vi "CRYO_MASTER_FULL_RUN4_dev2.vi"() -> ()   [LabVIEW 2017]
uses:
  LSI218Data.lvclass
  LSI336Data.lvclass
  USBData.lvclass
  6240AData.lvclass
  DMMsData.lvclass
  LMData.lvclass
  <vilib>/DAQmx/miscellaneous.llb/DAQmx Fill In Error Info.vi
  <vilib>/DAQmx/create/channels.llb/DAQmx Create Channel (DO-Digital Output).vi
  <vilib>/DAQmx/create/channels.llb/DAQmx Create Channel (AO-Voltage-Basic).vi
  <vilib>/express/express arith-compare/Formula/XNode/ExpressFormulaBlockNode.xnode
  <vilib>/Analysis/NI_AALBase.lvlib
  istr.lib/Agilent 33XXX Series/Agilent 33XXX Series.lvlib
panel:
  out "Error Out (AZDAX status)":errorcluster
  in  "Automatic \nScreenshots?":bool=TRUE
  in  "Frontpanel screenshots":bool
  in  "Screenshots interval":i64=3605
  in  "Record interval":i64=20
  out "Cycle #":u32=2
  in  "Measurement Interval (s)":dbl=1.0
  in  "Stop Button":bool
  in  "?":T1(tab)=enum."VALVE/HEATER CTRL"
  out "RUN Identifier":string="20210323_164300_RUNIV"
  in  "Base Path (screenshots)":path=path "C:/LabVIEW/DATA/Google/TUCAN Experiments/KEK_cryotests_2019-2020/data/screenshots"
  out "error out (USB6210/6218 AOUT)":errorcluster
  in  "AOUT Labels":string[](array[string])=["PWR400H_I", "PMC183A_I"]
  in  "AOUT assignment":tag[](array[tag])=["Dev1/ao0", "Dev1/ao1"]
  out "AO task out":refnum<k21>="20210323_164300_RUNIV_AO"
  in  "Analog Out ON?":bool=TRUE
  in  "DOUT6218 Labels":string[](array[string])=["D_V1_NO", "D_V2_NC", "D_CV1", "D_H1", "D_HOME", "D_STOP", "D_M0", "D_M1"]
  in  "InstName (USB6218)":string="USB6218"
  in  "USB6218 Config":T2(array[cluster])=[{"Label"="F_1", "FileFormat"="%5.5f", "Active?"=TRUE, "Physical CH"="Dev1/ai0", " terminal\n type"=10083, "ConversionType"={"Type"=enum."SimpleProp", "ConversionParameters"=[0.0, 5.0, 0.0, 500.0]}, "VoltageLimits"=[0.0, 5.0]}, {"Label"="F_2", "FileFormat"="%5.5f", "Active?"=TRUE, "Physical CH"="Dev1/ai1", " terminal\n type"=10083, "ConversionType"={"Type"=enum."SimpleProp", "ConversionParameters"=[0.0, 5.0, 0.0, 200.0]}, "VoltageLimits"=[0.0, 5.0]}, {"Label"="F_3", "FileFormat"="%5.5f", "Active?"=TRUE, "Physical CH"="Dev1/ai2", " terminal\n type"=10083, "ConversionType"={"Type"=enum."SimpleProp", "ConversionParameters"=[0.0, 5.0, 0.0, 200.0]}, "VoltageLimits"=[0.0, 5.0]}, {"Label"="F_4", "FileFormat"="%5.5f", "Active?"=TRUE, "Physical CH"="Dev1/ai3", " terminal\n type"=10083, "ConversionType"={"Type"=enum."SimpleProp", "ConversionParameters"=[0.0, 5.0, 0.0, 500.0]}, "VoltageLimits"=[0.0, 5.0]}, {"Label"="F_5", "FileFormat"="%5.5f", "Active?"=TRUE, "Physical CH"="Dev1/ai4", " terminal\n type"=10083, "ConversionType"={"Type"=enum."SimpleProp", "ConversionParameters"=[0.0, 5.0, 0.0, 500.0]}, "VoltageLimits"=[0.0, 5.0]}, {"Label"="I_CV", "FileFormat"="%3.5f", "Active?"=TRUE, "Physical CH"="Dev1/ai5", " terminal\n type"=10083, "ConversionType"={"Type"=enum."Raw", "ConversionParameters"=[0.0, 0.0, 0.0, 0.0]}, "VoltageLimits"=[0.0, 10.0]}, {"Label"="CV1_answer", "FileFormat"="%3.5f", "Active?"=TRUE, "Physical CH"="Dev1/ai6", " terminal\n type"=10083, "ConversionType"={"Type"=enum."SimpleProp", "ConversionParameters"=[1.0, 5.0, 0.0, 100.0]}, "VoltageLimits"=[0.0, 5.0]}, {"Label"="P_Dewar", "FileFormat"="%5.5e", "Active?"=TRUE, "Physical CH"="Dev1/ai7", " terminal\n type"=10083, "ConversionType"={"Type"=enum."SimpleProp", "ConversionParameters"=[1.0, 5.0, 0.0, 200000.0]}, "VoltageLimits"=[0.0, 5.0]}, {"Label"="L_Dewar", "FileFormat"="%5.5f", "Active?"=TRUE, "Physical CH"="Dev1/ai8", " terminal\n type"=10083, "ConversionType"={"Type"=enum."SimpleProp", "ConversionParameters"=[0.0, 10.0, 0.0, 100.0]}, "VoltageLimits"=[0.0, 10.0]}] {"terminal\n type" items=["Default"=-1, "RSE"=10083, "NRSE"=10078, "Differential"=10106, "Pseudodifferential"=12529]}
  out "error out (USB6218)":errorcluster
  out "error out (USB6210/6218 DOUT)":errorcluster
  out "DOUT task out":refnum<k21>="20210323_164301_DO"
  in  "DOUT Physical CH":tag[](array[tag])=["Dev1/port1/line0", "Dev1/port1/line1", "Dev1/port1/line2", "Dev1/port1/line3", "Dev1/port1/line4", "Dev1/port1/line5", "Dev1/port1/line6", "Dev1/port1/line7"]
  in  "Digital Out ON?":bool=TRUE
  in  "USB6210 Config":T2(array[cluster])=[{"Label"="P_ins", "FileFormat"="%5.5e", "Active?"=TRUE, "Physical CH"="Dev2/ai0", " terminal\n type"=10083, "ConversionType"={"Type"=enum."CC-10_LOG", "ConversionParameters"=[0.5, 9.0, 0.0, 1.0]}, "VoltageLimits"=[0.0, 10.0]}, {"Label"="P_4Kres", "FileFormat"="%5.5e", "Active?"=TRUE, "Physical CH"="Dev2/ai1", " terminal\n type"=10083, "ConversionType"={"Type"=enum."SimpleProp", "ConversionParameters"=[1.0, 5.0, 0.0, 200000.0]}, "VoltageLimits"=[0.0, 5.0]}, {"Label"="P_3HeIN", "FileFormat"="%5.5e", "Active?"=TRUE, "Physical CH"="Dev2/ai2", " terminal\n type"=10083, "ConversionType"={"Type"=enum."SimpleProp", "ConversionParameters"=[1.0, 5.0, 0.0, 200000.0]}, "VoltageLimits"=[0.0, 5.0]}, {"Label"="P_SldRTN", "FileFormat"="%5.5e", "Active?"=TRUE, "Physical CH"="Dev2/ai3", " terminal\n type"=10083, "ConversionType"={"Type"=enum."SimpleProp", "ConversionParameters"=[1.0, 5.0, 0.0, 200000.0]}, "VoltageLimits"=[0.0, 5.0]}, {"Label"="P_3Hepot", "FileFormat"="%5.5e", "Active?"=TRUE, "Physical CH"="Dev2/ai4", " terminal\n type"=10083, "ConversionType"={"Type"=enum."SimpleProp", "ConversionParameters"=[0.0, 10.0, 0.0, 133320.0]}, "VoltageLimits"=[0.0, 10.0]}, {"Label"="P_1Kpot", "FileFormat"="%5.5e", "Active?"=TRUE, "Physical CH"="Dev2/ai5", " terminal\n type"=10083, "ConversionType"={"Type"=enum."SimpleProp", "ConversionParameters"=[0.0, 10.0, 0.0, 133320.0]}, "VoltageLimits"=[0.0, 10.0]}, {"Label"="P_Dewar(old)", "FileFormat"="%5.5e", "Active?"=FALSE, "Physical CH"="Dev2/ai6", " terminal\n type"=10083, "ConversionType"={"Type"=enum."SimpleProp", "ConversionParameters"=[1.0, 5.0, 0.0, 200000.0]}, "VoltageLimits"=[0.0, 5.0]}, {"Label"="DP_HEX4", "FileFormat"="%5.5e", "Active?"=TRUE, "Physical CH"="Dev2/ai7", " terminal\n type"=10083, "ConversionType"={"Type"=enum."SimpleProp", "ConversionParameters"=[1.0, 5.0, 0.0, 1000.0]}, "VoltageLimits"=[0.0, 5.0]}, {"Label"="DP_HEX5", "FileFormat"="%5.5e", "Active?"=TRUE, "Physical CH"="Dev2/ai8", " terminal\n type"=10083, "ConversionType"={"Type"=enum."SimpleProp", "ConversionParameters"=[1.0, 5.0, 0.0, 1000.0]}, "VoltageLimits"=[0.0, 5.0]}, {"Label"="L1(old)", "FileFormat"="%5.5f", "Active?"=TRUE, "Physical CH"="Dev2/ai9", " terminal\n type"=10083, "ConversionType"={"Type"=enum."SimpleProp", "ConversionParameters"=[0.0, 10.0, 0.0, 100.0]}, "VoltageLimits"=[0.0, 10.0]}, {"Label"="L2-1", "FileFormat"="%5.5f", "Active?"=TRUE, "Physical CH"="Dev2/ai10", " terminal\n type"=10083, "ConversionType"={"Type"=enum."SimpleProp", "ConversionParameters"=[0.0, 10.0, 0.0, 100.0]}, "VoltageLimits"=[0.0, 10.0]}, {"Label"="L1", "FileFormat"="%5.5f", "Active?"=TRUE, "Physical CH"="Dev2/ai11", " terminal\n type"=10083, "ConversionType"={"Type"=enum."SimpleProp", "ConversionParameters"=[0.0, 10.0, 0.0, 100.0]}, "VoltageLimits"=[0.0, 10.0]}, {"Label"="L3", "FileFormat"="%5.5f", "Active?"=TRUE, "Physical CH"="Dev2/ai12", " terminal\n type"=10083, "ConversionType"={"Type"=enum."SimpleProp", "ConversionParameters"=[0.0, 10.0, 0.0, 100.0]}, "VoltageLimits"=[0.0, 10.0]}, {"Label"="P_HEX7OUT", "FileFormat"="%5.5e", "Active?"=TRUE, "Physical CH"="Dev2/ai13", " terminal\n type"=10083, "ConversionType"={"Type"=enum."SimpleProp", "ConversionParameters"=[1.0, 5.0, 0.0, 200000.0]}, "VoltageLimits"=[0.0, 5.0]}, {"Label"="P_IP", "FileFormat"="%5.5e", "Active?"=TRUE, "Physical CH"="Dev2/ai14", " terminal\n type"=10083, "ConversionType"={"Type"=enum."CC-10_LOG", "ConversionParameters"=[0.5, 9.0, 0.0, 1.0]}, "VoltageLimits"=[0.0, 10.0]}, {"Label"="V_H1", "FileFormat"="%3.5f", "Active?"=TRUE, "Physical CH"="Dev2/ai15", " terminal\n type"=10083, "ConversionType"={"Type"=enum."Raw", "ConversionParameters"=[0.0, 1.0, 0.0, 1.0]}, "VoltageLimits"=[0.0, 10.0]}] {"terminal\n type" items=["Default"=-1, "RSE"=10083, "NRSE"=10078, "Differential"=10106, "Pseudodifferential"=12529]}
  in  "RUN label":string="RUNIV"
  in  "Base Path":path=path "C:/LabVIEW/DATA/RUN_4"
  in  "InstName (USB6210)":string="USB6210"
  out "error out (USB6210)":errorcluster
  out "File Refn USB AO":refnum<file>
  out "File Refn USB DO":refnum<file>
  out "File ref AZD-AX status":refnum<file>
  in  "LM measurement interval (>0)":i64=10
  in  "Active? (HP34401 LM)":bool=TRUE
  in  "Labels (HP34401 LM)":string[](array[string])=["R_L2-2", "L2-2"]
  in  "FileFormat (HP34401 LM)":string[](array[string])=["%.4f", "%.4f"]
  in  "VISA (HP34401 LM)":refnum<visa-resource-name>="GPIB0::24::INSTR"
  in  "LevelCalibration (R0, R1, L0, L1)":dbl[](array[numeric])=[186.541, 0.0, 0.0, 100.0]
  in  "InstName (HP34401 LM)":string="HP34401LM"
  out "error out (LSI336)":errorcluster
  in  "InstName (LSI336)":string="LSI336"
  in  "FileFormat (336)":string="%4.4f"
  in  "LSI336Settings(X,Y)":T3(array[cluster])=[{"LSIName"="LSi336X", "Labels"=["T1K3-1", "T1K3-2", "T3He5", "T3He8"], "SensorLocations"=[enum."T1K3-1", enum."T1K3-2", enum."T3He5", enum."T3He8"], "Active?"=TRUE, "VISA res. name"="COM15_LSI336Y"}, {"LSIName"="LSi336Y", "Labels"=["T3He6-1", "T3He6-2", "T3He7-1", "T3He7-2"], "SensorLocations"=[enum."T3He6-1", enum."T3He6-2", enum."T3He7-1", enum."T3He7-2"], "Active?"=TRUE, "VISA res. name"="COM20_LSI336X"}]
  in  "FileFormat (218)":string="%4.4f"
  in  "InstName (LSI218)":string="LSI218"
  in  "LSI218Settings(A-F)":T3(array[cluster])=[{"LSIName"="LSI218A", "Labels"=["T3He10", "T3He1-1", "TTH3", "TTH4", "TTH1", "TTH2", "T4He1", "T1K1"], "SensorLocations"=[enum."T3He10", enum."T3He1-1", enum."TTH3", enum."TTH4", enum."TTH1", enum."TTH2", enum."T4He1", enum."T1K1"], "Active?"=TRUE, "VISA res. name"="GPIB0::7::INSTR"}, {"LSIName"="LSI218B", "Labels"=["N.C.", "N.C.", "N.C.", "N.C.", "T3He2-1", "T3He2-2", "T3He3", "T3He1-4"], "SensorLocations"=[enum."N.C.", enum."N.C.", enum."N.C.", enum."N.C.", enum."T3He2-1", enum."T3He2-2", enum."T3He3", enum."T3He1-4"], "Active?"=TRUE, "VISA res. name"="GPIB0::4::INSTR"}, {"LSIName"="LSI218C", "Labels"=["T4He3-1", "T4He3-2", "T4He3-3", "T4He3-4", "T4He2-1", "T4He2-2", "T4He4", "T4He5"], "SensorLocations"=[enum."T4He3-1", enum."T4He3-2", enum."T4He3-3", enum."T4He3-4", enum."T4He2-1", enum."T4He2-2", enum."T4He4", enum."T4He5"], "Active?"=TRUE, "VISA res. name"="GPIB0::3::INSTR"}, {"LSIName"="LSI218D", "Labels"=["T4He6", "T4He9", "T3He1-2", "T3He1-3", "T4He7", "T4He8", "T4He10", "T1K6"], "SensorLocations"=[enum."T4He6", enum."T4He9", enum."T3He1-2", enum."T3He1-3", enum."T4He7", enum."T4He8", enum."T4He10", enum."T1K6"], "Active?"=TRUE, "VISA res. name"="GPIB0::5::INSTR"}, {"LSIName"="LSI218E", "Labels"=["TIP1", "N.C.", "TIP2", "N.C.", "TIP3", "TIP4", "TIP5", "N.C."], "SensorLocations"=[enum."TIP1", enum."N.C.", enum."TIP2", enum."N.C.", enum."TIP3", enum."TIP4", enum."TIP5", enum."N.C."], "Active?"=TRUE, "VISA res. name"="GPIB0::11::INSTR"}, {"LSIName"="LSI218F", "Labels"=["T1K2", "T1K4", "T1K5", "T3He4", "T3He9", "TIP6", "N.C.", "N.C."], "SensorLocations"=[enum."T1K2", enum."T1K4", enum."T1K5", enum."T3He4", enum."T3He9", enum."TIP6", enum."N.C.", enum."N.C."], "Active?"=TRUE, "VISA res. name"="GPIB0::8::INSTR"}]
  out "error out (LSI218)":errorcluster
  out "RUN Identifier 2":string="20210323_164300_RUNIV" caption="RUN Identifier"
  out "error out (HP34401 LM)":errorcluster
  out "Graph 3":T4(graph)=[{"TimeArray"=[timestamp(3699330182.9543066 s since 1904-01-01), timestamp(3699330183.99275 s since 1904-01-01)], "DataArray"=[2.229000287561577, 1.8476051977193715]}, {"TimeArray"=[timestamp(3699330182.9543066 s since 1904-01-01), timestamp(3699330183.99275 s since 1904-01-01)], "DataArray"=[6.5651805759101745, 6.559919954343005]}, {"TimeArray"=[timestamp(3699330182.9543066 s since 1904-01-01), timestamp(3699330183.99275 s since 1904-01-01)], "DataArray"=[0.6141023076914145, 0.5720173311260397]}, {"TimeArray"=[timestamp(3699330182.9543066 s since 1904-01-01), timestamp(3699330183.99275 s since 1904-01-01)], "DataArray"=[-0.3684318274206404, -0.35856816207260195]}, {"TimeArray"=[timestamp(3699330182.9543066 s since 1904-01-01), timestamp(3699330183.99275 s since 1904-01-01)], "DataArray"=[23.39313821847484, 23.485199087329573]}, {"TimeArray"=[timestamp(3699330182.9543066 s since 1904-01-01), timestamp(3699330183.99275 s since 1904-01-01)], "DataArray"=[-0.0038120682713622734, -0.00019463958134809388]}] caption="XY Graph"
  out "Graph 1":T4(graph)=[{"TimeArray"=[timestamp(3699330182.9503174 s since 1904-01-01), timestamp(3699330183.988761 s since 1904-01-01)], "DataArray"=[0.0001467822274904493, 0.00014331210383532943]}, {"TimeArray"=[timestamp(3699330182.9503174 s since 1904-01-01), timestamp(3699330183.988761 s since 1904-01-01)], "DataArray"=[103386.1520739023, 103419.04061540413]}, {"TimeArray"=[timestamp(3699330182.9503174 s since 1904-01-01), timestamp(3699330183.988761 s since 1904-01-01)], "DataArray"=[102917.4903816534, 102917.49038025808]}, {"TimeArray"=[timestamp(3699330182.9503174 s since 1904-01-01), timestamp(3699330183.988761 s since 1904-01-01)], "DataArray"=[102784.29179605731, 102876.37970352173]}, {"TimeArray"=[timestamp(3699330182.9503174 s since 1904-01-01), timestamp(3699330183.988761 s since 1904-01-01)], "DataArray"=[102285.6157171335, 102299.64398756107]}, {"TimeArray"=[timestamp(3699330182.9503174 s since 1904-01-01), timestamp(3699330183.988761 s since 1904-01-01)], "DataArray"=[102778.35876990847, 102783.61937258235]}, {"TimeArray"=[timestamp(3699330182.9503174 s since 1904-01-01), timestamp(3699330183.988761 s since 1904-01-01)], "DataArray"=[0.0, 0.0]}, {"TimeArray"=[timestamp(3699330182.9503174 s since 1904-01-01), timestamp(3699330183.988761 s since 1904-01-01)], "DataArray"=[102831.98017524344, 102960.24547937719]}, {"TimeArray"=[timestamp(3699330182.9503174 s since 1904-01-01), timestamp(3699330183.988761 s since 1904-01-01)], "DataArray"=[6.658695577811817e-05, 6.903046749339257e-05]}, {"TimeArray"=[timestamp(3699330182.9543066 s since 1904-01-01), timestamp(3699330183.99275 s since 1904-01-01)], "DataArray"=[133922.54729625225, 134754.38150670484]}] caption="XY Graph"
  in  "FIle suffix 4":string="Graph4_noise"
  in  "Take Screenshot! 4":bool
  in  "Take Screenshot! 3":bool
  in  "Take Screenshot! 2":bool
  in  "Take Screenshot! 1":bool
  in  "FIle suffix 3":string="Graph3_noise"
  in  "FIle suffix 2":string="Graph2_build"
  in  "FIle suffix 1":string="Graph1_noise"
  in  "log/linear 2":bool
  in  "Tab Control 2":T5(tab)=enum."Temperature (3)"
  in  "Plot selecter (USB6210)\n    1      2     3     4":bool[][](array[boolean])=[[TRUE, FALSE, FALSE, FALSE], [TRUE, FALSE, FALSE, FALSE], [TRUE, FALSE, FALSE, FALSE], [TRUE, FALSE, FALSE, FALSE], [TRUE, FALSE, FALSE, FALSE], [TRUE, FALSE, FALSE, FALSE], [TRUE, FALSE, FALSE, FALSE], [FALSE, FALSE, FALSE, FALSE], [FALSE, FALSE, FALSE, FALSE], [FALSE, TRUE, FALSE, FALSE], [FALSE, TRUE, FALSE, FALSE], [FALSE, TRUE, FALSE, FALSE], [FALSE, TRUE, FALSE, FALSE], [TRUE, FALSE, FALSE, FALSE], [TRUE, FALSE, FALSE, FALSE], [FALSE, FALSE, FALSE, FALSE]]
  out "All Labels (USB6210)":string[](array[string])=["P_ins", "P_4Kres", "P_3HeIN", "P_SldRTN", "P_3Hepot", "P_1Kpot", "P_Dewar(old)", "DP_HEX4", "DP_HEX5", "L1(old)", "L2-1", "L1", "L3", "P_HEX7OUT", "P_IP", "V_H1"]
  out "Last Data \n(USB6210)":dbl[](array[numeric])=[0.00014331210383532943, 103419.04061540413, 102917.49038025808, 102876.37970352173, 102299.64398756107, 102783.61937258235, 0.0, 0.009359860621893645, 6.307429085038785, 9.980910378649359, 0.03893370650245273, 0.17703499365619763, 31.866703704233657, 102960.24547937719, 6.903046749339257e-05, 5.354612085872782] format="%#_6e"
  out "Time of Last Measurement (USB6210)":timestamp=timestamp(3699330183.988761 s since 1904-01-01)
  out "USB6210 Status":T6(ring)=enum."Ready"
  out "Last Vol\n(USB6210)":dbl[](array[numeric])=[5.578141435767079, 3.0683808123080825, 3.0583498076051616, 3.0575275940704345, 7.673240623129393, 7.709542407184395, 0.0, 1.0000374394424876, 1.0252297163401551, 0.9980910378649359, 0.003893370650245273, 0.01770349936561976, 3.1866703704233657, 3.0592049095875438, 5.419520407280226, 5.354612085872782] format="%_5f"
  out "Labels (HP34401 LM) 2":string[](array[string])=["R_L2-2", "L2-2"]
  out "LastData (HP34401 LM)":dbl[](array[numeric])
  in  "Plot selecter (HP34401A)\n    1      2     3     4":bool[][](array[boolean])=[[FALSE, TRUE, FALSE, FALSE], [FALSE, TRUE, FALSE, FALSE], [TRUE, FALSE, FALSE, FALSE], [TRUE, FALSE, FALSE, FALSE], [TRUE, FALSE, FALSE, FALSE], [TRUE, FALSE, FALSE, FALSE], [TRUE, FALSE, FALSE, FALSE], [FALSE, TRUE, FALSE, FALSE], [FALSE, TRUE, FALSE, FALSE], [FALSE, TRUE, FALSE, FALSE], [FALSE, TRUE, FALSE, FALSE], [FALSE, TRUE, FALSE, FALSE], [FALSE, TRUE, FALSE, FALSE], [TRUE, FALSE, FALSE, FALSE], [TRUE, FALSE, FALSE, FALSE], [FALSE, FALSE, FALSE, FALSE]]
  out "Time of Last Measurement (USB6218)":timestamp=timestamp(3699330183.99275 s since 1904-01-01)
  out "USB6218 Status":T6(ring)=enum."Ready"
  out "Last Vol \n(USB6218)":dbl[](array[numeric])=[0.018476051977193715, 0.16399799885857513, 0.014300433278150993, -0.0035856816207260195, 0.23485199087329572, -0.00019463958134809388, 0.003022974846202206, 3.695087630134097, 1.4212571383113937] format="%_5f"
  out "Last Data \n(USB6218)":dbl[](array[numeric])=[1.8476051977193715, 6.559919954343005, 0.5720173311260397, -0.35856816207260195, 23.485199087329573, -0.00019463958134809388, -24.924425628844947, 134754.38150670484, 14.212571383113936] format="%#_6e"
  out "All Labels (USB6218)":string[](array[string])=["F_1", "F_2", "F_3", "F_4", "F_5", "I_CV", "CV1_answer", "P_Dewar", "L_Dewar"]
  in  "Plot selecter (USB6218)\n    1      2     3     4":bool[][](array[boolean])=[[FALSE, FALSE, TRUE, FALSE], [FALSE, FALSE, TRUE, FALSE], [FALSE, FALSE, TRUE, FALSE], [FALSE, FALSE, TRUE, FALSE], [FALSE, FALSE, TRUE, FALSE], [FALSE, FALSE, TRUE, FALSE], [FALSE, FALSE, FALSE, FALSE], [TRUE, FALSE, FALSE, FALSE], [FALSE, TRUE, FALSE, FALSE], [FALSE, FALSE, FALSE, TRUE], [FALSE, FALSE, FALSE, TRUE], [FALSE, FALSE, FALSE, TRUE], [FALSE, FALSE, FALSE, TRUE], [FALSE, FALSE, FALSE, FALSE], [FALSE, FALSE, FALSE, FALSE], [FALSE, FALSE, FALSE, FALSE]]
  out "Time of Last Measurement (LSI218)":timestamp=timestamp(3699330183.988761 s since 1904-01-01)
  out "LSI218 Status":T7(ring)=enum."Measuring"
  out "Last Data \nLSI218 (1)":dbl[](array[numeric])=[238.58, 276.68, 145.02, 218.62, 54.478, 85.05, 4.442, 4.661, 30.0, 0.0, 0.0, 0.0, 56.991, 53.134, 5.055, 271.93, 282.27, 282.4, 279.79, 279.75, 34.466, 36.266, 28.98, 55.8]
  out "Labels LSI218 (1)":string[](array[string])=["T3He10", "T3He1-1", "TTH3", "TTH4", "TTH1", "TTH2", "T4He1", "T1K1", "N.C.", "N.C.", "N.C.", "N.C.", "T3He2-1", "T3He2-2", "T3He3", "T3He1-4", "T4He3-1", "T4He3-2", "T4He3-3", "T4He3-4", "T4He2-1", "T4He2-2", "T4He4", "T4He5"]
  in  "Plot selecter LSI218(1)\n    1      2     3     4":bool[][](array[boolean])=[[FALSE, FALSE, FALSE, TRUE], [FALSE, FALSE, FALSE, TRUE], [FALSE, FALSE, FALSE, TRUE], [FALSE, FALSE, FALSE, TRUE], [FALSE, FALSE, FALSE, TRUE], [FALSE, FALSE, FALSE, TRUE], [FALSE, FALSE, FALSE, TRUE], [FALSE, FALSE, FALSE, TRUE], [FALSE, FALSE, FALSE, FALSE], [FALSE, FALSE, FALSE, FALSE], [FALSE, FALSE, FALSE, FALSE], [FALSE, FALSE, FALSE, FALSE], [FALSE, FALSE, FALSE, TRUE], [FALSE, FALSE, FALSE, TRUE], [FALSE, FALSE, FALSE, TRUE], [FALSE, FALSE, FALSE, TRUE], [FALSE, FALSE, FALSE, TRUE], [FALSE, FALSE, FALSE, TRUE], [FALSE, FALSE, FALSE, TRUE], [FALSE, FALSE, FALSE, TRUE], [FALSE, FALSE, FALSE, TRUE], [FALSE, FALSE, FALSE, TRUE], [FALSE, FALSE, FALSE, TRUE], [FALSE, FALSE, FALSE, TRUE]]
  out "Active?\n (1)":bool[](array[boolean])=[TRUE, TRUE, TRUE, TRUE, TRUE, TRUE, TRUE, TRUE, TRUE, TRUE, TRUE, TRUE, TRUE, TRUE, TRUE, TRUE, TRUE, TRUE, TRUE, TRUE, TRUE, TRUE, TRUE, TRUE]
  out "Labels LSI218 (2)":string[](array[string])=["T4He6", "T4He9", "T3He1-2", "T3He1-3", "T4He7", "T4He8", "T4He10", "T1K6", "TIP1", "N.C.", "TIP2", "N.C.", "TIP3", "TIP4", "TIP5", "N.C.", "T1K2", "T1K4", "T1K5", "T3He4", "T3He9", "TIP6", "N.C.", "N.C."]
  out "Active?\n(2)":bool[](array[boolean])=[TRUE, TRUE, TRUE, TRUE, TRUE, TRUE, TRUE, TRUE, TRUE, TRUE, TRUE, TRUE, TRUE, TRUE, TRUE, TRUE, TRUE, TRUE, TRUE, TRUE, TRUE, TRUE, TRUE, TRUE]
  out "Last Data \nLSI218 (2)":dbl[](array[numeric])=[62.643, 171.21, 276.82, 272.08, 143.05, 161.51, 221.22, 243.0, 252.76, 0.0, 130.11, 688.49, 83.786, 70.623, 114.8, 688.58, 14.054, 11.753, 10.988, 12.938, 10.918, 110.83, 0.433, 0.0]
  in  "Plot selecter LSI218(2)\n    1      2     3     4":bool[][](array[boolean])=[[FALSE, FALSE, FALSE, TRUE], [FALSE, FALSE, FALSE, TRUE], [FALSE, FALSE, FALSE, FALSE], [FALSE, FALSE, FALSE, FALSE], [FALSE, FALSE, FALSE, FALSE], [FALSE, FALSE, FALSE, FALSE], [FALSE, FALSE, FALSE, FALSE], [FALSE, FALSE, FALSE, FALSE], [FALSE, FALSE, FALSE, FALSE], [FALSE, FALSE, FALSE, FALSE], [FALSE, FALSE, FALSE, FALSE], [FALSE, FALSE, FALSE, FALSE], [FALSE, FALSE, FALSE, FALSE], [FALSE, FALSE, FALSE, FALSE], [FALSE, FALSE, FALSE, FALSE], [FALSE, FALSE, FALSE, FALSE], [FALSE, FALSE, FALSE, TRUE], [FALSE, FALSE, FALSE, TRUE], [FALSE, FALSE, FALSE, TRUE], [FALSE, FALSE, FALSE, TRUE], [FALSE, FALSE, FALSE, TRUE], [FALSE, FALSE, FALSE, FALSE], [FALSE, FALSE, FALSE, FALSE], [FALSE, FALSE, FALSE, FALSE]]
  in  "Plot selecter LSI336 \n     1      2     3     4":bool[][](array[boolean])=[[FALSE, FALSE, FALSE, TRUE], [FALSE, FALSE, FALSE, TRUE], [FALSE, FALSE, FALSE, TRUE], [FALSE, FALSE, FALSE, TRUE], [FALSE, FALSE, FALSE, TRUE], [FALSE, FALSE, FALSE, TRUE], [FALSE, FALSE, FALSE, TRUE], [FALSE, FALSE, FALSE, TRUE]]
  out "Time of Last Measurement (LSI336)":timestamp=timestamp(3699330183.988761 s since 1904-01-01)
  out "Last Data \nLSI336":dbl[](array[numeric])=[12.0158, 12.046, 13.2196, 12.3577, 19.0262, 19.857, 21.3351, 16.3982]
  out "Active?\n(LSI336)":bool[](array[boolean])=[TRUE, TRUE, TRUE, TRUE, TRUE, TRUE, TRUE, TRUE]
  out "Labels LSI336":string[](array[string])=["T1K3-1", "T1K3-2", "T3He5", "T3He8", "T3He6-1", "T3He6-2", "T3He7-1", "T3He7-2"]
  out "LSI336 Status":T7(ring)=enum."Measuring"
  in  "log/linear 1":bool
  out "Graph 2":T4(graph)=[{"TimeArray"=[timestamp(3699330182.9503174 s since 1904-01-01), timestamp(3699330183.988761 s since 1904-01-01)], "DataArray"=[10.022340765034453, 9.980910378649359]}, {"TimeArray"=[timestamp(3699330182.9503174 s since 1904-01-01), timestamp(3699330183.988761 s since 1904-01-01)], "DataArray"=[0.028411703634074498, 0.03893370650245273]}, {"TimeArray"=[timestamp(3699330182.9503174 s since 1904-01-01), timestamp(3699330183.988761 s since 1904-01-01)], "DataArray"=[0.17703499366301226, 0.17703499365619763]}, {"TimeArray"=[timestamp(3699330182.9503174 s since 1904-01-01), timestamp(3699330183.988761 s since 1904-01-01)], "DataArray"=[31.87854099600237, 31.866703704233657]}, {"TimeArray"=[timestamp(3699330182.9543066 s since 1904-01-01), timestamp(3699330183.99275 s since 1904-01-01)], "DataArray"=[14.198759390010572, 14.212571383113936]}, {"TimeArray"=[], "DataArray"=[]}, {"TimeArray"=[], "DataArray"=[]}] caption="XY Graph"
  out "Graph 4":T4(graph)=[{"TimeArray"=[timestamp(3699330182.9493194 s since 1904-01-01), timestamp(3699330183.988761 s since 1904-01-01)], "DataArray"=[238.58, 238.58]}, {"TimeArray"=[timestamp(3699330182.9493194 s since 1904-01-01), timestamp(3699330183.988761 s since 1904-01-01)], "DataArray"=[276.68, 276.68]}, {"TimeArray"=[timestamp(3699330182.9493194 s since 1904-01-01), timestamp(3699330183.988761 s since 1904-01-01)], "DataArray"=[145.0, 145.02]}, {"TimeArray"=[timestamp(3699330182.9493194 s since 1904-01-01), timestamp(3699330183.988761 s since 1904-01-01)], "DataArray"=[218.62, 218.62]}, {"TimeArray"=[timestamp(3699330182.9493194 s since 1904-01-01), timestamp(3699330183.988761 s since 1904-01-01)], "DataArray"=[54.48, 54.478]}, {"TimeArray"=[timestamp(3699330182.9493194 s since 1904-01-01), timestamp(3699330183.988761 s since 1904-01-01)], "DataArray"=[85.051, 85.05]}, {"TimeArray"=[timestamp(3699330182.9493194 s since 1904-01-01), timestamp(3699330183.988761 s since 1904-01-01)], "DataArray"=[4.447, 4.442]}, {"TimeArray"=[timestamp(3699330182.9493194 s since 1904-01-01), timestamp(3699330183.988761 s since 1904-01-01)], "DataArray"=[4.668, 4.661]}, {"TimeArray"=[timestamp(3699330182.9493194 s since 1904-01-01), timestamp(3699330183.988761 s since 1904-01-01)], "DataArray"=[56.993, 56.991]}, {"TimeArray"=[timestamp(3699330182.9493194 s since 1904-01-01), timestamp(3699330183.988761 s since 1904-01-01)], "DataArray"=[53.128, 53.134]}, {"TimeArray"=[timestamp(3699330182.9493194 s since 1904-01-01), timestamp(3699330183.988761 s since 1904-01-01)], "DataArray"=[5.052, 5.055]}, {"TimeArray"=[timestamp(3699330182.9493194 s since 1904-01-01), timestamp(3699330183.988761 s since 1904-01-01)], "DataArray"=[271.93, 271.93]}, {"TimeArray"=[timestamp(3699330182.9493194 s since 1904-01-01), timestamp(3699330183.988761 s since 1904-01-01)], "DataArray"=[282.27, 282.27]}, {"TimeArray"=[timestamp(3699330182.9493194 s since 1904-01-01), timestamp(3699330183.988761 s since 1904-01-01)], "DataArray"=[282.4, 282.4]}, {"TimeArray"=[timestamp(3699330182.9493194 s since 1904-01-01), timestamp(3699330183.988761 s since 1904-01-01)], "DataArray"=[279.78, 279.79]}, {"TimeArray"=[timestamp(3699330182.9493194 s since 1904-01-01), timestamp(3699330183.988761 s since 1904-01-01)], "DataArray"=[279.75, 279.75]}, {"TimeArray"=[timestamp(3699330182.9493194 s since 1904-01-01), timestamp(3699330183.988761 s since 1904-01-01)], "DataArray"=[34.464, 34.466]}, {"TimeArray"=[timestamp(3699330182.9493194 s since 1904-01-01), timestamp(3699330183.988761 s since 1904-01-01)], "DataArray"=[36.266, 36.266]}, {"TimeArray"=[timestamp(3699330182.9493194 s since 1904-01-01), timestamp(3699330183.988761 s since 1904-01-01)], "DataArray"=[28.983, 28.98]}, {"TimeArray"=[timestamp(3699330182.9493194 s since 1904-01-01), timestamp(3699330183.988761 s since 1904-01-01)], "DataArray"=[55.799, 55.8]}, {"TimeArray"=[timestamp(3699330182.9493194 s since 1904-01-01), timestamp(3699330183.988761 s since 1904-01-01)], "DataArray"=[62.642, 62.643]}, {"TimeArray"=[timestamp(3699330182.9493194 s since 1904-01-01), timestamp(3699330183.988761 s since 1904-01-01)], "DataArray"=[171.21, 171.21]}, {"TimeArray"=[timestamp(3699330182.9493194 s since 1904-01-01), timestamp(3699330183.988761 s since 1904-01-01)], "DataArray"=[330.07, 14.054]}, {"TimeArray"=[timestamp(3699330182.9493194 s since 1904-01-01), timestamp(3699330183.988761 s since 1904-01-01)], "DataArray"=[11.658, 11.753]}, {"TimeArray"=[timestamp(3699330182.9493194 s since 1904-01-01), timestamp(3699330183.988761 s since 1904-01-01)], "DataArray"=[10.992, 10.988]}, {"TimeArray"=[timestamp(3699330182.9493194 s since 1904-01-01), timestamp(3699330183.988761 s since 1904-01-01)], "DataArray"=[12.951, 12.938]}, {"TimeArray"=[timestamp(3699330182.9493194 s since 1904-01-01), timestamp(3699330183.988761 s since 1904-01-01)], "DataArray"=[10.898, 10.918]}, {"TimeArray"=[timestamp(3699330182.9493194 s since 1904-01-01), timestamp(3699330183.988761 s since 1904-01-01)], "DataArray"=[12.015, 12.0158]}, {"TimeArray"=[timestamp(3699330182.9493194 s since 1904-01-01), timestamp(3699330183.988761 s since 1904-01-01)], "DataArray"=[12.0443, 12.046]}, {"TimeArray"=[timestamp(3699330182.9493194 s since 1904-01-01), timestamp(3699330183.988761 s since 1904-01-01)], "DataArray"=[13.2176, 13.2196]}, {"TimeArray"=[timestamp(3699330182.9493194 s since 1904-01-01), timestamp(3699330183.988761 s since 1904-01-01)], "DataArray"=[12.3577, 12.3577]}, {"TimeArray"=[timestamp(3699330182.9493194 s since 1904-01-01), timestamp(3699330183.988761 s since 1904-01-01)], "DataArray"=[19.0199, 19.0262]}, {"TimeArray"=[timestamp(3699330182.9493194 s since 1904-01-01), timestamp(3699330183.988761 s since 1904-01-01)], "DataArray"=[19.8429, 19.857]}, {"TimeArray"=[timestamp(3699330182.9493194 s since 1904-01-01), timestamp(3699330183.988761 s since 1904-01-01)], "DataArray"=[21.346, 21.3351]}, {"TimeArray"=[timestamp(3699330182.9493194 s since 1904-01-01), timestamp(3699330183.988761 s since 1904-01-01)], "DataArray"=[16.396, 16.3982]}] caption="XY Graph"
  in  "log/linear 4":bool
  in  "log/linear 3":bool
  out "RUN Identifier 3":string="20210323_164300_RUNIV" caption="RUN Identifier"
  in  "AutoFill Source (P)":T8(ring)=enum."USB6218AI"
  in  "AutoFill Source (L)":T8(ring)
  out "RUN Identifier 4":string="20210323_164300_RUNIV" caption="RUN Identifier"
  out "Fill (false)":bool=TRUE
  in  "Fill state":bool
  out "state 1 (false)":bool=TRUE
  out "state 1":bool
  out "state 2":bool
  out "state 2 (false)":bool=TRUE
  out "Status V2 CTRL":enum16{"Pressurize", "Release"}(ring)=enum."Release"
  out "Status V1 CTRL":enum16{"Pressurize", "Release"}(ring)
  out "Lav (%)":dbl=30.34365086955015 format="%0.2f"
  out "Lstd":dbl=0.17773361622742143 format="%0.2f"
  out "Last N M.A. Levels":dbl[](array[numeric])=[30.20997642107327, 30.208825573733307, 30.21112726841796, 30.201098455866088, 30.197317100320245, 30.217045912709, 30.215730658595675, 30.22247133587181, 30.329993364101796, 30.41285437666867, 30.517745896584714, 30.621650976139335, 30.621322162577258, 30.62395267104293] format="%_5e"
  out "Lstd history":dbl(graph)=0.16113734277944766
  out "Lav history":dbl(graph)=30.314139854110472
  out "Target Index (L)":i32=12
  in  "Auto Fll He L. label":string="L3"
  out "Target Index (P)":i32=7
  in  "Auto Fll Dewar P. label":string="P_Dewar"
  out "He Level":T9(graph)=[{"TimeArray"=[timestamp(3699330022.9537086 s since 1904-01-01), timestamp(3699330023.955344 s since 1904-01-01), timestamp(3699330024.9525824 s since 1904-01-01), timestamp(3699330025.9546447 s since 1904-01-01), timestamp(3699330027.2328625 s since 1904-01-01), timestamp(3699330028.229321 s since 1904-01-01), timestamp(3699330029.2276254 s since 1904-01-01), timestamp(3699330030.2324934 s since 1904-01-01), timestamp(3699330031.232282 s since 1904-01-01), timestamp(3699330032.2356615 s since 1904-01-01), timestamp(3699330033.2346354 s since 1904-01-01), timestamp(3699330034.2382703 s since 1904-01-01), timestamp(3699330035.2374697 s since 1904-01-01), timestamp(3699330036.2392607 s since 1904-01-01)], "Filtered X"=[30.210798454864992, 30.199618794984247, 30.206852692583265, 30.18712388103185, 30.195673032681615, 30.278534044539267, 30.201591676129958, 30.214086590136382, 30.625761145601587, 30.60997809480675, 30.62115775579414, 30.629706908354855, 30.624445891353268, 30.620500128669455]}, {"TimeArray"=[timestamp(3699330022.9537086 s since 1904-01-01), timestamp(3699330023.955344 s since 1904-01-01), timestamp(3699330024.9525824 s since 1904-01-01), timestamp(3699330025.9546447 s since 1904-01-01), timestamp(3699330027.2328625 s since 1904-01-01), timestamp(3699330028.229321 s since 1904-01-01), timestamp(3699330029.2276254 s since 1904-01-01), timestamp(3699330030.2324934 s since 1904-01-01), timestamp(3699330031.232282 s since 1904-01-01), timestamp(3699330032.2356615 s since 1904-01-01), timestamp(3699330033.2346354 s since 1904-01-01), timestamp(3699330034.2382703 s since 1904-01-01), timestamp(3699330035.2374697 s since 1904-01-01), timestamp(3699330036.2392607 s since 1904-01-01)], "Filtered X"=[30.20997642107327, 30.208825573733307, 30.21112726841796, 30.201098455866088, 30.197317100320245, 30.217045912709, 30.215730658595675, 30.22247133587181, 30.329993364101796, 30.41285437666867, 30.517745896584714, 30.621650976139335, 30.621322162577258, 30.62395267104293]}] caption="XY Graph"
  in  "P_safelimit_high (Pa)":dbl=300000.0 format="%_4e"
  in  "P_safelimit_low (Pa)":dbl=100.0 format="%_4e"
  in  "Auto Fill ON?":bool=TRUE
  out "Pstd history":dbl(graph)=112.64721280636759
  out "Pav history":dbl(graph)=134960.75483198816
  in  "Mov. Avg Interval":i64=4
  in  "V2 (N.C.)":bool
  in  "V1 (N.O.)":bool=TRUE
  in  "N for sampling":i64=7
  in  "L_low (%)":dbl=100.0 format="%_3f"
  in  "L_high (%)":dbl=100.0 format="%_3g"
  in  "P_2_low (Pa)":dbl=125000.0 format="%_4e"
  in  "P_1_low (Pa)":dbl=130000.0 format="%_4g"
  in  "P_2_high (Pa)":dbl=130000.0 format="%_4e"
  in  "P_1_high (Pa)":dbl=140000.0 format="%_4e"
  out "Dewar Pressure":T9(graph)=[{"TimeArray"=[timestamp(3699330022.9537086 s since 1904-01-01), timestamp(3699330023.955344 s since 1904-01-01), timestamp(3699330024.9525824 s since 1904-01-01), timestamp(3699330025.9546447 s since 1904-01-01), timestamp(3699330027.2328625 s since 1904-01-01), timestamp(3699330028.229321 s since 1904-01-01), timestamp(3699330029.2276254 s since 1904-01-01), timestamp(3699330030.2324934 s since 1904-01-01), timestamp(3699330031.232282 s since 1904-01-01), timestamp(3699330032.2356615 s since 1904-01-01), timestamp(3699330033.2346354 s since 1904-01-01), timestamp(3699330034.2382703 s since 1904-01-01), timestamp(3699330035.2374697 s since 1904-01-01), timestamp(3699330036.2392607 s since 1904-01-01)], "Filtered X"=[135209.75320043054, 134926.99532732347, 134780.68456741524, 135167.01073154903, 135073.3060872024, 135183.4501426732, 134866.16950587436, 135137.4197911484, 135043.7151461262, 134885.8967985415, 135068.37426296223, 135086.4576165694, 134769.176979279, 134866.16950482436]}, {"TimeArray"=[timestamp(3699330022.9537086 s since 1904-01-01), timestamp(3699330023.955344 s since 1904-01-01), timestamp(3699330024.9525824 s since 1904-01-01), timestamp(3699330025.9546447 s since 1904-01-01), timestamp(3699330027.2328625 s since 1904-01-01), timestamp(3699330028.229321 s since 1904-01-01), timestamp(3699330029.2276254 s since 1904-01-01), timestamp(3699330030.2324934 s since 1904-01-01), timestamp(3699330031.232282 s since 1904-01-01), timestamp(3699330032.2356615 s since 1904-01-01), timestamp(3699330033.2346354 s since 1904-01-01), timestamp(3699330034.2382703 s since 1904-01-01), timestamp(3699330035.2374697 s since 1904-01-01), timestamp(3699330036.2392607 s since 1904-01-01)], "Filtered X"=[134731.7773170951, 134792.1921541982, 134855.89487302888, 135021.11095667956, 134986.99917837253, 135051.11288220997, 135072.48411682475, 135065.0863817246, 135057.68864645553, 134983.30031042264, 135033.8514996946, 135021.11095604982, 134952.47641433805, 134947.54459090874]}] caption="XY Graph"
  out "Last N M.A. Pressures":dbl[](array[numeric])=[134731.7773170951, 134792.1921541982, 134855.89487302888, 135021.11095667956, 134986.99917837253, 135051.11288220997, 135072.48411682475, 135065.0863817246, 135057.68864645553, 134983.30031042264, 135033.8514996946, 135021.11095604982, 134952.47641433805, 134947.54459090874] format="%_5e"
  out "Pav (Pa)":dbl=134969.47359128593 format="%0.4e"
  out "Pstd":dbl=105.89314471586617 format="%0.4e"
  out "File Refn DewarCTRL":refnum<file>
  out "Error Out (Dewar CTRL":errorcluster
  out "... more steps":u64
  in  "Current position":dbl format="%_4f"
  out "AZD-AZ status":string
  out "Opening rate (Closed:0, Full open:100)":dbl(knob)=8.822438978731505 scale=0.0..100.0
  in  "DOUT Raw state":bool[](array[boolean])=[FALSE, FALSE, FALSE, FALSE, FALSE, FALSE, FALSE, FALSE]
  out "DOUT Labels 2":string[](array[string])=["D_V1_NO", "D_V2_NC", "D_CV1", "D_H1", "D_HOME", "D_START", "D_M0", "D_M1"]
  in  "DOUT (PMC)":string="D_H1"
  in  "DOUT (PWR)":string="D_CV1"
  in  "lower limit (mA) \n(PMC)":dbl=4.0 format="%_3f"
  in  "upper limit (mA)\n (PMC)":dbl=40.0 format="%_3f"
  in  "OUTPUT\n(PMC)":bool
  in  "Set Current (mA)\n (PMC)":dbl=4.0 min=4.0 max=40.0 format="%_3g"
  in  "update values":bool
  out "USB 6218 AOUT":dbl[](array[numeric])=[0.004, 0.004, 0.06969546425555169, 0.06969546425555169]
  out "Graph 7":T10(graph) caption="XY Graph"
  in  "lower limit (mA)":dbl=4.0 format="%_3f"
  in  "SetCurrent 2 (mA)":dbl=4.0 min=4.0 max=500.0 format="%_3f"
  in  "upper limit (mA)":dbl=500.0 format="%_3f"
  out "error out (KIKUSI CTRL)":errorcluster
  out "ActualVoltage (V)":dbl[](array[numeric]) format="%_6g"
  out "ActualCurrent (A)":dbl[](array[numeric])=[0.004, 0.004] format="%_3e"
  in  "SetCurrent 1 (mA)":dbl=4.0 min=4.0 max=500.0 format="%_3g"
  in  "Output\n (ADCMT)":bool[](array[boolean])=[FALSE, FALSE]
  out "error out (ADCMT6420A)":errorcluster
  out "Monitor Current (mA)":dbl=11.069310829336025 min=0.0 max=1.9 format="%_4e"
  in  "update current":bool
  in  "lower limit (mA) \n(PWR)":dbl=4.0 format="%_3f"
  in  "upper limit (mA)\n (PWR)":dbl=20.0 format="%_3f"
  in  "CONTROL KIKUSUI?":bool=TRUE
  in  "OUTPUT\n(PWR)":bool
  in  "Set Current (mA)\n (PWR)":dbl=4.0 min=4.0 max=20.0 format="%_3g"
  in  "Voltage limits (V)":dbl[](array[numeric])=[12.0, 12.0] format="%_3f"
  in  "CtrlLabels":string[](array[string])=["CV2", "CV3"]
  in  "VISA":refnum<visa-resource-name>[](array[refnum])=["GPIB0::1::INSTR", "GPIB0::12::INSTR"]
  out "Initialized?":bool
  in  "InstName":string="ADCMT6240"
  out "Graph 6":T9(graph)=[{"TimeArray"=[timestamp(3695085214.3168983 s since 1904-01-01), timestamp(3695085244.964852 s since 1904-01-01), timestamp(3695085246.0168433 s since 1904-01-01), timestamp(3695085588.0010176 s since 1904-01-01)], "Filtered X"=[0.001, 0.005, 0.005, 0.01]}, {"TimeArray"=[timestamp(3695085214.3168983 s since 1904-01-01), timestamp(3695085244.964852 s since 1904-01-01), timestamp(3695085246.0168433 s since 1904-01-01), timestamp(3695085588.0010176 s since 1904-01-01)], "Filtered X"=[0.004, 0.004, 0.004, 0.004]}, {"TimeArray"=[timestamp(3695085214.3168983 s since 1904-01-01), timestamp(3695085244.964852 s since 1904-01-01), timestamp(3695085246.0168433 s since 1904-01-01), timestamp(3695085588.0010176 s since 1904-01-01)], "Filtered X"=[0.001, 0.005, 0.005, 0.01]}, {"TimeArray"=[timestamp(3695085214.3168983 s since 1904-01-01), timestamp(3695085244.964852 s since 1904-01-01), timestamp(3695085246.0168433 s since 1904-01-01), timestamp(3695085588.0010176 s since 1904-01-01)], "Filtered X"=[0.004, 0.004, 0.004, 0.004]}] caption="XY Graph"
  in  "Initialize":bool
  out "RUN Identifier 5":string="20210323_164300_RUNIV" caption="RUN Identifier"
  in  "Tab Control 3":enum32{"Basic control", "Advanced control"}(tab)=enum."Advanced control"
  in  "wait for home (s)":dbl=50.0
  in  "wait for open/close/stop (s)":dbl=2.0
  in  "AZD-AZ open":string="D_M0"
  in  "AZD-AZ close":string="D_M1"
  in  "AZD-AZ home":string="D_HOME"
  in  "AZD-AZ stop":string="D_STOP"
  in  "Motor stop":bool
  in  "Open 1/4":bool
  in  "Close 1/4":bool
  in  "Motor home":bool
  in  "N to close":u64=1
  in  "N to open":u64=1
  in  "Open N":bool
  in  "Close N":bool
  out "Close Command accepted":bool
  out "Open Command accepted":bool
  in  "DMMsConfig":T11(array[cluster])=[{"Label"="I_H1", "Active?"=TRUE, "VISA resource name"="USB0::0x1334::0x0204::262800066::INSTR", "Device"=enum."ADCMT7351", "Measurement"=enum."DC Currents", "FileFormat"="%.4e"}, {"Label"="V_H1", "Active?"=TRUE, "VISA resource name"="USB0::0x1334::0x0204::262800451::INSTR", "Device"=enum."ADCMT7351", "Measurement"=enum."DC Volts", "FileFormat"="%.4e"}, {"Label"="I_H2", "Active?"=TRUE, "VISA resource name"="GPIB0::23::INSTR", "Device"=enum."ADCMT7451", "Measurement"=enum."DC Currents", "FileFormat"="%.4e"}, {"Label"="V_H2", "Active?"=TRUE, "VISA resource name"="GPIB0::22::INSTR", "Device"=enum."Agilent34401A", "Measurement"=enum."DC Volts", "FileFormat"="%.4e"}, {"Label"="I_H4", "Active?"=TRUE, "VISA resource name"="GPIB0::21::INSTR", "Device"=enum."Agilent34401A", "Measurement"=enum."DC Currents", "FileFormat"="%.4e"}, {"Label"="V_H4", "Active?"=TRUE, "VISA resource name"="GPIB0::25::INSTR", "Device"=enum."Agilent34401A", "Measurement"=enum."DC Volts", "FileFormat"="%.4e"}]
  out "ƒ¢T=T_2 -T_1":dbl=-101388.71309149737
  out "Graph DMMs 3":T4(graph)=[{"TimeArray"=[timestamp(3695672642.6155486 s since 1904-01-01)], "DataArray"=[-2.68e-05]}, {"TimeArray"=[timestamp(3695672642.6155486 s since 1904-01-01)], "DataArray"=[-0.0014684]}, {"TimeArray"=[timestamp(3695672642.6155486 s since 1904-01-01)], "DataArray"=[-1.232e-05]}, {"TimeArray"=[timestamp(3695672642.6155486 s since 1904-01-01)], "DataArray"=[2.8262e-06]}, {"TimeArray"=[timestamp(3695672642.6155486 s since 1904-01-01)], "DataArray"=[3.71392e-06]}, {"TimeArray"=[timestamp(3695672642.6155486 s since 1904-01-01)], "DataArray"=[0.000182]}, {"TimeArray"=[timestamp(3695672642.6155486 s since 1904-01-01)], "DataArray"=[101407.09548804205]}, {"TimeArray"=[timestamp(3695672642.6155486 s since 1904-01-01)], "DataArray"=[-0.36185606613019977]}, {"TimeArray"=[timestamp(3695672642.6155486 s since 1904-01-01)], "DataArray"=[-3.0973798990583647]}, {"TimeArray"=[timestamp(3695672642.6155486 s since 1904-01-01)], "DataArray"=[18.382396544680894]}, {"TimeArray"=[timestamp(3695672642.6155486 s since 1904-01-01)], "DataArray"=[-48.20456535494683]}, {"TimeArray"=[timestamp(3695672642.6155486 s since 1904-01-01)], "DataArray"=[167.919]}, {"TimeArray"=[timestamp(3695672642.6155486 s since 1904-01-01)], "DataArray"=[163.1]}, {"TimeArray"=[timestamp(3695672642.6155486 s since 1904-01-01)], "DataArray"=[162.659]}, {"TimeArray"=[timestamp(3695672642.6155486 s since 1904-01-01)], "DataArray"=[160.848]}] caption="XY Graph"
  out "Q = I *V":dbl=3.935312e-08
  in  "index I":i64
  in  "index V":i64=1
  out "VariableSources":T12(array[ring])=[enum."USB6210", enum."USB6218AI", enum."USB6218AI", enum."USB6218AI", enum."USB6210", enum."LSI336", enum."LSI336", enum."LSI336", enum."LSI336"]
  in  "DMMsConfig (variables)":T13(array[cluster])=[{"Label"="P_3Hepot", "Active?"=TRUE, "Source"=enum."USB6210", "SourceLabel"="P_3Hepot", "FileFormat"="%6.4e"}, {"Label"="F_1", "Active?"=TRUE, "Source"=enum."USB6218AI", "SourceLabel"="F_1", "FileFormat"="%3.4f"}, {"Label"="F_4", "Active?"=TRUE, "Source"=enum."USB6218AI", "SourceLabel"="F_4", "FileFormat"="%3.4f"}, {"Label"="F_5", "Active?"=TRUE, "Source"=enum."USB6218AI", "SourceLabel"="F_5", "FileFormat"="%3.4f"}, {"Label"="DP_HEX4", "Active?"=TRUE, "Source"=enum."USB6210", "SourceLabel"="DP_HEX4", "FileFormat"="%4.3e"}, {"Label"="T3He6-1", "Active?"=TRUE, "Source"=enum."LSI336", "SourceLabel"="T3He6-1", "FileFormat"="%3.4f"}, {"Label"="T3He6-2", "Active?"=TRUE, "Source"=enum."LSI336", "SourceLabel"="T3He6-2", "FileFormat"="%3.4f"}, {"Label"="T3He7-1", "Active?"=TRUE, "Source"=enum."LSI336", "SourceLabel"="T3He7-1", "FileFormat"="%3.4f"}, {"Label"="T3He7-2", "Active?"=TRUE, "Source"=enum."LSI336", "SourceLabel"="T3He7-2", "FileFormat"="%3.4f"}]
  in  "Measure DMMs?":bool
  out "DMMsLabels":string[](array[string])=["I_H1", "V_H1", "I_H2", "V_H2", "I_H4", "V_H4", "P_3Hepot", "F_1", "F_4", "F_5", "DP_HEX4", "T3He6-1", "T3He6-2", "T3He7-1", "T3He7-2"]
  out "Active?":bool[](array[boolean])=[TRUE, TRUE, TRUE, TRUE, TRUE, TRUE, TRUE, TRUE, TRUE, TRUE, TRUE, TRUE, TRUE, TRUE, TRUE]
  out "DMM LastMeasurements":dbl[](array[numeric])=[-2.68e-05, -0.0014684, -1.232e-05, 2.8262e-06, 3.71392e-06, 0.000182, 101407.09548804205, -0.36185606613019977, -3.0973798990583647, 18.382396544680894, -48.20456535494683, 167.919, 163.1, 162.659, 160.848]
  out "Graph DMMs 2":T4(graph)=[{"TimeArray"=[timestamp(3695672642.6155486 s since 1904-01-01)], "DataArray"=[-2.68e-05]}, {"TimeArray"=[timestamp(3695672642.6155486 s since 1904-01-01)], "DataArray"=[-0.0014684]}, {"TimeArray"=[timestamp(3695672642.6155486 s since 1904-01-01)], "DataArray"=[-1.232e-05]}, {"TimeArray"=[timestamp(3695672642.6155486 s since 1904-01-01)], "DataArray"=[2.8262e-06]}, {"TimeArray"=[timestamp(3695672642.6155486 s since 1904-01-01)], "DataArray"=[3.71392e-06]}, {"TimeArray"=[timestamp(3695672642.6155486 s since 1904-01-01)], "DataArray"=[0.000182]}, {"TimeArray"=[timestamp(3695672642.6155486 s since 1904-01-01)], "DataArray"=[101407.09548804205]}, {"TimeArray"=[timestamp(3695672642.6155486 s since 1904-01-01)], "DataArray"=[-0.36185606613019977]}, {"TimeArray"=[timestamp(3695672642.6155486 s since 1904-01-01)], "DataArray"=[-3.0973798990583647]}, {"TimeArray"=[timestamp(3695672642.6155486 s since 1904-01-01)], "DataArray"=[18.382396544680894]}, {"TimeArray"=[timestamp(3695672642.6155486 s since 1904-01-01)], "DataArray"=[-48.20456535494683]}, {"TimeArray"=[timestamp(3695672642.6155486 s since 1904-01-01)], "DataArray"=[167.919]}, {"TimeArray"=[timestamp(3695672642.6155486 s since 1904-01-01)], "DataArray"=[163.1]}, {"TimeArray"=[timestamp(3695672642.6155486 s since 1904-01-01)], "DataArray"=[162.659]}, {"TimeArray"=[timestamp(3695672642.6155486 s since 1904-01-01)], "DataArray"=[160.848]}] caption="XY Graph"
  out "DMMFileName":string="20210209_084357_RUNIII_DMMs_20210209_084357.csv"
  out "error out (DMMs)":errorcluster
  out "cycle # (DMMs)":i32=7
  in  "Measurement Interval DMMs (ms)":i64=500
  in  "InstName DMMs":string="DMMs"
  in  "Initialize (DMMs)":bool
  out "Graph DMMs 1":T4(graph)=[{"TimeArray"=[timestamp(3695672642.6155486 s since 1904-01-01)], "DataArray"=[-2.68e-05]}, {"TimeArray"=[timestamp(3695672642.6155486 s since 1904-01-01)], "DataArray"=[-0.0014684]}, {"TimeArray"=[timestamp(3695672642.6155486 s since 1904-01-01)], "DataArray"=[-1.232e-05]}, {"TimeArray"=[timestamp(3695672642.6155486 s since 1904-01-01)], "DataArray"=[2.8262e-06]}, {"TimeArray"=[timestamp(3695672642.6155486 s since 1904-01-01)], "DataArray"=[3.71392e-06]}, {"TimeArray"=[timestamp(3695672642.6155486 s since 1904-01-01)], "DataArray"=[0.000182]}, {"TimeArray"=[timestamp(3695672642.6155486 s since 1904-01-01)], "DataArray"=[101407.09548804205]}, {"TimeArray"=[timestamp(3695672642.6155486 s since 1904-01-01)], "DataArray"=[-0.36185606613019977]}, {"TimeArray"=[timestamp(3695672642.6155486 s since 1904-01-01)], "DataArray"=[-3.0973798990583647]}, {"TimeArray"=[timestamp(3695672642.6155486 s since 1904-01-01)], "DataArray"=[18.382396544680894]}, {"TimeArray"=[timestamp(3695672642.6155486 s since 1904-01-01)], "DataArray"=[-48.20456535494683]}, {"TimeArray"=[timestamp(3695672642.6155486 s since 1904-01-01)], "DataArray"=[167.919]}, {"TimeArray"=[timestamp(3695672642.6155486 s since 1904-01-01)], "DataArray"=[163.1]}, {"TimeArray"=[timestamp(3695672642.6155486 s since 1904-01-01)], "DataArray"=[162.659]}, {"TimeArray"=[timestamp(3695672642.6155486 s since 1904-01-01)], "DataArray"=[160.848]}] caption="XY Graph"
  out "error out (DMM graphs)":errorcluster
  in  "Sample #":i32=5
  in  "index T_ 1":i64=6
  in  "index T_2":i64=9
  out "error out (DMMs) 2":errorcluster={"status"=TRUE, "code"=1, "source"="Close File in DMMsData.lvclass:DMMs_terminate.vi->CRYO_MASTER_FULL_RUN4.vi"}
  out "P_HEX7OUT":dbl=102831.98017524344 format="%_4e"
  out "P (HEX7 out)":dbl=102831.98017524344 format="%_4e"
  out "DP HEX5":dbl=5.509892853373055 format="%_4e"
  out "DP_HEX5":dbl=5.509892853373055 format="%_4e"
  in  "Diff pressure HEX5":string="DP_HEX5"
  out "3He pot level":dbl format="%_4f"
  in  "3He pot":string="L1"
  out "He level (3He)":dbl(slide) scale=0.0..100.0
  out "He level (1K) b":dbl(slide) scale=0.0..100.0
  out "He level (1K)":dbl(slide)=0.028411703634074498 scale=0.0..100.0
  out "He level (4K)":dbl(slide)=31.87854099600237 scale=0.0..100.0
  out "1K pot(b1)":dbl format="%_4f"
  in  "1K pot (b)":string="L2-2"
  in  "1K pot level":string="L2-1"
  out "L(1K) (a1)":dbl=0.028411703634074498 format="%_4f"
  in  "SensorLocation 2":T14(ring)=enum."T3He5"
  out "Temperature 2":dbl=13.2176
  out "DP HEX4":dbl=2.073087401132434 format="%_4e"
  in  "Diff pressure HEX4":string="DP_HEX4"
  out "V2":bool
  out "V1":bool
  out "F5 (1K pump ex.)":dbl=23.39313821847484 format="%_4f"
  out "F4 (3He in to HEX7)":dbl=-0.3684318274206404 format="%_3f"
  out "F3 (4He rtn flw via HEX7)":dbl=0.6141023076914145 format="%_4f"
  out "F1 (3He pump exhaust) flow":dbl=2.229000287561577 format="%_4f"
  out "P (Dewar)":dbl=133922.54729625225 format="%_4e"
  out "P (1K pot)":dbl=102778.35876990847 format="%_4e"
  out "P (3He pot)":dbl=102285.6157171335 format="%_4e"
  out "P (shield return)":dbl=102784.29179605731 format="%_4e"
  out "P (3He IN)":dbl=102917.4903816534 format="%_4e"
  out "P (4K reservoir)":dbl=103386.1520739023 format="%_4e"
  out "P (insulation)":dbl=0.0001467822274904493 format="%_4e"
  in  "1Kpot pump exhaust flow":string="F_5"
  out "F_5":dbl=23.39313821847484 format="%_4f"
  in  "3He incoming flow into HEX7":string="F_4"
  out "F_4":dbl=-0.3684318274206404 format="%_4f"
  out "F_3":dbl=0.6141023076914145 format="%_4f"
  in  "4He return flow from HEX7":string="F_3"
  out "F_2":dbl=6.5651805759101745 format="%_4f"
  in  "Shield flow":string="F_2"
  out "P_SldRTN":dbl=102784.29179605731 format="%_4e"
  in  "3He pot pressure":string="P_3Hepot"
  out "P_3Hepot":dbl=102285.6157171335 format="%_4e"
  in  "Shield return press.":string="P_SldRTN"
  out "F_1":dbl=2.229000287561577 format="%_4f"
  in  "3He pump exhaust flow":string="F_1"
  out "P_Dewar":dbl=133922.54729625225 format="%_4e"
  in  "Dewar pressure":string="P_Dewar"
  out "P_1Kpot":dbl=102778.35876990847 format="%_4e"
  in  "1Kpot pressure":string="P_1Kpot"
  out "P_3HeIN":dbl=102917.4903816534 format="%_4e"
  in  "3He inlet pressure":string="P_3HeIN"
  in  "4K reservoir pressure":string="P_4Kres"
  out "P_4Kres":dbl=103386.1520739023 format="%_4e"
  out "P_ins":dbl=0.0001467822274904493 format="%_4e"
  in  "Insulation vacuum":string="P_ins"
  out "T3He7-1/6-2 (3He pot) 2":dbl=16.396 format="%_4f"
  out "T3He7-1/7-2 (HEX1)":dbl=21.346 format="%_4f"
  out "T3He6-1/6-2 (3He pot) 2":dbl=19.8429 format="%_4f"
  out "T3He6-1/6-2 (HEX1)":dbl=19.0199 format="%_4f"
  out "T1K3-1/3-2 (1K pot) 2":dbl=12.0443 format="%_4f"
  out "T1K3-1/3-2 (1K pot)":dbl=12.015 format="%_4f"
  out "T4He1 (4K reservoir )":dbl=4.447 format="%_4f"
  out "Temperature 1":dbl=85.051
  in  "SensorLocation 1":T14(ring)=enum."TTH2"
  out "TIP7":dbl format="%_4g"
  out "T3He6-2":dbl=19.8429 format="%_4g"
  out "T3He7-2":dbl=16.396 format="%_4g"
  out "T3He6-1":dbl=19.0199 format="%_4g"
  out "T3He4":dbl=12.951 format="%_4g"
  out "T3He7-1":dbl=21.346 format="%_4g"
  out "T3He8":dbl=12.3577 format="%_4g"
  out "T3He5":dbl=13.2176 format="%_4g"
  out "T1K3-2":dbl=12.0443 format="%_4g"
  out "T1K3-1":dbl=12.015 format="%_4g"
  out "TIP6":dbl=110.79 format="%_4g"
  out "T3He9":dbl=10.898 format="%_4g"
  out "T1K5":dbl=10.992 format="%_4g"
  out "T1K4":dbl=11.658 format="%_4g"
  out "T1K2":dbl=330.07 format="%_4g"
  out "TIP5":dbl=114.8 format="%_4g"
  out "TIP4":dbl=70.626 format="%_4g"
  out "TIP3":dbl=83.788 format="%_4g"
  out "TIP2":dbl=130.11 format="%_4g"
  out "TIP1":dbl=252.77 format="%_4g"
  out "T1K6":dbl=243.0 format="%_4g"
  out "T4He10":dbl=221.22 format="%_4g"
  out "T4He8":dbl=161.53 format="%_4g"
  out "T4He7":dbl=143.04 format="%_4g"
  out "T3He1-3":dbl=272.06 format="%_4g"
  out "T3He1-2":dbl=276.82 format="%_4g"
  out "T4He9":dbl=171.21 format="%_4g"
  out "T4He6":dbl=62.642 format="%_4g"
  out "T4He5":dbl=55.799 format="%_4g"
  out "T4He4":dbl=28.983 format="%_4g"
  out "T4He2-2":dbl=36.266 format="%_4g"
  out "T4He2-1":dbl=34.464 format="%_4g"
  out "T4He3-4":dbl=279.75 format="%_4g"
  out "T4He3-3":dbl=279.78 format="%_4g"
  out "T4He3-2":dbl=282.4 format="%_4g"
  out "T4He3-1":dbl=282.27 format="%_4g"
  out "T3He1-4":dbl=271.93 format="%_4g"
  out "T3He3":dbl=5.052 format="%_4g"
  out "T3He2-2":dbl=53.128 format="%_4g"
  out "T3He2-1":dbl=56.993 format="%_4g"
  out "T1K1":dbl=4.668 format="%_4g"
  out "T4He1":dbl=4.447 format="%_4g"
  out "TTH1":dbl=54.48 format="%_4g"
  out "TTH2":dbl=85.051 format="%_4g"
  out "TTH4":dbl=218.62 format="%_4g"
  out "TTH3":dbl=145.0 format="%_4g"
  out "T3He1-1":dbl=276.68 format="%_4g"
  out "T3He10":dbl=238.58 format="%_4g"
  out "F2 (shield flow)":dbl=6.5651805759101745 format="%_4f"
  out "DP_HEX4":dbl=2.073087401132434 format="%_4e"
  in  "4K reservoir level":string="L3"
  out "L3":dbl=31.87854099600237 format="%_4f"
  out "RUN Identifier 6":string="20210323_164300_RUNIV" caption="RUN Identifier"
  in  "HEX7 out pressure":string="P_HEX7OUT"
  in  "CHF Graph Comment":string="CHF_TEST2"
  in  "REFRESH GRAPH":bool
  in  "RECORD GRAPH":bool
  out "Graph CHF log 2":T4(graph) caption="XY Graph"
  out "ƒ¢T_array":dbl[](array[numeric])=[52.7753, 52.7753, 52.7113, 52.7149, 52.7149, 52.4737, 52.4737, 52.4737, 52.3482, 52.3482, 52.178799999999995, 52.165000000000006, 52.165000000000006, 52.165000000000006, 52.0492, 52.0492, 51.9912, 51.9912, 51.9912, 51.7804, 51.7804, 51.7804, 51.6556, 51.6556, 51.6556, 51.5194, 51.5194, 51.447500000000005, 51.3779, 51.3779, 51.3779, 51.1899, 51.1899, 51.2118, 51.2118, 51.2118, 51.182199999999995, 51.1555, 51.1555, 51.0157, 51.0157, 51.0157, 50.9915, 50.9915, 50.8838, 50.926899999999996, 50.926899999999996, 50.861599999999996, 50.861599999999996, 50.861599999999996, 50.876400000000004, 50.876400000000004, 50.748400000000004, 50.7998, 50.7998, 50.7998, 50.7818, 50.7818, 50.8097, 50.8097, 50.8097, 50.7905, 50.7905, 50.7905, 50.8299, 50.8299, 50.8299, 50.8304, 50.8304, 50.8908, 50.884699999999995, 50.884699999999995, 51.0378, 51.0378, 51.0378, 51.019000000000005, 51.019000000000005, 51.120799999999996, 51.156600000000005, 51.156600000000005, 51.156600000000005, 51.2329, 51.2329, 51.369299999999996, 51.369299999999996, 51.369299999999996, 51.5356, 51.5356, 51.5356, 51.6671, 51.6671, 51.6671, 51.8208, 51.8208, 51.987899999999996, 52.0073, 52.0073, 52.2344, 52.2344, 52.2344, 52.459, 52.459, 52.672399999999996, 52.708999999999996, 52.708999999999996, 52.708999999999996, 52.9287, 52.9287, 53.1942, 53.1942, 53.1942, 53.5324, 53.5324, 53.5324, 53.849000000000004, 53.849000000000004, 53.849000000000004, 54.1092, 54.1092, 54.4229, 54.5156, 54.5156, 54.8154, 54.8154, 54.8154, 55.2085, 55.2085, 55.5868, 55.656800000000004, 55.656800000000004, 0.0, 0.0, 0.0, 0.0, 0.0, 0.0, 0.0, 0.0, 0.0, 0.0, 0.0, 0.0, 0.0, 0.0, 0.0, 0.0, 0.0, 0.0, 0.0, 0.0, 0.0, 0.0, 0.0, 0.0, 0.0, 0.0, 0.0, 0.0, 0.0, 0.0, 0.0, 0.0, 0.0, 0.0, 0.0, 0.0, 0.0, 0.0, 0.0, 0.0, 0.0, 0.0, 0.0, 0.0, 0.0, 0.0, 0.0, 0.0, 0.0, 0.0, 0.0, 0.0, 0.0, 0.0, 0.0, 0.0, 0.0, 0.0, 0.0, 0.0, 0.0, 0.0, 0.0, 0.0, 0.0, 0.0, 0.0, 0.0, 0.0, 0.0, 0.0, 0.0, 0.0, 0.0, 0.0, 0.0, 0.0, 0.0, 0.0, 0.0, 0.0, 0.0, 0.0, 0.0, 0.0, 0.0, 0.0, 0.0, 0.0, 0.0, 0.0, 0.0, 0.0, 0.0, 0.0, 0.0, 0.0, 0.0, 0.0, 0.0, 0.0, 0.0, 0.0, 0.0, 0.0, 0.0, 0.0, 0.0, 0.0, 0.0, 0.0, 0.0, 0.0, 0.0, 0.0, 0.0, 0.0, 0.0, 0.0, 0.0, 0.0, 0.0, 0.0, 0.0, 0.0, 0.0, 0.0, 0.0, 0.0, 0.0]
  out "Graph CHF":cluster{dbl[], dbl[]}(graph)={[52.7753, 52.7753, 52.7113, 52.7149, 52.7149, 52.4737, 52.4737, 52.4737, 52.3482, 52.3482, 52.178799999999995, 52.165000000000006, 52.165000000000006, 52.165000000000006, 52.0492, 52.0492, 51.9912, 51.9912, 51.9912, 51.7804, 51.7804, 51.7804, 51.6556, 51.6556, 51.6556, 51.5194, 51.5194, 51.447500000000005, 51.3779, 51.3779, 51.3779, 51.1899, 51.1899, 51.2118, 51.2118, 51.2118, 51.182199999999995, 51.1555, 51.1555, 51.0157, 51.0157, 51.0157, 50.9915, 50.9915, 50.8838, 50.926899999999996, 50.926899999999996, 50.861599999999996, 50.861599999999996, 50.861599999999996, 50.876400000000004, 50.876400000000004, 50.748400000000004, 50.7998, 50.7998, 50.7998, 50.7818, 50.7818, 50.8097, 50.8097, 50.8097, 50.7905, 50.7905, 50.7905, 50.8299, 50.8299, 50.8299, 50.8304, 50.8304, 50.8908, 50.884699999999995, 50.884699999999995, 51.0378, 51.0378, 51.0378, 51.019000000000005, 51.019000000000005, 51.120799999999996, 51.156600000000005, 51.156600000000005, 51.156600000000005, 51.2329, 51.2329, 51.369299999999996, 51.369299999999996, 51.369299999999996, 51.5356, 51.5356, 51.5356, 51.6671, 51.6671, 51.6671, 51.8208, 51.8208, 51.987899999999996, 52.0073, 52.0073, 52.2344, 52.2344, 52.2344, 52.459, 52.459, 52.672399999999996, 52.708999999999996, 52.708999999999996, 52.708999999999996, 52.9287, 52.9287, 53.1942, 53.1942, 53.1942, 53.5324, 53.5324, 53.5324, 53.849000000000004, 53.849000000000004, 53.849000000000004, 54.1092, 54.1092, 54.4229, 54.5156, 54.5156, 54.8154, 54.8154, 54.8154, 55.2085, 55.2085, 55.5868, 55.656800000000004, 55.656800000000004, 0.0, 0.0, 0.0, 0.0, 0.0, 0.0, 0.0, 0.0, 0.0, 0.0, 0.0, 0.0, 0.0, 0.0, 0.0, 0.0, 0.0, 0.0, 0.0, 0.0, 0.0, 0.0, 0.0, 0.0, 0.0, 0.0, 0.0, 0.0, 0.0, 0.0, 0.0, 0.0, 0.0, 0.0, 0.0, 0.0, 0.0, 0.0, 0.0, 0.0, 0.0, 0.0, 0.0, 0.0, 0.0, 0.0, 0.0, 0.0, 0.0, 0.0, 0.0, 0.0, 0.0, 0.0, 0.0, 0.0, 0.0, 0.0, 0.0, 0.0, 0.0, 0.0, 0.0, 0.0, 0.0, 0.0, 0.0, 0.0, 0.0, 0.0, 0.0, 0.0, 0.0, 0.0, 0.0, 0.0, 0.0, 0.0, 0.0, 0.0, 0.0, 0.0, 0.0, 0.0, 0.0, 0.0, 0.0, 0.0, 0.0, 0.0, 0.0, 0.0, 0.0, 0.0, 0.0, 0.0, 0.0, 0.0, 0.0, 0.0, 0.0, 0.0, 0.0, 0.0, 0.0, 0.0, 0.0, 0.0, 0.0, 0.0, 0.0, 0.0, 0.0, 0.0, 0.0, 0.0, 0.0, 0.0, 0.0, 0.0, 0.0, 0.0, 0.0, 0.0, 0.0, 0.0, 0.0, 0.0, 0.0, 0.0], [64.988847618, 0.0008371808639999999, 0.0008371808639999999, 0.0008371808639999999, 0.0008371808639999999, 0.0008371808639999999, 0.0008371808639999999, 0.0008371808639999999, 0.0008371808639999999, 0.0008371808639999999, 0.027133083646800005, 0.027133083646800005, 0.027133083646800005, 0.027133083646800005, 0.027133083646800005, 0.027133083646800005, 0.027133083646800005, 0.027133083646800005, 0.497141592024, 0.497141592024, 0.497141592024, 0.497141592024, 0.497141592024, 0.497141592024, 0.497141592024, 0.497141592024, 1.476215545728, 1.476215545728, 1.476215545728, 1.476215545728, 1.476215545728, 1.476215545728, 1.476215545728, 1.476215545728, 1.476215545728, 3.02773055424, 3.02773055424, 3.02773055424, 3.02773055424, 3.02773055424, 3.02773055424, 3.02773055424, 3.02773055424, 4.86484683444, 4.86484683444, 4.86484683444, 4.86484683444, 4.86484683444, 4.86484683444, 4.86484683444, 4.86484683444, 4.86484683444, 7.4475440352, 7.4475440352, 7.4475440352, 7.4475440352, 7.4475440352, 7.4475440352, 7.4475440352, 7.4475440352, 10.986195312400001, 10.986195312400001, 10.986195312400001, 10.986195312400001, 10.986195312400001, 10.986195312400001, 10.986195312400001, 10.986195312400001, 14.5582761144, 14.5582761144, 14.5582761144, 14.5582761144, 14.5582761144, 14.5582761144, 14.5582761144, 14.5582761144, 14.5582761144, 16.831454674799996, 16.831454674799996, 16.831454674799996, 16.831454674799996, 16.831454674799996, 16.831454674799996, 16.831454674799996, 16.831454674799996, 23.431170976799997, 23.431170976799997, 23.431170976799997, 23.431170976799997, 23.431170976799997, 23.431170976799997, 23.431170976799997, 23.431170976799997, 28.729140804, 28.729140804, 28.729140804, 28.729140804, 28.729140804, 28.729140804, 28.729140804, 28.729140804, 28.729140804, 31.9837009252, 31.9837009252, 31.9837009252, 31.9837009252, 31.9837009252, 31.9837009252, 31.9837009252, 31.9837009252, 40.691919848000005, 40.691919848000005, 40.691919848000005, 40.691919848000005, 40.691919848000005, 40.691919848000005, 40.691919848000005, 40.691919848000005, 47.4670420756, 47.4670420756, 47.4670420756, 47.4670420756, 47.4670420756, 47.4670420756, 47.4670420756, 47.4670420756, 47.4670420756, 50.1891742, 50.1891742, 50.1891742, 3.935312e-08, 3.935312e-08, 3.935312e-08, 3.935312e-08, 3.935312e-08, 3.935312e-08, 3.935312e-08, 3.935312e-08, 3.935312e-08, 3.935312e-08, 3.935312e-08, 3.935312e-08, 3.935312e-08, 3.935312e-08, 3.935312e-08, 3.935312e-08, 3.935312e-08, 3.935312e-08, 3.935312e-08, 3.935312e-08, 3.935312e-08, 3.935312e-08, 3.935312e-08, 3.935312e-08, 3.935312e-08, 3.935312e-08, 3.935312e-08, 3.935312e-08, 3.935312e-08, 3.935312e-08, 3.935312e-08, 3.935312e-08, 3.935312e-08, 3.935312e-08, 3.935312e-08, 3.935312e-08, 3.935312e-08, 3.935312e-08, 3.935312e-08, 3.935312e-08, 3.935312e-08, 3.935312e-08, 3.935312e-08, 3.935312e-08, 3.935312e-08, 3.935312e-08, 3.935312e-08, 3.935312e-08, 3.935312e-08, 3.935312e-08, 3.935312e-08, 3.935312e-08, 3.935312e-08, 3.935312e-08, 3.935312e-08, 3.935312e-08, 3.935312e-08, 3.935312e-08, 3.935312e-08, 3.935312e-08, 3.935312e-08, 3.935312e-08, 3.935312e-08, 3.935312e-08, 3.935312e-08, 3.935312e-08, 3.935312e-08, 3.935312e-08, 3.935312e-08, 3.935312e-08, 3.935312e-08, 3.935312e-08, 3.935312e-08, 3.935312e-08, 3.935312e-08, 3.935312e-08, 3.935312e-08, 3.935312e-08, 3.935312e-08, 3.935312e-08, 3.935312e-08, 3.935312e-08, 3.935312e-08, 3.935312e-08, 3.935312e-08, 3.935312e-08, 3.935312e-08, 3.935312e-08, 3.935312e-08, 3.935312e-08, 3.935312e-08, 3.935312e-08, 3.935312e-08, 3.935312e-08, 3.935312e-08, 3.935312e-08, 3.935312e-08, 3.935312e-08, 3.935312e-08, 3.935312e-08, 3.935312e-08, 3.935312e-08, 3.935312e-08, 3.935312e-08, 3.935312e-08, 3.935312e-08, 3.935312e-08, 3.935312e-08, 3.935312e-08, 3.935312e-08, 3.935312e-08, 3.935312e-08, 3.935312e-08, 3.935312e-08, 3.935312e-08, 3.935312e-08, 3.935312e-08, 3.935312e-08, 3.935312e-08, 3.935312e-08, 3.935312e-08, 3.935312e-08, 3.935312e-08, 3.935312e-08, 3.935312e-08, 3.935312e-08, 3.935312e-08, 3.935312e-08, 3.935312e-08, 3.935312e-08]}
  in  "V_lim_low (V)":dbl format="%_5f"
  in  "V_lim_up (V)":dbl=120.0 format="%_5f"
  out "V":dbl=-0.0014684
  out "I":dbl=-2.68e-05
  out "Q":dbl=3.935312e-08
  out "T_low":dbl
  out "error out (Agilent)":errorcluster
  in  "VISA (Agilent 34402)":refnum<visa-resource-name>="USB0::0x0957::0x0407::MY44010230::INSTR"
  out "Agilent\nIntialized?":bool
  in  "Initialize (Agilent)":bool=TRUE
  in  "OUTPUT \nKenwood":bool
  in  "Kenwood set V (V)":dbl min=0.0 max=120.0 format="%_5f"
  out "Graph CHF log 1":T4(graph) caption="XY Graph"
  out "CHF Data Labels":string[](array[string])=["I_H1", "V_H1", "P_3Hepot", "F_1", "F_4", "F_5", "DP_HEX4", "T3He6-1", "T3He6-2", "T3He7-1", "T3He7-2", "T1K3-1", "T1K3-2"]
  out "CHF last data":dbl[](array[numeric])=[-2.68e-05, -0.0014684, -820.4557600165222, -4.458565576380751, 0.2595549305851412, 0.3318884836547996, -250.30990640814414, 0.0, 0.0, 0.0, 0.0, 0.0, 0.0]
  out "Error out (CHF rec)":errorcluster
  out "CHF measurement counter":i32
  out "T_high":dbl
  out "ƒ¢T":dbl
  out "Q_array":dbl[](array[numeric])=[64.988847618, 0.0008371808639999999, 0.0008371808639999999, 0.0008371808639999999, 0.0008371808639999999, 0.0008371808639999999, 0.0008371808639999999, 0.0008371808639999999, 0.0008371808639999999, 0.0008371808639999999, 0.027133083646800005, 0.027133083646800005, 0.027133083646800005, 0.027133083646800005, 0.027133083646800005, 0.027133083646800005, 0.027133083646800005, 0.027133083646800005, 0.497141592024, 0.497141592024, 0.497141592024, 0.497141592024, 0.497141592024, 0.497141592024, 0.497141592024, 0.497141592024, 1.476215545728, 1.476215545728, 1.476215545728, 1.476215545728, 1.476215545728, 1.476215545728, 1.476215545728, 1.476215545728, 1.476215545728, 3.02773055424, 3.02773055424, 3.02773055424, 3.02773055424, 3.02773055424, 3.02773055424, 3.02773055424, 3.02773055424, 4.86484683444, 4.86484683444, 4.86484683444, 4.86484683444, 4.86484683444, 4.86484683444, 4.86484683444, 4.86484683444, 4.86484683444, 7.4475440352, 7.4475440352, 7.4475440352, 7.4475440352, 7.4475440352, 7.4475440352, 7.4475440352, 7.4475440352, 10.986195312400001, 10.986195312400001, 10.986195312400001, 10.986195312400001, 10.986195312400001, 10.986195312400001, 10.986195312400001, 10.986195312400001, 14.5582761144, 14.5582761144, 14.5582761144, 14.5582761144, 14.5582761144, 14.5582761144, 14.5582761144, 14.5582761144, 14.5582761144, 16.831454674799996, 16.831454674799996, 16.831454674799996, 16.831454674799996, 16.831454674799996, 16.831454674799996, 16.831454674799996, 16.831454674799996, 23.431170976799997, 23.431170976799997, 23.431170976799997, 23.431170976799997, 23.431170976799997, 23.431170976799997, 23.431170976799997, 23.431170976799997, 28.729140804, 28.729140804, 28.729140804, 28.729140804, 28.729140804, 28.729140804, 28.729140804, 28.729140804, 28.729140804, 31.9837009252, 31.9837009252, 31.9837009252, 31.9837009252, 31.9837009252, 31.9837009252, 31.9837009252, 31.9837009252, 40.691919848000005, 40.691919848000005, 40.691919848000005, 40.691919848000005, 40.691919848000005, 40.691919848000005, 40.691919848000005, 40.691919848000005, 47.4670420756, 47.4670420756, 47.4670420756, 47.4670420756, 47.4670420756, 47.4670420756, 47.4670420756, 47.4670420756, 47.4670420756, 50.1891742, 50.1891742, 50.1891742, 3.935312e-08, 3.935312e-08, 3.935312e-08, 3.935312e-08, 3.935312e-08, 3.935312e-08, 3.935312e-08, 3.935312e-08, 3.935312e-08, 3.935312e-08, 3.935312e-08, 3.935312e-08, 3.935312e-08, 3.935312e-08, 3.935312e-08, 3.935312e-08, 3.935312e-08, 3.935312e-08, 3.935312e-08, 3.935312e-08, 3.935312e-08, 3.935312e-08, 3.935312e-08, 3.935312e-08, 3.935312e-08, 3.935312e-08, 3.935312e-08, 3.935312e-08, 3.935312e-08, 3.935312e-08, 3.935312e-08, 3.935312e-08, 3.935312e-08, 3.935312e-08, 3.935312e-08, 3.935312e-08, 3.935312e-08, 3.935312e-08, 3.935312e-08, 3.935312e-08, 3.935312e-08, 3.935312e-08, 3.935312e-08, 3.935312e-08, 3.935312e-08, 3.935312e-08, 3.935312e-08, 3.935312e-08, 3.935312e-08, 3.935312e-08, 3.935312e-08, 3.935312e-08, 3.935312e-08, 3.935312e-08, 3.935312e-08, 3.935312e-08, 3.935312e-08, 3.935312e-08, 3.935312e-08, 3.935312e-08, 3.935312e-08, 3.935312e-08, 3.935312e-08, 3.935312e-08, 3.935312e-08, 3.935312e-08, 3.935312e-08, 3.935312e-08, 3.935312e-08, 3.935312e-08, 3.935312e-08, 3.935312e-08, 3.935312e-08, 3.935312e-08, 3.935312e-08, 3.935312e-08, 3.935312e-08, 3.935312e-08, 3.935312e-08, 3.935312e-08, 3.935312e-08, 3.935312e-08, 3.935312e-08, 3.935312e-08, 3.935312e-08, 3.935312e-08, 3.935312e-08, 3.935312e-08, 3.935312e-08, 3.935312e-08, 3.935312e-08, 3.935312e-08, 3.935312e-08, 3.935312e-08, 3.935312e-08, 3.935312e-08, 3.935312e-08, 3.935312e-08, 3.935312e-08, 3.935312e-08, 3.935312e-08, 3.935312e-08, 3.935312e-08, 3.935312e-08, 3.935312e-08, 3.935312e-08, 3.935312e-08, 3.935312e-08, 3.935312e-08, 3.935312e-08, 3.935312e-08, 3.935312e-08, 3.935312e-08, 3.935312e-08, 3.935312e-08, 3.935312e-08, 3.935312e-08, 3.935312e-08, 3.935312e-08, 3.935312e-08, 3.935312e-08, 3.935312e-08, 3.935312e-08, 3.935312e-08, 3.935312e-08, 3.935312e-08, 3.935312e-08, 3.935312e-08, 3.935312e-08, 3.935312e-08]
  out "CHF file name":string="20210205_150936_RUNIII_CHF20210205_154539_CHF_TEST1.csv"
  out "Graph CHF log 3":T4(graph) caption="XY Graph"
  out "File Refnum (CHF)":refnum<file>
  in  "Tab Control":T15(tab)=enum."Beam heat emulation"
  in  "ƒ¢V / cycle (V)":dbl=0.5 format="%_4f"
  in  "V start (V)":dbl format="%_4f"
  in  "V_end (V)":dbl=65.0 format="%_4f"
  in  "CHF cycle interval (s) (>1s)":dbl=1.0 format="%_3f"
  in  "Data I":T16={"Source"=enum."DMMs", "SourceLabel"="I_H1"}
  in  "Data V":T16={"Source"=enum."DMMs", "SourceLabel"="V_H1"}
  in  "RecordSettings":T17(array[cluster])=[{"Source"=enum."DMMs", "SourceLabel"="I_H1", "FileFormat"="%4.4e"}, {"Source"=enum."DMMs", "SourceLabel"="V_H1", "FileFormat"="%4.4f"}, {"Source"=enum."USB6210", "SourceLabel"="P_3Hepot", "FileFormat"="%4.4e"}, {"Source"=enum."USB6218AI", "SourceLabel"="F_1", "FileFormat"="%4.4f"}, {"Source"=enum."USB6218AI", "SourceLabel"="F_4", "FileFormat"="%4.4f"}, {"Source"=enum."USB6218AI", "SourceLabel"="F_5", "FileFormat"="%4.4f"}, {"Source"=enum."USB6210", "SourceLabel"="DP_HEX4", "FileFormat"="%4.4e"}, {"Source"=enum."LSI336", "SourceLabel"="T3He6-1", "FileFormat"="%4.4f"}, {"Source"=enum."LSI336", "SourceLabel"="T3He6-2", "FileFormat"="%4.4f"}, {"Source"=enum."LSI336", "SourceLabel"="T3He7-1", "FileFormat"="%4.4f"}, {"Source"=enum."LSI336", "SourceLabel"="T3He7-2", "FileFormat"="%4.4f"}, {"Source"=enum."LSI336", "SourceLabel"="T1K3-1", "FileFormat"="%4.4f"}, {"Source"=enum."LSI336", "SourceLabel"="T1K3-2", "FileFormat"="%4.4f"}]
  in  "Data T_high":T16={"Source"=enum."LSI336", "SourceLabel"="T3He7-2"}
  in  "Data T_low":T16={"Source"=enum."LSI336", "SourceLabel"="T3He6-1"}
  out "CHF log file name":string="20210318_151011_RUNIV_20210318_151011_CHFlog.csv"
  in  "STOP CHF":bool
  in  "START CHF":bool
  in  "V_peak":dbl=65.0 format="%_4f"
  out "Heat Cycle counter":i32=3
  in  "t_off":dbl=5.0 format="%_4f"
  in  "t_on":dbl=10.0 format="%_4f"
  in  "Q_input":dbl=65.0 format="%_4f"
  out "V_input":dbl=1.0 format="%_4f"
  out "R_sample":dbl=65.0 format="%_4f"
  in  "V_sample":dbl=65.0 format="%_4f"
  out "Q_sample":dbl=65.0 format="%_4f"
  in  "I_sample":dbl=1.0 format="%_4f"
  in  "START heater cycle":bool
  in  "STOP heater cycle":bool
  out "Series 1":string[](array[string])=["P_ins", "P_4Kres", "P_3HeIN", "P_SldRTN", "P_3Hepot", "P_1Kpot", "P_Dewar(old)", "P_HEX7OUT", "P_IP", "P_Dewar"]
  out "Series 2":string[](array[string])=["L1(old)", "L2-1", "L1", "L3", "L_Dewar", "R_L2-2", "L2-2"]
  out "Series 3":string[](array[string])=["F_1", "F_2", "F_3", "F_4", "F_5", "I_CV"]
  out "Series 4":string[](array[string])=["T3He10", "T3He1-1", "TTH3", "TTH4", "TTH1", "TTH2", "T4He1", "T1K1", "T3He2-1", "T3He2-2", "T3He3", "T3He1-4", "T4He3-1", "T4He3-2", "T4He3-3", "T4He3-4", "T4He2-1", "T4He2-2", "T4He4", "T4He5", "T4He6", "T4He9", "T1K2", "T1K4", "T1K5", "T3He4", "T3He9", "T1K3-1", "T1K3-2", "T3He5", "T3He8", "T3He6-1", "T3He6-2", "T3He7-1", "T3He7-2"]
  out "Plot errors":errorcluster={"status"=TRUE, "code"=1077, "source"="Property Node (arg 1) in CRYO_MASTER_FULL_RUN4.vi\n<APPEND>\nProperty Name: <b>Active Plot</b>"}
  out "LastMeasurementConfig (218)":T18(array[cluster])=[{"LSIName"="LSI218A", "Active?"=TRUE, "LastData"=[238.58, 276.68, 145.02, 218.62, 54.478, 85.05, 4.442, 4.661], "Labels"=["T3He10", "T3He1-1", "TTH3", "TTH4", "TTH1", "TTH2", "T4He1", "T1K1"]}, {"LSIName"="LSI218B", "Active?"=TRUE, "LastData"=[30.0, 0.0, 0.0, 0.0, 56.991, 53.134, 5.055, 271.93], "Labels"=["N.C.", "N.C.", "N.C.", "N.C.", "T3He2-1", "T3He2-2", "T3He3", "T3He1-4"]}, {"LSIName"="LSI218C", "Active?"=TRUE, "LastData"=[282.27, 282.4, 279.79, 279.75, 34.466, 36.266, 28.98, 55.8], "Labels"=["T4He3-1", "T4He3-2", "T4He3-3", "T4He3-4", "T4He2-1", "T4He2-2", "T4He4", "T4He5"]}, {"LSIName"="LSI218D", "Active?"=TRUE, "LastData"=[62.643, 171.21, 276.82, 272.08, 143.05, 161.51, 221.22, 243.0], "Labels"=["T4He6", "T4He9", "T3He1-2", "T3He1-3", "T4He7", "T4He8", "T4He10", "T1K6"]}, {"LSIName"="LSI218E", "Active?"=TRUE, "LastData"=[252.76, 0.0, 130.11, 688.49, 83.786, 70.623, 114.8, 688.58], "Labels"=["TIP1", "N.C.", "TIP2", "N.C.", "TIP3", "TIP4", "TIP5", "N.C."]}, {"LSIName"="LSI218F", "Active?"=TRUE, "LastData"=[14.054, 11.753, 10.988, 12.938, 10.918, 110.83, 0.433, 0.0], "Labels"=["T1K2", "T1K4", "T1K5", "T3He4", "T3He9", "TIP6", "N.C.", "N.C."]}]
  out "DataArrayConv (USB6210)":dbl[][](array[numeric])=[[0.0001467822274904493, 103386.1520739023, 102917.4903816534, 102784.29179605731, 102285.6157171335, 102778.35876990847, 0.0, 2.073087401132434, 5.509892853373055, 10.022340765034453, 0.028411703634074498, 0.17703499366301226, 31.87854099600237, 102831.98017524344, 6.658695577811817e-05, 5.600304013757209], [0.00014331210383532943, 103419.04061540413, 102917.49038025808, 102876.37970352173, 102299.64398756107, 102783.61937258235, 0.0, 0.009359860621893645, 6.307429085038785, 9.980910378649359, 0.03893370650245273, 0.17703499365619763, 31.866703704233657, 102960.24547937719, 6.903046749339257e-05, 5.354612085872782]]
  out "LastMeasurementConfig (336)":T18(array[cluster])=[{"LSIName"="LSi336X", "Active?"=TRUE, "LastData"=[12.0158, 12.046, 13.2196, 12.3577], "Labels"=["T1K3-1", "T1K3-2", "T3He5", "T3He8"]}, {"LSIName"="LSi336Y", "Active?"=TRUE, "LastData"=[19.0262, 19.857, 21.3351, 16.3982], "Labels"=["T3He6-1", "T3He6-2", "T3He7-1", "T3He7-2"]}]
  out "DataArrayConv (USB6218)":dbl[][](array[numeric])=[[2.229000287561577, 6.5651805759101745, 0.6141023076914145, -0.3684318274206404, 23.39313821847484, -0.0038120682713622734, -24.983607626866934, 133922.54729625225, 14.198759390010572], [1.8476051977193715, 6.559919954343005, 0.5720173311260397, -0.35856816207260195, 23.485199087329573, -0.00019463958134809388, -24.924425628844947, 134754.38150670484, 14.212571383113936]]
  out "TimeArray (USB6218)":timestamp[](array[timestamp])=[timestamp(3699330182.9543066 s since 1904-01-01), timestamp(3699330183.99275 s since 1904-01-01)]
  out "Data Array sizes (6210)":i32[](array[numeric])=[2, 16]
  out "DataArraySize (6218)":i32[](array[numeric])=[2, 9]
  out "TimeArray size (6218)":i32=2
  out "TimeArray (LSI336)":timestamp[](array[timestamp])=[timestamp(3699330182.9493194 s since 1904-01-01), timestamp(3699330183.988761 s since 1904-01-01)]
  out "TimeArray Size (336)":i32=2
  out "DataArray (336)":dbl[][](array[numeric])=[[12.015, 12.0443, 13.2176, 12.3577, 19.0199, 19.8429, 21.346, 16.396], [12.0158, 12.046, 13.2196, 12.3577, 19.0262, 19.857, 21.3351, 16.3982]]
  out "DataArray size (336)":i32[](array[numeric])=[2, 8]
  out "LastData (LSI218)":dbl[](array[numeric])=[238.58, 276.68, 145.02, 218.62, 54.478, 85.05, 4.442, 4.661, 30.0, 0.0, 0.0, 0.0, 56.991, 53.134, 5.055, 271.93, 282.27, 282.4, 279.79, 279.75, 34.466, 36.266, 28.98, 55.8, 62.643, 171.21, 276.82, 272.08, 143.05, 161.51, 221.22, 243.0, 252.76, 0.0, 130.11, 688.49, 83.786, 70.623, 114.8, 688.58, 14.054, 11.753, 10.988, 12.938, 10.918, 110.83, 0.433, 0.0]
  out "TempSensorsLocations":T19(array[ring])=[enum."T3He10", enum."T3He1-1", enum."TTH3", enum."TTH4", enum."TTH1", enum."TTH2", enum."T4He1", enum."T1K1", enum."N.C.", enum."N.C.", enum."N.C.", enum."N.C.", enum."T3He2-1", enum."T3He2-2", enum."T3He3", enum."T3He1-4", enum."T4He3-1", enum."T4He3-2", enum."T4He3-3", enum."T4He3-4", enum."T4He2-1", enum."T4He2-2", enum."T4He4", enum."T4He5", enum."T4He6", enum."T4He9", enum."T3He1-2", enum."T3He1-3", enum."T4He7", enum."T4He8", enum."T4He10", enum."T1K6", enum."TIP1", enum."N.C.", enum."TIP2", enum."N.C.", enum."TIP3", enum."TIP4", enum."TIP5", enum."N.C.", enum."T1K2", enum."T1K4", enum."T1K5", enum."T3He4", enum."T3He9", enum."TIP6", enum."N.C.", enum."N.C.", enum."T1K3-1", enum."T1K3-2", enum."T3He5", enum."T3He8", enum."T3He6-1", enum."T3He6-2", enum."T3He7-1", enum."T3He7-2"]
  out "AllTemperatures":dbl[](array[numeric])=[238.58, 276.68, 145.0, 218.62, 54.48, 85.051, 4.447, 4.668, 30.0, 0.0, 0.0, 0.0, 56.993, 53.128, 5.052, 271.93, 282.27, 282.4, 279.78, 279.75, 34.464, 36.266, 28.983, 55.799, 62.642, 171.21, 276.82, 272.06, 143.04, 161.53, 221.22, 243.0, 252.77, 0.0, 130.11, 688.49, 83.788, 70.626, 114.8, 688.58, 330.07, 11.658, 10.992, 12.951, 10.898, 110.79, 0.433, 0.0, 12.015, 12.0443, 13.2176, 12.3577, 19.0199, 19.8429, 21.346, 16.396]
  out "error out (frontpanel screenshots)":errorcluster
  out "error out (graph operations)":errorcluster
  out "error out (monthly folder creation)":errorcluster={"status"=TRUE, "code"=10, "source"="Create Folder in CRYO_MASTER_FULL_RUN4.vi<APPEND>\nC:\\LabVIEW\\DATA\\Google\\TUCAN Experiments\\KEK_cryotests_2019-2020\\data\\screenshots\\202103"}
  out "RUN Identifier 7":string="20210323_164300_RUNIV" caption="RUN Identifier"
  out "error out (notifier)":errorcluster
  # "GLOBAL STATUS/CONTROL"
  # "Global Settings"
  # "USB6210 Analog inputs Settings"
  # "USB6218 Analog inputs Settings"
  # "USB6218/6210 Digital Outputs"
  # "USB6218 Analog Output Settings"
  # "LSI218 Settings"
  # "LSI336 Settings"
  # "HP 34401A (He level meter)"
  # "Graph screenshots"
  # "Configuration"
  # "Activated only when *FIll state* = TRUE"
  # "Activated only when *FIll state* = TRUE"
  # "Vavle Status"
  # "OPEN"
  # "CLOSED"
  # "ADCMT6240A Control/Status"
  # "ADCMT6240A Initialization"
  # "Set Currents (mA)"
  # "PWR400H CTRL via USB6218"
  # "PMC18-3A CTRL via USB6218"
  # "USB6218 low-level control"
  # "Stepping motor AZD-AX"
  # "DMM configurations"
  # "DMM measurements"
  # "CAUTION: ADCMT 7351 does not have 4-wire resistance measurement function. \n 4-Wire Resistance --> 2-Wire Resistance wih Low Power for this device"
  # "Representative temperatures"
  # "Pressures / Flows"
  # "Labels"
  # "Values"
  # "Helium Levels"
  # "Manual Control of Kenwood"
  # "Automatic Boiling Cruve Measurement"
  # "Before the measurement\n - Intialize Agilent 34402 (FG)\n - Refresh the CHF graph if necessary\n - Go to DMMs tab and check that DMM measurement is running \n - Fill in the CHF measurement parameters below \nThen press START CHF!"
  # "Measurement Configurations"
  # "Channel selection"
  # "Q = I x V"
  # "ƒ¢T = T_high - T_low"
  # "Record Configurations"
  # "Heat emulation"
  # "Before starting, \n - turn off the boiling curve measuremnt on the other tab\n - make sure that the DMMs are running"
  # "Calculator"
  # "Previous measurement:"
  # "Caclulate V which corresponds to derired Q:"
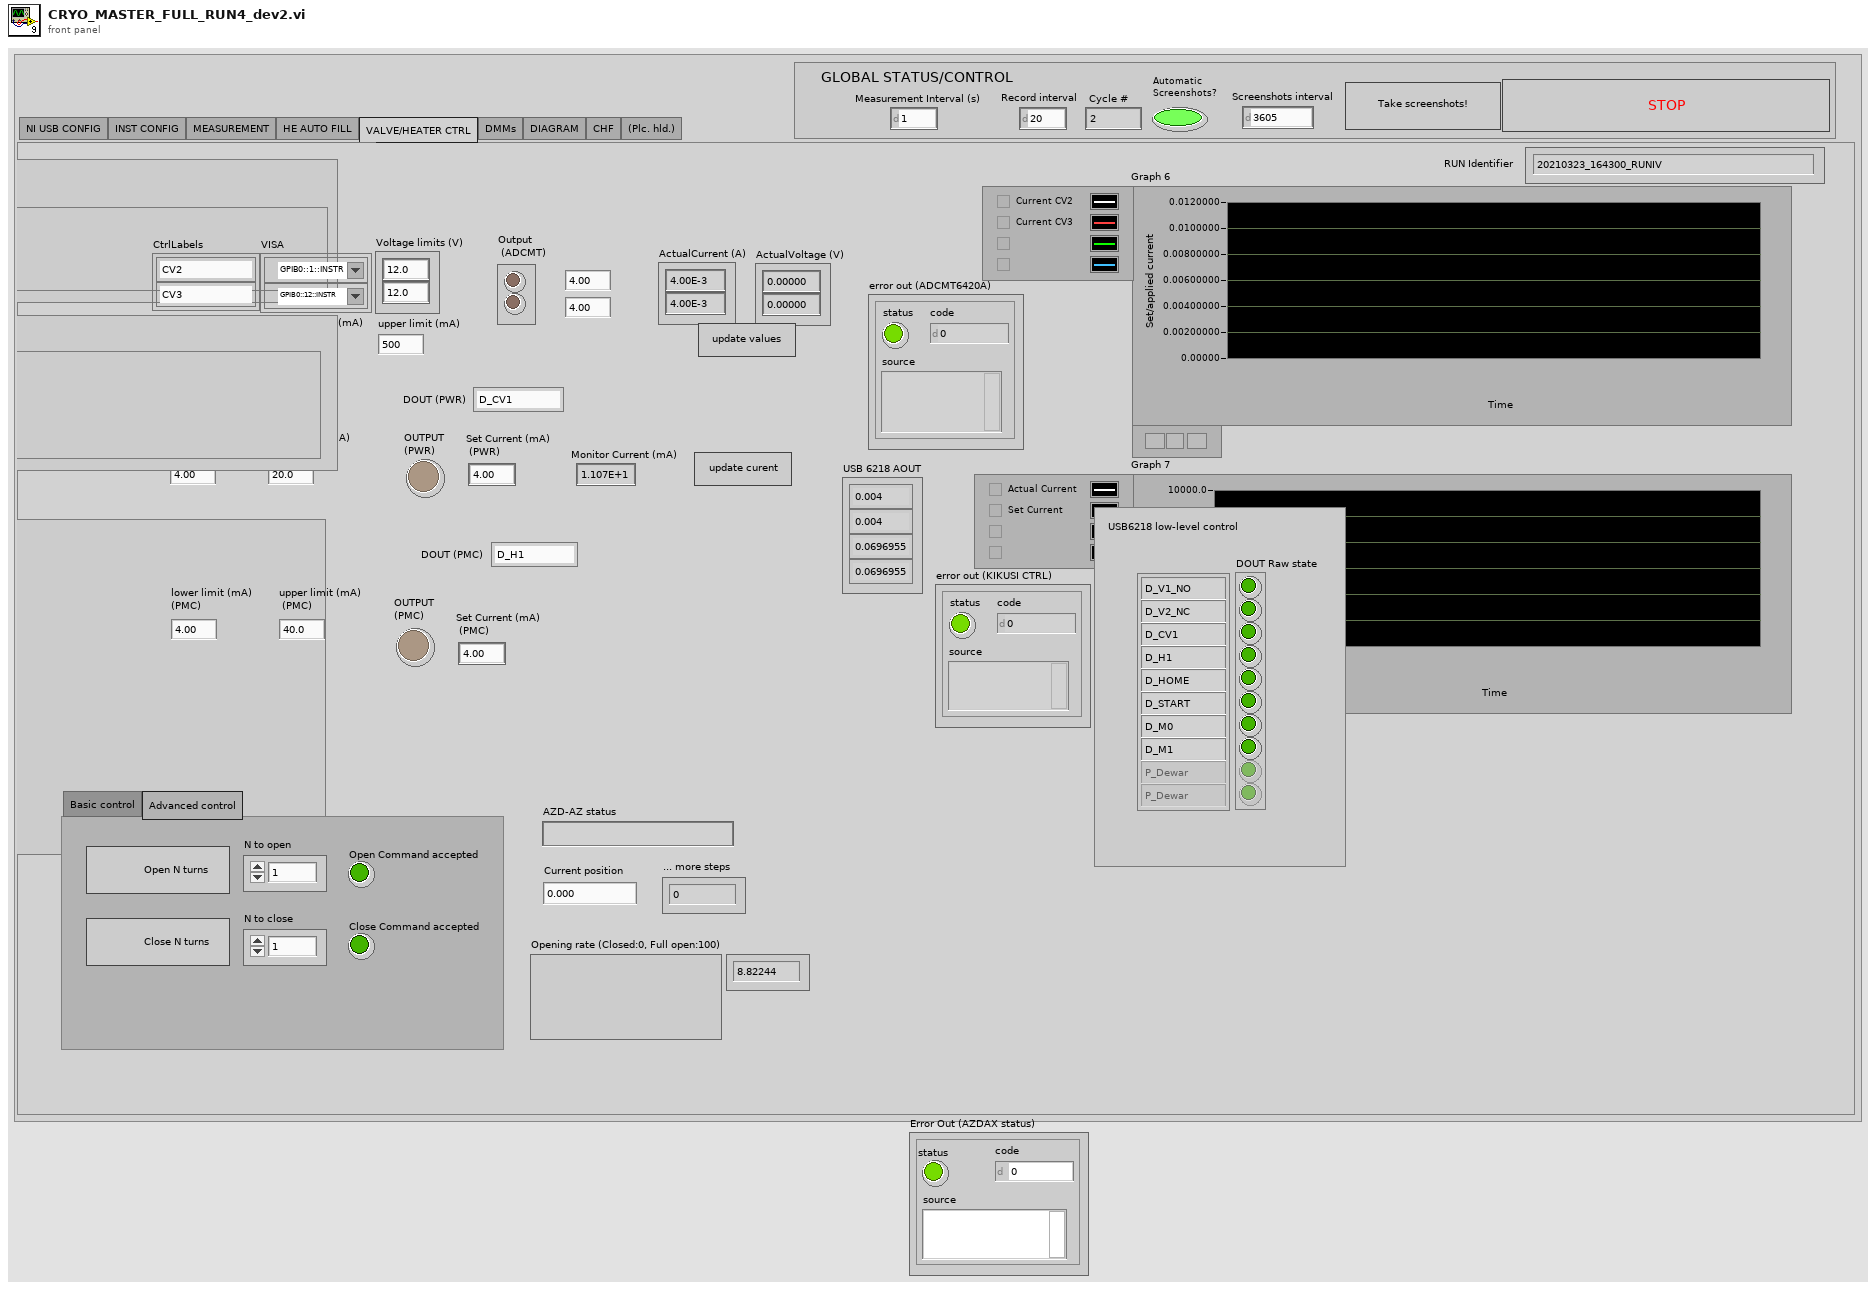
[diagram p1: front panel]
types:
  T1 = enum32{"NI USB CONFIG", "INST CONFIG", "MEASUREMENT", "HE AUTO FILL", "VALVE/HEATER CTRL", "DMMs", "DIAGRAM", "CHF", "(Plc. hld.)"}
  T2 = cluster{"Label":string, "FileFormat":string, "Active?":bool, "Physical CH":tag, " terminal\n type":i32, "ConversionType":cluster{"Type":enum16{"Raw", "SimpleProp", "CC-10_COMBINED", "CC-10_LOG", "LeakDet_EXP", "LeakDet_Mantissa", "Baratron"}, "ConversionParameters":dbl[]}, "VoltageLimits":dbl[]}[]
  T3 = cluster{"LSIName":string, "Labels":string[], "SensorLocations":enum16{"N.C.", "T3He1-1", "T3He1-2", "T3He1-3", "T3He1-4", "T3He2-1", "T3He2-2", "T3He3", "T3He4", "T3He5", "T3He6-1", "T3He6-2", "T3He7-1", "T3He7-2", "T3He8", "T3He9", "T3He10", "T4He1", "T4He2-1", "T4He2-2", "T4He3-1", "T4He3-2", "T4He3-3", "T4He3-4", "T4He4", "T4He5", "T4He6", "T4He7", "T4He8", "T4He9", "T4He10", "T1K1", "T1K2", "T1K3-1", "T1K3-2", "T1K4", "T1K5", "T1K6", "TIP1", "TIP2", "TIP3", "TIP4", "TIP5", "TIP6", "TIP7", "TTH1", "TTH2", "TTH3", "TTH4"}[], "Active?":bool, "VISA res. name":refnum<visa-resource-name>}[]
  T4 = cluster{"TimeArray":timestamp[], "DataArray":dbl[]}[]
  T5 = enum32{"USB6210", "USB6218", "Temeprature (1)", "Temperature (2)", "Temperature (3)"}
  T6 = enum16{"Intialized", "Ready", "Measuring", "Terminated"}
  T7 = enum16{"Initialized", "Ready", "Measuring", "Terminated"}
  T8 = enum16{"USB6210", "USB6218AI", "USB6218AO", "LSI218", "LSI336"}
  T9 = cluster{"TimeArray":timestamp[], "Filtered X":dbl[]}[]
  T10 = cluster{"TimeArray (USB6218)":timestamp[], "DataArrayConv (USB6218)":dbl[]}[]
  T11 = cluster{"Label":string, "Active?":bool, "VISA resource name":refnum<visa-resource-name>, "Device":enum16{"Agilent34401A", "ADCMT7351", "HP3478A", "ADCMT7451"}, "Measurement":enum16{"DC Volts", "DC Currents", "2-Wire Resistance", "4-Wire Resistance"}, "FileFormat":string}[]
  T12 = enum16{"USB6210", "USB6218AI", "USB6218AO", "LSI218", "LSI336"}[]
  T13 = cluster{"Label":string, "Active?":bool, "Source":enum16{"USB6210", "USB6218AI", "USB6218AO", "LSI218", "LSI336"}, "SourceLabel":string, "FileFormat":string}[]
  T14 = enum16{"N.C.", "T3He1-1", "T3He1-2", "T3He1-3", "T3He1-4", "T3He2-1", "T3He2-2", "T3He3", "T3He4", "T3He5", "T3He6-1", "T3He6-2", "T3He7-1", "T3He7-2", "T3He8", "T3He9", "T3He10", "T4He1", "T4He2-1", "T4He2-2", "T4He3-1", "T4He3-2", "T4He3-3", "T4He3-4", "T4He4", "T4He5", "T4He6", "T4He7", "T4He8", "T4He9", "T4He10", "T1K1", "T1K2", "T1K3-1", "T1K3-2", "T1K4", "T1K5", "T1K6", "TIP1", "TIP2", "TIP3", "TIP4", "TIP5", "TIP6", "TIP7", "TTH1", "TTH2", "TTH3", "TTH4"}
  T15 = enum32{"Boiling curve measurement", "Beam heat emulation"}
  T16 = cluster{"Source":enum16{"USB6210", "USB6218AI", "USB6218AO", "LSI218", "LSI336", "DMMs"}, "SourceLabel":string}
  T17 = cluster{"Source":enum16{"USB6210", "USB6218AI", "USB6218AO", "LSI218", "LSI336", "DMMs"}, "SourceLabel":string, "FileFormat":string}[]
  T18 = cluster{"LSIName":string, "Active?":bool, "LastData":dbl[], "Labels":string[]}[]
  T19 = enum16{"N.C.", "T3He1-1", "T3He1-2", "T3He1-3", "T3He1-4", "T3He2-1", "T3He2-2", "T3He3", "T3He4", "T3He5", "T3He6-1", "T3He6-2", "T3He7-1", "T3He7-2", "T3He8", "T3He9", "T3He10", "T4He1", "T4He2-1", "T4He2-2", "T4He3-1", "T4He3-2", "T4He3-3", "T4He3-4", "T4He4", "T4He5", "T4He6", "T4He7", "T4He8", "T4He9", "T4He10", "T1K1", "T1K2", "T1K3-1", "T1K3-2", "T1K4", "T1K5", "T1K6", "TIP1", "TIP2", "TIP3", "TIP4", "TIP5", "TIP6", "TIP7", "TTH1", "TTH2", "TTH3", "TTH4"}[]
  T20 = cluster{"TimeArray (USB6218)":timestamp[], "DataArrayConv (USB6218)":dbl[]}
  T21 = cluster{"appended array":timestamp[], "ActualCurrentArray":dbl[]}
  T22 = cluster{"appended array":timestamp[], "SetCurrentArray":dbl[]}
  T23 = cluster{"appended array":timestamp[], "SetCurrentArray":dbl[]}[]
  T24 = typedef "imagedata.ctl" = cluster{"image type":i32, "image depth":i32, "image":u8[], "mask":u8[], "colors":u32[], "Rectangle":cluster{"left":i16, "top":i16, "right":i16, "bottom":i16}}
  T25 = enum16{"open", "replace", "create", "open or create", "replace or create", "replace or create with confirmation"}
  T26 = cluster{"TimeArray":timestamp[], "DataArrayConv":dbl[]}[]
  T27 = cluster{"IndexArray":i64[], "TimeArray":timestamp[], "DataArrayRaw":dbl[][], "DataArrayConv":dbl[][], "LDArray":dbl[]}
  T28 = cluster{"InstName":string, "Active?":bool, "Status":enum16{"Intialized", "Ready", "Measuring", "Terminated"}, "Labels":string[], "LabelLD":string, "FileFormat":string[], "FileFormatLD":string, "ReadLeakDet?":bool}
  T29 = cluster{"AOUT Labels[0]":string, "AOUT Labels[1]":string, "AOUT Labels[2]":string, "AOUT Labels[3]":string, "AOUT Labels[4]":string, "AOUT Labels[5]":string, "AOUT Labels[6]":string, "AOUT Labels[7]":string, "AOUT Labels[8]":string}
  T30 = cluster{"LastTimeArray":timestamp[], "LastDataArray":dbl[]}
  T31 = cluster{"LastTimeArray":timestamp[], "LastDataArray":dbl[]}[]
  T32 = cluster{"TimeArray":timestamp[], "DataArrayConv":dbl[]}
  T33 = cluster{"TimeArray":timestamp[], "DataArrayConv (USB6218)":dbl[]}
  T34 = cluster{"TimeArray":timestamp[], "M.A. Array":dbl[]}
  T35 = cluster{"TimeArray":timestamp[], "M.A. Array":dbl[]}[]
  T36 = cluster{"TimeArray":timestamp[], "DataArray":dbl[]}
  T37 = enum16{"USB6210", "USB6218AI", "USB6218AO", "LSI218", "LSI336", "DMMs"}
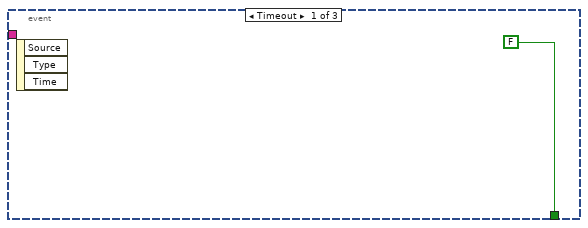
[diagram p3: hidden frame]
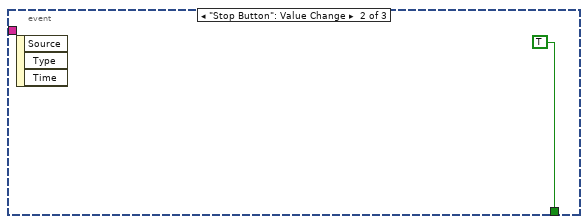
[diagram p4: hidden frame]
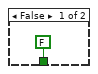
[diagram p5: hidden frame]
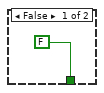
[diagram p7: hidden frame]
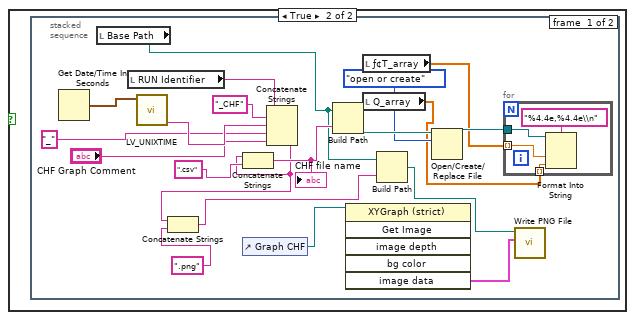
[diagram p8: hidden frame]
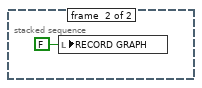
[diagram p9: hidden frame]
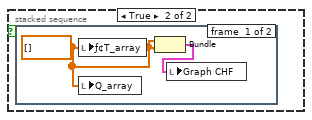
[diagram p10: hidden frame]
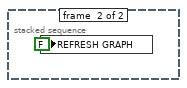
[diagram p11: hidden frame]
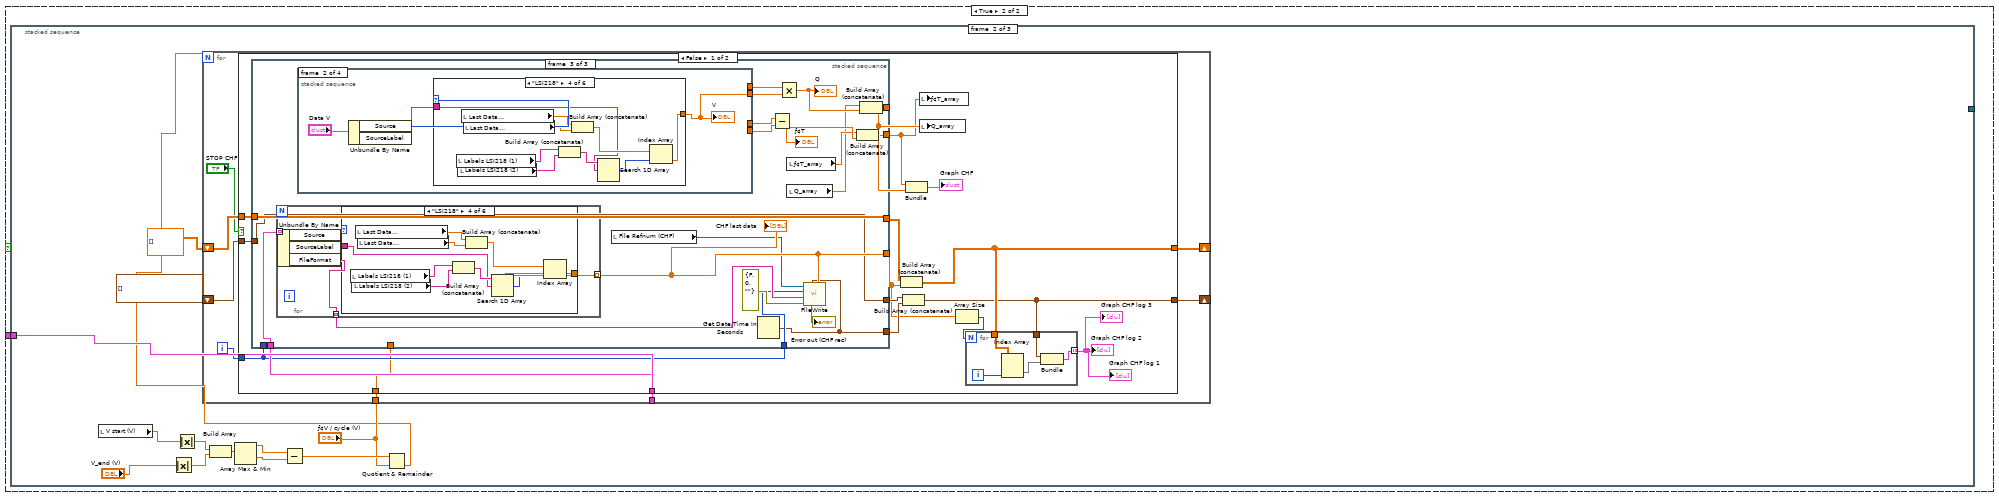
[diagram p12: hidden frame]
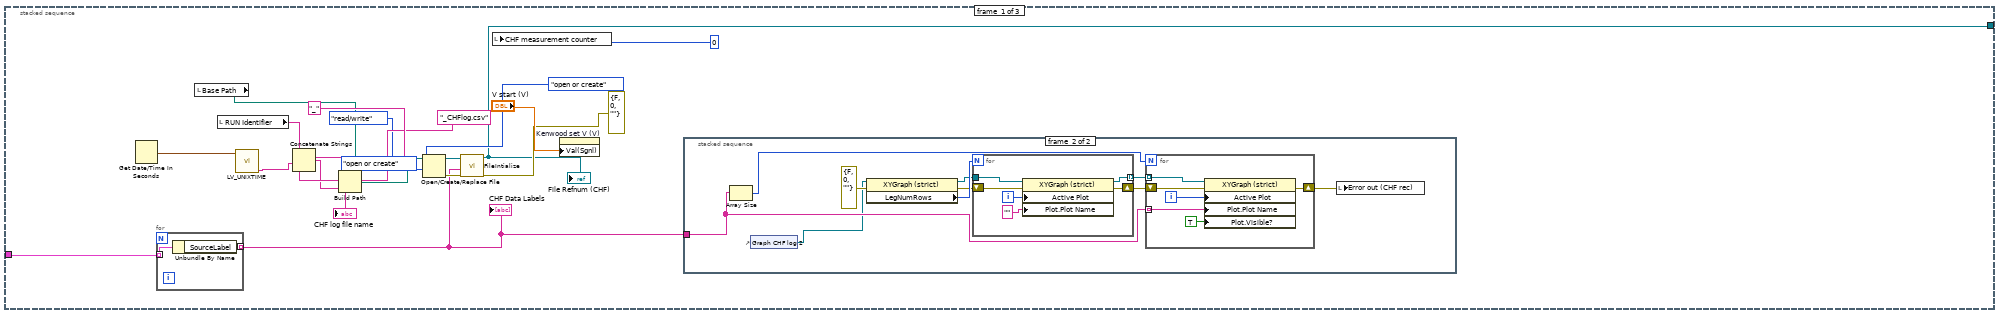
[diagram p13: hidden frame]
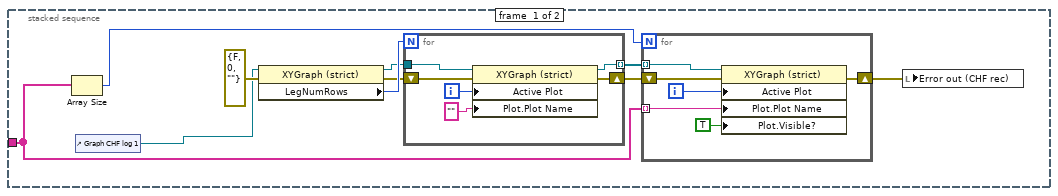
[diagram p14: hidden frame]
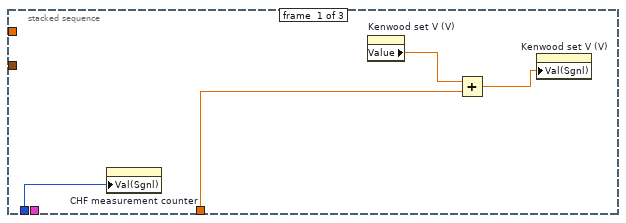
[diagram p15: hidden frame]
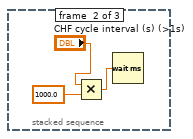
[diagram p16: hidden frame]
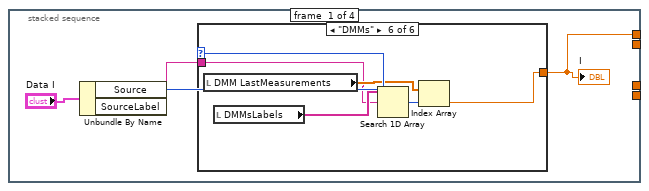
[diagram p17: hidden frame]
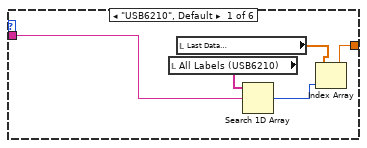
[diagram p18: hidden frame]
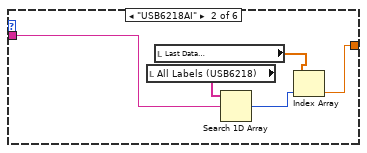
[diagram p19: hidden frame]
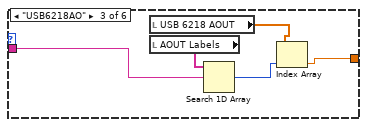
[diagram p20: hidden frame]
diagram:
  w17 = TRUE ("create if not found? (T)")
  w21 = errorcluster {"status"=FALSE, "code"=0, "source"=""} ("error in (no error)")
  w6 = errorcluster {"status"=FALSE, "code"=0, "source"=""} ("error in (no error)")
  n1 = while {
    shift-right: [w45] -> _
    shift-left: dbl[] [] -> [w51]
    shift-right: [w48] -> _
    shift-left: timestamp[] [] -> [w50]
    i -> [w49]
    stop <- w52 stop-if-true
    n2 = Wait (ms)(milliseconds to wait=u32 131) -> ()  [unwired: 1 out]
    n3 = event shown="[7] \"Open N\", \"Close N\": Value Change" {
      selector: _ -> [_ _ _ _ _ _ _ _]
      dyn-events: _ -> [_ _ _ _ _ _ _ _]
      timeout: _ -> [_ _ _ _ _ _ _ _]
      tunnel: [_ TRUE _ _ _ _ _ _] -> w52
      tunnel: w49 -> [_ _ _ w100 _ _ _ _]
      tunnel: [_ _ _ w99 w183 _ _ _] -> w45
      tunnel: w51 -> [_ _ _ w96 w183 _ _ _]
      tunnel: [w53 w63 _ w98 w182 w186 _ _] -> w48
      tunnel: w50 -> [w53 w63 _ w97 w182 w186 _ _]
      tunnel: [_ _ _ w87 _ _ _ _] -> w44
      event Timeout {
        n4 = event-data() -> ()  [unwired: 1 in, 3 out]
      }
      event "Stop Button": Value Change {
        w54 = FALSE
        n5 = event-data() -> ()  [unwired: 1 in, 3 out]
        n6 = local read "error out (USB6210/6218 DOUT)"() -> (w62:errorcluster)
        n7 = local read "error out (USB6210/6218 AOUT)"() -> (w59:errorcluster)
        n8 = local read "DOUT task out"() -> (w58:refnum<k21>)
        n9 = local read "AO task out"() -> (w65:refnum<k21>)
        n10 = property on="OUTPUT\n(PWR)" class="Bool (strict)"("Value"=w54) -> ()  [unwired: 2 in, 2 out]
        n11 = property on="V2 (N.C.)" class="Bool (strict)"("Val(Sgnl)"=w54) -> ()  [unwired: 2 in, 2 out]
        n12 = property on="OUTPUT\n(PMC)" class="Bool (strict)"("Value"=w54) -> ()  [unwired: 2 in, 2 out]
        n13 = Build Array(w54, w54, w54, w54) -> (w61:bool[])
        n14 = Not(x=w54) -> (.not. x?=w55:bool)
        n15 = call <vilib>:"DAQmx Clear Task.vi"("task in"=w65, "error in"=w59) -> ("error out"=w64:errorcluster)  [unwired: 13 in]
        n16 = property on="V1 (N.O.)" class="Bool (strict)"("Val(Sgnl)"=w55) -> ()  [unwired: 2 in, 2 out]
        n17 = call <vilib>:"DAQmx Write (Digital 1D Bool NChan 1Samp 1Line).vi"("task/channels in"=w58, "data"=w61, "timeout"=10.0, "error in"=w62) -> ("task out"=w57:refnum<k21>, "error out"=w56:errorcluster)  [unwired: 9 in, 1 out]
        n18 = call <vilib>:"DAQmx Clear Task.vi"("task in"=w57, "error in"=w56) -> ("error out"=w66:errorcluster)  [unwired: 13 in]
        n19 = local write "error out (USB6210/6218 AOUT)"(w64) -> ()
        n20 = local write "error out (USB6210/6218 DOUT)"(w66) -> ()
      }
      event "V1 (N.O.)", "V2 (N.C.)": Value Change {
        n21 = event-data() -> ()  [unwired: 1 in, 3 out]
        n22 = local read "Cycle #"() -> (w72:u32)
        n23 = Greater?(x=w72, y=u32 0) -> (0:w70:bool)
        n24 = case shown="False" w70 {
          tunnel: "V1 (N.O.)" -> [_ w83]
          tunnel: "V2 (N.C.)" -> [_ w73]
          frame False {
          }
          frame True {
            n25 = local read "DOUT6218 Labels"() -> (w74:string[])
            n26 = property on="DOUT Raw state" class="Arr (strict)"() -> ("Value"=w82:bool[])  [unwired: 2 in, 2 out]
            n27 = Search 1D Array(1D array=w74, element="D_V1_NO") -> (index of element=w81:i32)  [unwired: 1 in]
            n28 = Search 1D Array(1D array=w74, element="D_V2_NC") -> (index of element=w80:i32)  [unwired: 1 in]
            n29 = Not(x=w83) -> (.not. x?=w76:bool)
            n30 = Replace Array Subset(array=w82, new element=w76, index=w81) -> (w79:bool[])
            n31 = Replace Array Subset(array=w79, new element=w73, index=w80) -> (w78:bool[])
            n32 = property on="DOUT Raw state" class="Arr (strict)"("Val(Sgnl)"=w78) -> ()  [unwired: 2 in, 2 out]
          }
        }
        "V1" <- "V1 (N.O.)"
        "V2" <- "V2 (N.C.)"
      }
      event "Set Current (mA)\n (PMC)", "Set Current (mA)\n (PWR)", "update current": Value Change {
        n33 = event-data() -> ()  [unwired: 1 in, 3 out]
        n34 = case shown="True" "CONTROL KIKUSUI?" {
          tunnel: w100 -> [_ w151]
          tunnel: [w110 w144] -> w99
          tunnel: [w113 w143] -> w98
          tunnel: w97 -> [w115 w146]
          tunnel: w96 -> [w111 w145]
          tunnel: "Set Current (mA)\n (PWR)" -> [_ w123]
          tunnel: "Set Current (mA)\n (PMC)" -> [_ w127]
          frame False {
            w112 = 0.0 ("element")
            n35 = Get Date/Time In Seconds() -> (seconds since 1Jan1904=w114:timestamp)
            n36 = local read "AO task out"() -> (w120:refnum<k21>)
            n37 = Build Array (concatenate)(w115, w114) -> (w113:timestamp[])
            n38 = Build Array (concatenate)(w111, w112) -> (w110:dbl[])
            n39 = Build Array(w112, w112) -> (w118:dbl[])
            n40 = call <vilib>:"DAQmx Write (Analog 1D DBL NChan 1Samp).vi"("task/channels in"=w120, "data"=w118, "timeout"=100.0, "error in"=errorcluster {"status"=FALSE, "code"=0, "source"=""}) -> ("task out"=w121:refnum<k21>, "error out"=w116:errorcluster)  [unwired: 9 in, 1 out]
            n41 = local write "AO task out"(w121) -> ()
            n42 = local write "error out (KIKUSI CTRL)"(w116) -> ()
          }
          frame True {
            w138 = 2 ("index")
            n43 = xnode "Formula"("X1"=w123) -> ("Result"=w140:dbl)  [unwired: 1 in, 1 out]
            n44 = xnode "Formula"("X1"=w127) -> ("Result"=w134:dbl)  [unwired: 1 in, 1 out]
            n45 = Build Array (concatenate)(w145, w123) -> (w144:dbl[])
            n46 = In Range and Coerce(upper limit=10.0, x=w140, lower limit=0.0 ("y")) -> (coerced(x)=w132:dbl, In Range?=w133:bool)
            n47 = In Range and Coerce(upper limit=10.0, x=w134, lower limit=0.0 ("y")) -> (coerced(x)=w129:dbl, In Range?=w130:bool)
            n48 = case shown="False" w133 {
              tunnel: w132 -> [_ w163]
              tunnel: [0.0 ("upper limit") w163] -> w131
              frame False {
              }
              frame True {
              }
            }
            n49 = case shown="True" w130 {
              tunnel: w129 -> [_ w161]
              tunnel: [0.0 ("upper limit") w161] -> w128
              frame False {
              }
              frame True {
              }
            }
            n50 = Multiply(x=w123, y=0.001) -> (x*y=w122:dbl)
            n51 = Multiply(x=w127, y=0.001) -> (x*y=w126:dbl)
            n52 = local read "File Refn USB AO"() -> (w152:refnum<file>)
            n53 = Build Array(w122, w126, w131, w128) -> (w139:dbl[])
            "USB 6218 AOUT" <- w139
            n54 = Initialize Array("%.3f", 4 ("dimension size")) -> (w153:string[])
            n55 = Get Date/Time In Seconds() -> (seconds since 1Jan1904=w147:timestamp)
            n56 = local read "AO task out"() -> (w157:refnum<k21>)
            n57 = call "FileWrite.vi"("DataArray"=w139, "Time Stamp"=w147, "Error In"=errorcluster {"status"=FALSE, "code"=0, "source"=""} ("error in"), "FileFormat"=w153, "Index"=w151, "refnum in"=w152) -> ("Error Out"=w149:errorcluster, "Byte Stream File Refnum"=w148:refnum<file>)  [unwired: 4 in]
            n58 = Build Array (concatenate)(w146, w147) -> (w143:timestamp[])
            n59 = Array Subset(array=w139, index=w138, length=w138) -> (w137:dbl[])
            n60 = local write "File Refn USB AO"(w148) -> ()
            n61 = call <vilib>:"DAQmx Write (Analog 1D DBL NChan 1Samp).vi"("task/channels in"=w157, "data"=w137, "timeout"=100.0, "error in"=w149) -> ("task out"=w158:refnum<k21>, "error out"=→"error out (KIKUSI CTRL)":errorcluster)  [unwired: 9 in, 1 out]
            n62 = local write "AO task out"(w158) -> ()
          }
        }
        n63 = local read "All Labels (USB6218)"() -> (w93:string[])
        n64 = local read "DataArrayConv (USB6218)"() -> (w92:dbl[][])
        n65 = local read "Last Data \n(USB6218)"() -> (w89:dbl[])
        n66 = local read "TimeArray (USB6218)"() -> (w90:timestamp[])
        n67 = Search 1D Array(1D array=w93, element="I_CV") -> (index of element=w94:i32)  [unwired: 1 in]
        n68 = Index Array(array=w92, index (row)=w94) -> (element=w91:dbl[])  [unwired: 1 in]
        n69 = Index Array(array=w89, index=w94) -> (element=w86:dbl)
        n70 = Bundle("TimeArray (USB6218)"=w90, "DataArrayConv (USB6218)"=w91) -> (w87:T20)  [unwired: 1 in]
        n71 = xnode "Formula"("X1"=w86) -> ("Result"=→"Monitor Current (mA)":dbl)  [unwired: 1 in, 1 out]
      }
      event "upper limit (mA)\n (PWR)", "lower limit (mA) \n(PWR)": Value Change {
        n72 = event-data() -> ()  [unwired: 1 in, 6 out]
        n73 = property on="Set Current (mA)\n (PWR)" class="DigNum (strict)"("Maximum"="upper limit (mA)\n (PWR)", "Minimum"="lower limit (mA) \n(PWR)") -> ()  [unwired: 2 in, 2 out]
        n74 = property on="Set Current (mA)\n (PMC)" class="DigNum (strict)"("Maximum"="upper limit (mA)\n (PMC)", "Minimum"="lower limit (mA) \n(PMC)") -> ()  [unwired: 2 in, 2 out]
      }
      event "OUTPUT\n(PWR)", "OUTPUT\n(PMC)": Value Change {
        n75 = event-data() -> ()  [unwired: 1 in, 6 out]
        n76 = local read "Cycle #"() -> (w189:u32)
        n77 = Greater?(x=w189, y=u32 0) -> (0:w187:bool)
        n78 = case shown="False" w187 {
          frame False {
          }
          frame True {
            (unwired) FALSE
            n79 = local read "DOUT6218 Labels"() -> (w195:string[])
            n80 = local read "DOUT Raw state"() -> (w190:bool[])
            n81 = Search 1D Array(1D array=w195, element="DOUT (PWR)") -> (index of element=w198:i32)  [unwired: 1 in]
            n82 = Search 1D Array(1D array=w195, element="DOUT (PMC)") -> (index of element=w193:i32)  [unwired: 1 in]
            n83 = Replace Array Subset(array=w190, new element="OUTPUT\n(PWR)", index=w198) -> (w192:bool[])
            n84 = Replace Array Subset(array=w192, new element="OUTPUT\n(PMC)", index=w193) -> (w191:bool[])
            n85 = property on="DOUT Raw state" class="Arr (strict)"("Val(Sgnl)"=w191) -> ()  [unwired: 2 in, 2 out]
          }
        }
      }
      event "Motor stop", "Close 1/4", "Open 1/4", "Motor home": Value Change {
        n86 = event-data() -> ()  [unwired: 1 in, 6 out]
        n87 = Divide(x="Current position", y=10.0) -> (x/y=w210:dbl)
        n88 = Multiply(x=w210, y=100.0) -> (x*y=→"Opening rate (Closed:0, Full open:100)":dbl)
        n89 = Multiply(x="wait for home (s)", y=1000) -> (x*y=w201:dbl)
        n90 = Multiply(x="wait for open/close/stop (s)", y=1000) -> (x*y=w203:dbl)
        n91 = stacked-sequence {
          tunnel: u32 100 ("milliseconds to wait") -> [w213 w254 w293 w322 _]
          tunnel: w203 -> [w212 w253 _ w321 _]
          tunnel: w201 -> [_ _ w290 _ _]
          frame #0 {
            n92 = case shown="True" "Open 1/4" {
              tunnel: "AZD-AZ open" -> [_ w221]
              tunnel: w213 -> [_ w220]
              tunnel: w212 -> [_ w219]
              frame False {
              }
              frame True {
                n93 = local read "Current position"() -> (w218:dbl)
                n94 = Less?(x=w218, y=10.0) -> (x < y?=w216:bool)
                n95 = case shown="False" w216 {
                  tunnel: w221 -> [_ w226]
                  tunnel: w220 -> [_ w225]
                  tunnel: w219 -> [_ w224]
                  frame False {
                    n96 = local write "Open 1/4"(FALSE ("Open 1/4")) -> ()
                    n97 = local write "AZD-AZ status"("Cannot open further!" ("AZD-AZ status")) -> ()
                  }
                  frame True {
                    n98 = flat-sequence {
                      tunnel: w226 -> [w229]
                      tunnel: [w229] -> w228
                      tunnel: w225 -> [w237]
                      tunnel: w228 -> [w236]
                      tunnel: [w236] -> w227
                      tunnel: w227 -> [w239]
                      tunnel: w224 -> [w246]
                      frame #0 {
                        n99 = local read "DOUT6218 Labels"() -> (w234:string[])
                        n100 = local read "DOUT Raw state"() -> (w233:bool[])
                        n101 = Search 1D Array(1D array=w234, element=w229) -> (index of element=w232:i32)  [unwired: 1 in]
                        n102 = Replace Array Subset(array=w233, new element=TRUE ("new element/subarray"), index=w232) -> (w230:bool[])
                        n103 = property on="DOUT Raw state" class="Arr (strict)"("Val(Sgnl)"=w230) -> ()  [unwired: 2 in, 2 out]
                      }
                      frame #1 {
                        n104 = Wait (ms)(milliseconds to wait=w237) -> ()  [unwired: 1 out]
                        n105 = local write "AZD-AZ status"("Command sent \"open 1/4\"" ("AZD-AZ status")) -> ()
                      }
                      frame #2 {
                        n106 = local read "DOUT6218 Labels"() -> (w240:string[])
                        n107 = local read "DOUT Raw state"() -> (w241:bool[])
                        n108 = Search 1D Array(1D array=w240, element=w239) -> (index of element=w242:i32)  [unwired: 1 in]
                        n109 = Replace Array Subset(array=w241, new element=FALSE ("new element/subarray"), index=w242) -> (w244:bool[])
                        n110 = property on="Open 1/4" class="Bool (strict)"("Val(Sgnl)"=FALSE ("Value (Signaling)")) -> ()  [unwired: 2 in, 2 out]
                        n111 = property on="DOUT Raw state" class="Arr (strict)"("Val(Sgnl)"=w244) -> ()  [unwired: 2 in, 2 out]
                      }
                      frame #3 {
                        n112 = local write "AZD-AZ status"("In operation..." ("AZD-AZ status")) -> ()
                        n113 = Wait (ms)(milliseconds to wait=w246) -> ()  [unwired: 1 out]
                      }
                      frame #4 {
                        n114 = property on="Current position" class="DigNum (strict)"() -> ("Value"=w250:dbl)  [unwired: 2 in, 2 out]
                        n115 = Add(x=w250, y=0.25) -> (x+y=w247:dbl)
                        n116 = local write "AZD-AZ status"("Operation complete" ("AZD-AZ status")) -> ()
                        n117 = property on="Current position" class="DigNum (strict)"("Val(Sgnl)"=w247) -> ()  [unwired: 2 in, 2 out]
                      }
                    }
                  }
                }
              }
            }
          }
          frame #1 {
            n118 = case shown="True" "Close 1/4" {
              tunnel: "AZD-AZ close" -> [_ w260]
              tunnel: w254 -> [_ w259]
              tunnel: w253 -> [_ w258]
              frame False {
              }
              frame True {
                n119 = local read "Current position"() -> (w257:dbl)
                n120 = Greater?(x=w257, y=0.0) -> (0:w255:bool)
                n121 = case shown="False" w255 {
                  tunnel: w260 -> [_ w265]
                  tunnel: w259 -> [_ w264]
                  tunnel: w258 -> [_ w263]
                  frame False {
                    n122 = local write "AZD-AZ status"("Cannot close further!" ("AZD-AZ status")) -> ()
                    n123 = local write "Close 1/4"(FALSE ("Value (Signaling)")) -> ()
                  }
                  frame True {
                    n124 = flat-sequence {
                      tunnel: w265 -> [w268]
                      tunnel: [w268] -> w267
                      tunnel: w264 -> [w276]
                      tunnel: w267 -> [w275]
                      tunnel: [w275] -> w266
                      tunnel: w266 -> [w278]
                      tunnel: w263 -> [w285]
                      frame #0 {
                        n125 = local read "DOUT6218 Labels"() -> (w273:string[])
                        n126 = local read "DOUT Raw state"() -> (w272:bool[])
                        n127 = Search 1D Array(1D array=w273, element=w268) -> (index of element=w271:i32)  [unwired: 1 in]
                        n128 = Replace Array Subset(array=w272, new element=TRUE ("new element/subarray"), index=w271) -> (w269:bool[])
                        n129 = property on="DOUT Raw state" class="Arr (strict)"("Val(Sgnl)"=w269) -> ()  [unwired: 2 in, 2 out]
                      }
                      frame #1 {
                        n130 = Wait (ms)(milliseconds to wait=w276) -> ()  [unwired: 1 out]
                        n131 = local write "AZD-AZ status"("Command sent \"close 1/4\"" ("AZD-AZ status")) -> ()
                      }
                      frame #2 {
                        n132 = local read "DOUT6218 Labels"() -> (w279:string[])
                        n133 = local read "DOUT Raw state"() -> (w280:bool[])
                        n134 = Search 1D Array(1D array=w279, element=w278) -> (index of element=w281:i32)  [unwired: 1 in]
                        n135 = Replace Array Subset(array=w280, new element=FALSE ("new element/subarray"), index=w281) -> (w283:bool[])
                        n136 = property on="Close 1/4" class="Bool (strict)"("Val(Sgnl)"=FALSE ("Value (Signaling)")) -> ()  [unwired: 2 in, 2 out]
                        n137 = property on="DOUT Raw state" class="Arr (strict)"("Val(Sgnl)"=w283) -> ()  [unwired: 2 in, 2 out]
                      }
                      frame #3 {
                        n138 = local write "AZD-AZ status"("In operation..." ("AZD-AZ status")) -> ()
                        n139 = Wait (ms)(milliseconds to wait=w285) -> ()  [unwired: 1 out]
                      }
                      frame #4 {
                        n140 = property on="Current position" class="DigNum (strict)"() -> ("Value"=w288:dbl)  [unwired: 2 in, 2 out]
                        n141 = Subtract(x=w288, y=0.25) -> (x-y=w286:dbl)
                        n142 = local write "AZD-AZ status"("Operation complete" ("AZD-AZ status")) -> ()
                        n143 = property on="Current position" class="DigNum (strict)"("Val(Sgnl)"=w286) -> ()  [unwired: 2 in, 2 out]
                      }
                    }
                  }
                }
              }
            }
          }
          frame #2 {
            n144 = case shown="True" "Motor home" {
              tunnel: "AZD-AZ home" -> [_ w298]
              tunnel: w293 -> [_ w297]
              tunnel: w290 -> [_ w294]
              frame False {
              }
              frame True {
                n145 = flat-sequence {
                  tunnel: w298 -> [w299]
                  tunnel: [w299] -> w296
                  tunnel: w297 -> [w307]
                  tunnel: w296 -> [w306]
                  tunnel: [w306] -> w295
                  tunnel: w295 -> [w309]
                  tunnel: w294 -> [w316]
                  frame #0 {
                    n146 = local read "DOUT6218 Labels"() -> (w304:string[])
                    n147 = local read "DOUT Raw state"() -> (w303:bool[])
                    n148 = Search 1D Array(1D array=w304, element=w299) -> (index of element=w302:i32)  [unwired: 1 in]
                    n149 = Replace Array Subset(array=w303, new element=TRUE ("new element/subarray"), index=w302) -> (w300:bool[])
                    n150 = property on="DOUT Raw state" class="Arr (strict)"("Val(Sgnl)"=w300) -> ()  [unwired: 2 in, 2 out]
                  }
                  frame #1 {
                    n151 = Wait (ms)(milliseconds to wait=w307) -> ()  [unwired: 1 out]
                    n152 = local write "AZD-AZ status"("Command sent \"Go home\"" ("AZD-AZ status")) -> ()
                  }
                  frame #2 {
                    n153 = local read "DOUT6218 Labels"() -> (w310:string[])
                    n154 = local read "DOUT Raw state"() -> (w311:bool[])
                    n155 = Search 1D Array(1D array=w310, element=w309) -> (index of element=w312:i32)  [unwired: 1 in]
                    n156 = property on="Motor home" class="Bool (strict)"("Val(Sgnl)"=FALSE ("Value (Signaling)")) -> ()  [unwired: 2 in, 2 out]
                    n157 = Replace Array Subset(array=w311, new element=FALSE ("new element/subarray"), index=w312) -> (w314:bool[])
                    n158 = property on="DOUT Raw state" class="Arr (strict)"("Val(Sgnl)"=w314) -> ()  [unwired: 2 in, 2 out]
                  }
                  frame #3 {
                    n159 = local write "AZD-AZ status"("In operation..." ("AZD-AZ status")) -> ()
                    n160 = Wait (ms)(milliseconds to wait=w316) -> ()  [unwired: 1 out]
                  }
                  frame #4 {
                    n161 = local write "AZD-AZ status"("Operation complete" ("AZD-AZ status")) -> ()
                    n162 = property on="Current position" class="DigNum (strict)"("Val(Sgnl)"=0.0 ("y")) -> ()  [unwired: 2 in, 2 out]
                  }
                }
              }
            }
          }
          frame #3 {
            n163 = case shown="True" "Motor stop" {
              tunnel: "AZD-AZ stop" -> [_ w327]
              tunnel: w322 -> [_ w326]
              tunnel: w321 -> [_ w323]
              frame False {
              }
              frame True {
                n164 = flat-sequence {
                  tunnel: w327 -> [w328]
                  tunnel: [w328] -> w325
                  tunnel: w326 -> [w336]
                  tunnel: w325 -> [w335]
                  tunnel: [w335] -> w324
                  tunnel: w324 -> [w338]
                  tunnel: w323 -> [w345]
                  frame #0 {
                    n165 = local read "DOUT6218 Labels"() -> (w333:string[])
                    n166 = local read "DOUT Raw state"() -> (w332:bool[])
                    n167 = Search 1D Array(1D array=w333, element=w328) -> (index of element=w331:i32)  [unwired: 1 in]
                    n168 = Replace Array Subset(array=w332, new element=TRUE ("new element/subarray"), index=w331) -> (w329:bool[])
                    n169 = property on="DOUT Raw state" class="Arr (strict)"("Val(Sgnl)"=w329) -> ()  [unwired: 2 in, 2 out]
                  }
                  frame #1 {
                    n170 = Wait (ms)(milliseconds to wait=w336) -> ()  [unwired: 1 out]
                    n171 = local write "AZD-AZ status"("Command sent \"Stop\"" ("AZD-AZ status")) -> ()
                  }
                  frame #2 {
                    n172 = local read "DOUT6218 Labels"() -> (w339:string[])
                    n173 = local read "DOUT Raw state"() -> (w340:bool[])
                    n174 = Search 1D Array(1D array=w339, element=w338) -> (index of element=w341:i32)  [unwired: 1 in]
                    n175 = Replace Array Subset(array=w340, new element=FALSE ("new element/subarray"), index=w341) -> (w343:bool[])
                    n176 = property on="Motor stop" class="Bool (strict)"("Val(Sgnl)"=FALSE ("Value (Signaling)")) -> ()  [unwired: 2 in, 2 out]
                    n177 = property on="DOUT Raw state" class="Arr (strict)"("Val(Sgnl)"=w343) -> ()  [unwired: 2 in, 2 out]
                  }
                  frame #3 {
                    n178 = local write "AZD-AZ status"("In operation..." ("AZD-AZ status")) -> ()
                    n179 = Wait (ms)(milliseconds to wait=w345) -> ()  [unwired: 1 out]
                  }
                  frame #4 {
                    n180 = local write "AZD-AZ status"("Operation complete" ("AZD-AZ status")) -> ()
                  }
                }
              }
            }
          }
          frame #4 {
            n181 = local read "Cycle #"() -> (w353:u32)
            n182 = local read "File ref AZD-AX status"() -> (w352:refnum<file>)
            n183 = property on="Current position" class="DigNum (strict)"() -> ("Value"=w350:dbl)  [unwired: 2 in, 2 out]
            n184 = Get Date/Time In Seconds() -> (seconds since 1Jan1904=w351:timestamp)
            n185 = Build Array(w350) -> (w349:dbl[])
            n186 = call "FileWrite.vi"("DataArray"=w349, "Time Stamp"=w351, "Error In"=errorcluster {"status"=FALSE, "code"=0, "source"=""}, "FileFormat"=string[] ["%.2f"], "Index"=w353, "refnum in"=w352) -> ("Error Out"=→"Error Out (AZDAX status)":errorcluster)  [unwired: 4 in, 1 out]
          }
        }
      }
      event "Open N", "Close N": Value Change {
        n187 = event-data() -> ()  [unwired: 1 in, 6 out]
        n188 = property on="Current position" class="DigNum (strict)"() -> ("Value"=w355:dbl)  [unwired: 2 in, 2 out]
        n189 = Divide(x=w355, y=10.0) -> (x/y=w362:dbl)
        n190 = Multiply(x=w362, y=100.0) -> (x*y=w356:dbl)
        n191 = property on="Opening rate (Closed:0, Full open:100)" class="Knob (strict)"("Val(Sgnl)"=w356) -> ()  [unwired: 2 in, 2 out]
        n192 = local read "wait for open/close/stop (s)"() -> (w357:dbl)
        n193 = Multiply(x=w357, y=1000) -> (x*y=w358:dbl)
        n194 = stacked-sequence {
          tunnel: u32 100 ("milliseconds to wait") -> [w370 w435]
          tunnel: w358 -> [w369 w434]
          frame #0 {
            n195 = local read "AZD-AZ open"() -> (w364:string)
            n196 = Multiply(x="N to open", y=u64 4) -> (x*y=w365:u64)
            n197 = case shown="True" "Open N" {
              tunnel: w364 -> [_ w380]
              tunnel: w370 -> [_ w379]
              tunnel: w369 -> [_ w378]
              tunnel: w365 -> [_ w374]
              frame False {
              }
              frame True {
                n198 = property on="Current position" class="DigNum (strict)"() -> ("Value"=w377:dbl)  [unwired: 2 in, 2 out]
                n199 = Multiply(x=0.25, y=w374) -> (x*y=w376:dbl)
                n200 = Add(x=w377, y=w376) -> (x+y=w373:dbl)
                n201 = Less Or Equal?(x=w373, y=9.9) -> (x <= y?=w371:bool)
                "Open Command accepted" <- w371
                n202 = case shown="False" w371 {
                  tunnel: w380 -> [_ w386]
                  tunnel: w379 -> [_ w385]
                  tunnel: w378 -> [_ w384]
                  tunnel: w374 -> [_ w383]
                  frame False {
                    n203 = local write "AZD-AZ status"("Cannot open further!" ("AZD-AZ status")) -> ()
                    n204 = local write "Open N"(FALSE ("Close N")) -> ()
                  }
                  frame True {
                    n205 = for {
                      N: w383 -> [w394]
                      tunnel: w386 -> [w399]
                      tunnel: w385 -> [w398]
                      tunnel: w384 -> [w397]
                      i -> [w396]
                      (unwired) errorcluster {"status"=FALSE, "code"=0, "source"=""} ("Error In")
                      n206 = stacked-sequence {
                        tunnel: w399 -> [w400 _ w408 _ _]
                        tunnel: w398 -> [_ w407 _ _ _]
                        tunnel: w396 -> [_ _ w413 _ _]
                        tunnel: w394 -> [_ _ w412 _ _]
                        tunnel: w397 -> [_ _ _ w421 _]
                        tunnel: [_ _ _ _ w425] -> w389
                        frame #0 {
                          n207 = local read "DOUT6218 Labels"() -> (w405:string[])
                          n208 = local read "DOUT Raw state"() -> (w404:bool[])
                          n209 = Search 1D Array(1D array=w405, element=w400) -> (index of element=w403:i32)  [unwired: 1 in]
                          n210 = Replace Array Subset(array=w404, new element=TRUE ("new element/subarray"), index=w403) -> (w401:bool[])
                          n211 = property on="DOUT Raw state" class="Arr (strict)"("Val(Sgnl)"=w401) -> ()  [unwired: 2 in, 2 out]
                        }
                        frame #1 {
                          n212 = Wait (ms)(milliseconds to wait=w407) -> ()  [unwired: 1 out]
                          n213 = local write "AZD-AZ status"("Command sent \"open 1/4\"" ("AZD-AZ status")) -> ()
                        }
                        frame #2 {
                          n214 = Subtract(x=w412, y=1) -> (x-y=w410:i32)
                          n215 = local read "DOUT6218 Labels"() -> (w414:string[])
                          n216 = Equal?(x=w413, y=w410) -> (x = y?=w409:bool)
                          n217 = case shown="True" w409 {
                            frame False {
                            }
                            frame True {
                              n218 = property on="Open N" class="Bool (strict)"("Val(Sgnl)"=FALSE ("Value (Signaling)")) -> ()  [unwired: 2 in, 2 out]
                            }
                          }
                          n219 = local read "DOUT Raw state"() -> (w415:bool[])
                          n220 = Search 1D Array(1D array=w414, element=w408) -> (index of element=w416:i32)  [unwired: 1 in]
                          n221 = Replace Array Subset(array=w415, new element=FALSE ("new element/subarray"), index=w416) -> (w418:bool[])
                          n222 = property on="DOUT Raw state" class="Arr (strict)"("Val(Sgnl)"=w418) -> ()  [unwired: 2 in, 2 out]
                        }
                        frame #3 {
                          n223 = local write "AZD-AZ status"("In operation..." ("AZD-AZ status")) -> ()
                          n224 = Wait (ms)(milliseconds to wait=w421) -> ()  [unwired: 1 out]
                        }
                        frame #4 {
                          n225 = property on="Current position" class="DigNum (strict)"() -> ("Value"=w426:dbl)  [unwired: 2 in, 2 out]
                          n226 = property on="Opening rate (Closed:0, Full open:100)" class="Knob (strict)"() -> ("Value"=w423:dbl)  [unwired: 2 in, 2 out]
                          n227 = Add(x=w423, y=2.5) -> (x+y=w422:dbl)
                          n228 = Add(x=w426, y=0.25) -> (x+y=w425:dbl)
                          n229 = local write "AZD-AZ status"("Operation complete" ("AZD-AZ status")) -> ()
                          n230 = property on="Current position" class="DigNum (strict)"("Val(Sgnl)"=w425) -> ()  [unwired: 2 in, 2 out]
                          n231 = property on="Opening rate (Closed:0, Full open:100)" class="Knob (strict)"("Val(Sgnl)"=w422) -> ()  [unwired: 2 in, 2 out]
                        }
                      }
                      n232 = Subtract(x=w394, y=w396) -> (x-y=w395:i32)
                      n233 = local write "... more steps"(w395) -> ()
                      n234 = local read "Cycle #"() -> (w393:u32)
                      n235 = local read "File ref AZD-AX status"() -> (w392:refnum<file>)
                      n236 = Get Date/Time In Seconds() -> (seconds since 1Jan1904=w391:timestamp)
                      n237 = Build Array(w389) -> (w388:dbl[])
                      n238 = call "FileWrite.vi"("DataArray"=w388, "Time Stamp"=w391, "FileFormat"=string[] ["%.2f"], "Index"=w393, "refnum in"=w392) -> ("Error Out"=w390:errorcluster)  [unwired: 5 in, 1 out]
                      n239 = local write "Error Out (AZDAX status)"(w390) -> ()
                    }
                  }
                }
              }
            }
          }
          frame #1 {
            n240 = local read "AZD-AZ close"() -> (w433:string)
            n241 = Multiply(x="N to close", y=u64 4) -> (x*y=w429:u64)
            n242 = case shown="True" "Close N" {
              tunnel: w433 -> [_ w446]
              tunnel: w435 -> [_ w445]
              tunnel: w434 -> [_ w444]
              tunnel: w429 -> [_ w443]
              tunnel: w429 -> [_ w441]
              frame False {
              }
              frame True {
                n243 = property on="Current position" class="DigNum (strict)"() -> ("Value"=w439:dbl)  [unwired: 2 in, 2 out]
                n244 = Multiply(x=0.25, y=w441) -> (x*y=w440:dbl)
                n245 = Subtract(x=w439, y=w440) -> (x-y=w438:dbl)
                n246 = Greater Or Equal?(x=w438, y=0.0) -> (x >= y?=w436:bool)
                "Close Command accepted" <- w436
                n247 = case shown="False" w436 {
                  tunnel: w446 -> [_ w452]
                  tunnel: w445 -> [_ w451]
                  tunnel: w444 -> [_ w450]
                  tunnel: w443 -> [_ w449]
                  frame False {
                    n248 = local write "Close N"(FALSE ("Close N")) -> ()
                    n249 = local write "AZD-AZ status"("Cannot close further!" ("AZD-AZ status")) -> ()
                  }
                  frame True {
                    n250 = flat-sequence {
                      tunnel: w452 -> [w456]
                      tunnel: w451 -> [w455]
                      tunnel: w450 -> [w454]
                      tunnel: w449 -> [w453]
                      frame #0 {
                        n251 = for {
                          N: w453 -> [w468]
                          tunnel: w456 -> [w457]
                          tunnel: w455 -> [w471]
                          tunnel: w454 -> [w470]
                          i -> [w466]
                          n252 = Subtract(x=w468, y=w466) -> (x-y=w467:i32)
                          n253 = stacked-sequence {
                            tunnel: w471 -> [_ w479 _ _ _]
                            tunnel: w468 -> [_ _ w484 _ _]
                            tunnel: w467 -> [_ _ _ _ _]
                            tunnel: w466 -> [_ _ w482 _ _]
                            tunnel: w470 -> [_ _ _ w493 _]
                            tunnel: [_ _ _ _ w497] -> w460
                            tunnel: w457 -> [w472 _ w480 _ _]
                            frame #0 {
                              n254 = local read "DOUT6218 Labels"() -> (w477:string[])
                              n255 = local read "DOUT Raw state"() -> (w476:bool[])
                              n256 = Search 1D Array(1D array=w477, element=w472) -> (index of element=w475:i32)  [unwired: 1 in]
                              n257 = Replace Array Subset(array=w476, new element=TRUE ("new element/subarray"), index=w475) -> (w473:bool[])
                              n258 = property on="DOUT Raw state" class="Arr (strict)"("Val(Sgnl)"=w473) -> ()  [unwired: 2 in, 2 out]
                            }
                            frame #1 {
                              n259 = local write "AZD-AZ status"("Command sent \"close 1/4\"" ("AZD-AZ status")) -> ()
                              n260 = Wait (ms)(milliseconds to wait=w479) -> ()  [unwired: 1 out]
                            }
                            frame #2 {
                              n261 = local read "DOUT6218 Labels"() -> (w487:string[])
                              n262 = local read "DOUT Raw state"() -> (w488:bool[])
                              n263 = Search 1D Array(1D array=w487, element=w480) -> (index of element=w489:i32)  [unwired: 1 in]
                              n264 = Replace Array Subset(array=w488, new element=FALSE ("new element/subarray"), index=w489) -> (w490:bool[])
                              n265 = property on="DOUT Raw state" class="Arr (strict)"("Val(Sgnl)"=w490) -> ()  [unwired: 2 in, 2 out]
                              n266 = Subtract(x=w484, y=1) -> (x-y=w483:i32)
                              n267 = Equal?(x=w482, y=w483) -> (x = y?=w481:bool)
                              n268 = case shown="True" w481 {
                                frame False {
                                }
                                frame True {
                                n269 = property on="Close N" class="Bool (strict)"("Val(Sgnl)"=FALSE ("new element/subarray")) -> ()  [unwired: 2 in, 2 out]
                                }
                              }
                            }
                            frame #3 {
                              n270 = local write "AZD-AZ status"("In operation..." ("AZD-AZ status")) -> ()
                              n271 = Wait (ms)(milliseconds to wait=w493) -> ()  [unwired: 1 out]
                            }
                            frame #4 {
                              n272 = property on="Current position" class="DigNum (strict)"() -> ("Value"=w498:dbl)  [unwired: 2 in, 2 out]
                              n273 = property on="Opening rate (Closed:0, Full open:100)" class="Knob (strict)"() -> ("Value"=w495:dbl)  [unwired: 2 in, 2 out]
                              n274 = Subtract(x=w495, y=2.5) -> (x-y=w496:dbl)
                              n275 = Subtract(x=w498, y=0.25) -> (x-y=w497:dbl)
                              n276 = local write "AZD-AZ status"("Operation complete" ("AZD-AZ status")) -> ()
                              n277 = property on="Current position" class="DigNum (strict)"("Val(Sgnl)"=w497) -> ()  [unwired: 2 in, 2 out]
                              n278 = property on="Opening rate (Closed:0, Full open:100)" class="Knob (strict)"("Val(Sgnl)"=w496) -> ()  [unwired: 2 in, 2 out]
                            }
                          }
                          n279 = local write "... more steps"(w467) -> ()
                          n280 = Wait (ms)(milliseconds to wait=u32 5) -> ()  [unwired: 1 out]
                          n281 = local read "File ref AZD-AX status"() -> (w464:refnum<file>)
                          n282 = local read "Cycle #"() -> (w465:u32)
                          n283 = Get Date/Time In Seconds() -> (seconds since 1Jan1904=w463:timestamp)
                          n284 = Build Array(w460) -> (w459:dbl[])
                          n285 = call "FileWrite.vi"("DataArray"=w459, "Time Stamp"=w463, "Error In"=errorcluster {"status"=FALSE, "code"=0, "source"=""}, "FileFormat"=string[] ["%.2f"], "Index"=w465, "refnum in"=w464) -> ("Error Out"=w458:errorcluster)  [unwired: 4 in, 1 out]
                          n286 = local write "Error Out (AZDAX status)"(w458) -> ()
                        }
                      }
                      frame #1 {
                        n287 = local write "... more steps"(u64 1 ("... more steps")) -> ()
                      }
                    }
                  }
                }
              }
            }
          }
        }
      }
    }
    n288 = Bundle(w48, w45) -> (w47:cluster{timestamp[], dbl[]})  [unwired: 1 in]
    n289 = Build Array(w47, w44) -> (→"Graph 7":T10)
  }
  n290 = while {
    i -> [w505]
    stop <- w507 stop-if-true
    n291 = local read "DOUT6218 Labels"() -> (w502:string[])
    "DOUT Labels 2" <- w502
    n292 = Wait (ms)(milliseconds to wait=u32 99) -> ()  [unwired: 1 out]
    n293 = Equal?(x=w505, y=0) -> (x = y?=w503:bool)
    n294 = case shown="True" w503 {
      tunnel: w502 -> [_ w510]
      frame False {
      }
      frame True {
        n295 = Array Size(array=w510) -> (size(s)=w509:i32)
        n296 = for {
          N: w509 -> [_]
          tunnel: [FALSE] -> w508 mode=indexing
        }
        n297 = property on="DOUT Raw state" class="Arr (strict)"("Val(Sgnl)"=w508) -> ()  [unwired: 2 in, 2 out]
      }
    }
    n298 = event shown="[2] \"DOUT Raw state\": Value Change" {
      selector: _ -> [_ _ _]
      dyn-events: _ -> [_ _ _]
      timeout: _ -> [_ _ _]
      tunnel: [FALSE TRUE w519] -> w507
      tunnel: w502 -> [_ _ w514]
      event Timeout {
        n299 = event-data() -> ()  [unwired: 1 in, 3 out]
      }
      event "Stop Button": Value Change {
        n300 = event-data() -> ()  [unwired: 1 in, 3 out]
      }
      event "DOUT Raw state": Value Change {
        n301 = event-data() -> ()  [unwired: 1 in, 3 out]
        n302 = local read "Cycle #"() -> (w516:u32)
        n303 = Greater?(x=w516, y=u32 0) -> (0:w517:bool)
        n304 = case shown="True" w517 {
          tunnel: [FALSE FALSE] -> w519
          tunnel: w516 -> [_ w525]
          tunnel: "DOUT Raw state" -> [_ w524]
          tunnel: "DOUT Raw state" -> [_ w523]
          tunnel: w514 -> [_ w522]
          frame False {
          }
          frame True {
            n305 = local read "error out (USB6210/6218 DOUT)"() -> (w528:errorcluster)
            n306 = local read "DOUT task out"() -> (w527:refnum<k21>)
            n307 = Array Size(array=w522) -> (size(s)=w521:i32)
            n308 = local read "File Refn USB DO"() -> (w536:refnum<file>)
            n309 = Boolean To (0,1)(Boolean=w524) -> (0, 1=w538:i16[])
            n310 = call <vilib>:"DAQmx Write (Digital 1D Bool NChan 1Samp 1Line).vi"("task/channels in"=w527, "data"=w523, "timeout"=10.0, "error in"=w528) -> ("task out"=w530:refnum<k21>, "error out"=w532:errorcluster)  [unwired: 9 in, 1 out]
            n311 = Initialize Array("%d" ("element"), w521) -> (w534:string[])
            n312 = local write "DOUT task out"(w530) -> ()
            n313 = Get Date/Time In Seconds() -> (seconds since 1Jan1904=w535:timestamp)
            n314 = call "FileWrite.vi"("DataArray"=w538, "Time Stamp"=w535, "Error In"=w532, "FileFormat"=w534, "Index"=w525, "refnum in"=w536) -> ("Error Out"=w533:errorcluster, "Byte Stream File Refnum"=w537:refnum<file>)  [unwired: 4 in]
            n315 = local write "File Refn USB DO"(w537) -> ()
            n316 = local write "error out (USB6210/6218 DOUT)"(w533) -> ()
          }
        }
      }
    }
  }
  n317 = while {
    shift-right: [w547] -> _
    shift-left: refnum<class "6240AData.lvclass"> refnum ("6240AData.lvclass") -> [w545]
    shift-right: [w543] -> _
    shift-left: errorcluster {"status"=FALSE, "code"=0, "source"=""} ("error in (no error)") -> [w544]
    i -> [w539]
    stop <- w546 stop-if-true
    n318 = Wait (ms)(milliseconds to wait=u32 231) -> ()  [unwired: 1 out]
    n319 = Equal?(x=w539, y=0) -> (x = y?=w541:bool)
    n320 = case shown="True" w541 {
      frame False {
      }
      frame True {
        n321 = property on="Initialized?" class="Bool (strict)"("Val(Sgnl)"=FALSE ("Value (Signaling)")) -> ()  [unwired: 2 in, 2 out]
      }
    }
    n322 = event shown="[1] \"update values\", \"SetCurrent 1 (mA)\", \"SetCurrent 2 (mA)\": Value Change" {
      selector: _ -> [_ _ _ _ _]
      dyn-events: _ -> [_ _ _ _ _]
      timeout: _ -> [_ _ _ _ _]
      tunnel: [w550 w565 _ w614 w635] -> w547
      tunnel: [_ _ _ _ TRUE ("Value (Signaling)")] -> w546
      tunnel: w545 -> [w550 w564 _ w598 w633]
      tunnel: w544 -> [w549 w563 _ w597 w631]
      tunnel: [w549 w562 _ w612 w634] -> w543
      tunnel: w539 -> [_ w561 _ _ _]
      tunnel: w539 -> [_ _ _ w606 _]
      event Timeout {
        n323 = event-data() -> ()  [unwired: 1 in, 3 out]
      }
      event "update values", "SetCurrent 1 (mA)", "SetCurrent 2 (mA)": Value Change {
        w554 = 1000.0 ("y")
        n324 = event-data() -> ()  [unwired: 1 in, 6 out]
        n325 = local read "Initialized?"() -> (w560:bool)
        n326 = Divide(x="SetCurrent 1 (mA)", y=w554) -> (x/y=w555:dbl)
        n327 = Divide(x="SetCurrent 2 (mA)", y=w554) -> (x/y=w556:dbl)
        n328 = Build Array(w555, w556) -> (w553:dbl[])
        n329 = Not Equal?(x=w560, y=FALSE) -> (x != y?=w558:bool)
        n330 = case shown="True" w558 {
          tunnel: [w567 w591] -> w565
          tunnel: "Output\n (ADCMT)" -> [_ w590]
          tunnel: w564 -> [w567 w589]
          tunnel: w563 -> [w566 w588]
          tunnel: [w566 w587] -> w562
          tunnel: w561 -> [_ w583]
          tunnel: w553 -> [_ w569]
          frame False {
          }
          frame True {
            w576 = 1 ("index (col)")
            w577 = 0 ("disabled index (col)")
            n331 = call-dynamic "6240AData_execute.vi"("6240AData in"=w589, "SetCurrent (A)"=w569, "FileFormat"="%3.5f", "Output status"=w590, "ExecutionIndex"=w583, "error in (no error)"=w588) -> ("ActualVoltage (V)"=w568:dbl[], "ActualCurrent (A)"=w582:dbl[], "6240AData out"=w591:refnum<class "6240AData.lvclass">, "appended array"=w572:timestamp[], "SetCurrentArray"=w578:dbl[][], "ActualCurrentArray"=w585:dbl[][], "error out"=w587:errorcluster)  [unwired: 3 in]
            n332 = property on="ActualVoltage (V)" class="Arr (strict)"("Val(Sgnl)"=w568) -> ()  [unwired: 2 in, 2 out]
            n333 = property on="ActualCurrent (A)" class="Arr (strict)"("Val(Sgnl)"=w582) -> ()  [unwired: 2 in, 2 out]
            n334 = Index Array(array=w585, index (col) #1=w577, index (col) #2=w576) -> (element #1=w586:dbl[], element #2=w580:dbl[])  [unwired: 2 in]
            n335 = Index Array(array=w578, index (col) #1=w577, index (col) #2=w576) -> (element #1=w574:dbl[], element #2=w571:dbl[])  [unwired: 2 in]
            n336 = Bundle("appended array"=w572, "ActualCurrentArray"=w586) -> (w581:T21)  [unwired: 1 in]
            n337 = Bundle("appended array"=w572, "ActualCurrentArray"=w580) -> (w575:T21)  [unwired: 1 in]
            n338 = Bundle("appended array"=w572, "SetCurrentArray"=w574) -> (w573:T22)  [unwired: 1 in]
            n339 = Bundle("appended array"=w572, "SetCurrentArray"=w571) -> (w570:T22)  [unwired: 1 in]
            n340 = Build Array(w581, w575, w573, w570) -> (→"Graph 6":T23)
          }
        }
      }
      event "upper limit (mA)", "lower limit (mA)": Value Change {
        n341 = event-data() -> ()  [unwired: 1 in, 6 out]
        n342 = property on="SetCurrent 1 (mA)" class="DigNum (strict)"("Maximum"="upper limit (mA)", "Minimum"="lower limit (mA)") -> ()  [unwired: 2 in, 2 out]
        n343 = property on="SetCurrent 2 (mA)" class="DigNum (strict)"("Maximum"="upper limit (mA)", "Minimum"="lower limit (mA)") -> ()  [unwired: 2 in, 2 out]
      }
      event "Initialize": Value Change {
        w608 = FALSE
        n344 = event-data() -> ()  [unwired: 1 in, 6 out]
        n345 = local read "Initialized?"() -> (w596:bool)
        n346 = case shown="True" w596 {
          tunnel: w598 -> [w624 w628]
          tunnel: w597 -> [w623 w627]
          tunnel: [w624 w626] -> w595
          tunnel: [w623 w625] -> w594
          frame False {
          }
          frame True {
            n347 = call-dynamic "6240AData_terrminate.vi"("error in (no error)"=w627, "6240AData in"=w628) -> ("error out"=w625:errorcluster, "6240AData out"=w626:refnum<class "6240AData.lvclass">)  [unwired: 8 in]
          }
        }
        n348 = property on="Initialized?" class="Bool (strict)"("Val(Sgnl)"=TRUE ("Value (Signaling)")) -> ()  [unwired: 2 in, 2 out]
        n349 = local read "SetCurrent 2 (mA)"() -> (w601:dbl)
        n350 = local read "SetCurrent 1 (mA)"() -> (w604:dbl)
        n351 = local read "RUN Identifier"() -> (w616:string)
        n352 = local read "Base Path"() -> (w617:path)
        n353 = Divide(x=w604, y=1000.0) -> (x/y=w603:dbl)
        n354 = Divide(x=w601, y=1000.0) -> (x/y=w600:dbl)
        n355 = Get Date/Time In Seconds() -> ()  [unwired: 1 out]
        n356 = call-dynamic "6240AData_initialize.vi"("6240AData in"=w595, "RunIdentifier"=w616, "InstName"="InstName", "base path"=w617, "VISA"="VISA", "error in (no error)"=w594, "CtrlLabels"="CtrlLabels", "Voltage limits (V)"="Voltage limits (V)") -> ("6240AData out"=w615:refnum<class "6240AData.lvclass">, "error out"=w613:errorcluster)  [unwired: 6 in]
        n357 = Build Array(w603, w600) -> (w599:dbl[])
        n358 = Build Array(w608, w608) -> (w607:bool[])
        n359 = call-dynamic "6240AData_execute.vi"("6240AData in"=w615, "SetCurrent (A)"=w599, "FileFormat"="%3.5f", "Output status"=w607, "ExecutionIndex"=w606, "error in (no error)"=w613) -> ("ActualVoltage (V)"=w610:dbl[], "ActualCurrent (A)"=w609:dbl[], "6240AData out"=w614:refnum<class "6240AData.lvclass">, "error out"=w612:errorcluster)  [unwired: 3 in, 3 out]
        n360 = property on="ActualVoltage (V)" class="Arr (strict)"("Val(Sgnl)"=w610) -> ()  [unwired: 2 in, 2 out]
        n361 = property on="ActualCurrent (A)" class="Arr (strict)"("Val(Sgnl)"=w609) -> ()  [unwired: 2 in, 2 out]
      }
      event "Stop Button": Value Change {
        n362 = event-data() -> ()  [unwired: 1 in, 6 out]
        n363 = local read "Initialized?"() -> (w629:bool)
        n364 = case shown="False" w629 {
          tunnel: w633 -> [w638 w650]
          tunnel: [w638 w649] -> w632
          tunnel: w631 -> [w637 w648]
          tunnel: [w637 w647] -> w630
          frame False {
          }
          frame True {
            w654 = FALSE
            n365 = local read "SetCurrent 2 (mA)"() -> (w640:dbl)
            n366 = local read "SetCurrent 1 (mA)"() -> (w644:dbl)
            n367 = Divide(x=w644, y=1000.0) -> (x/y=w642:dbl)
            n368 = Divide(x=w640, y=1000.0) -> (x/y=w639:dbl)
            n369 = Build Array(w642, w639) -> (w646:dbl[])
            n370 = Build Array(w654, w654) -> (w645:bool[])
            n371 = property on="Output\n (ADCMT)" class="Arr (strict)"("Val(Sgnl)"=w645) -> ()  [unwired: 2 in, 2 out]
            n372 = call-dynamic "6240AData_execute.vi"("6240AData in"=w650, "SetCurrent (A)"=w646, "FileFormat"="%3.5f", "Output status"=w645, "error in (no error)"=w648) -> ("ActualVoltage (V)"=w651:dbl[], "ActualCurrent (A)"=w652:dbl[], "6240AData out"=w649:refnum<class "6240AData.lvclass">, "error out"=w647:errorcluster)  [unwired: 4 in, 3 out]
            n373 = property on="ActualVoltage (V)" class="Arr (strict)"("Val(Sgnl)"=w651) -> ()  [unwired: 2 in, 2 out]
            n374 = property on="ActualCurrent (A)" class="Arr (strict)"("Val(Sgnl)"=w652) -> ()  [unwired: 2 in, 2 out]
          }
        }
        n375 = call-dynamic "6240AData_terrminate.vi"("error in (no error)"=w630, "6240AData in"=w632) -> ("error out"=w634:errorcluster, "6240AData out"=w635:refnum<class "6240AData.lvclass">)  [unwired: 8 in]
      }
    }
    "error out (ADCMT6420A)" <- w543
  }
  n376 = while {
    stop <- w663 stop-if-true
    n377 = Get Date/Time In Seconds() -> (seconds since 1Jan1904=w662:timestamp)
    n378 = Format Date/Time String(time format string (%c)="%Y%m", seconds (now)=w662) -> (date/time string=w659:string)  [unwired: 1 in]
    n379 = Build Path(base path="Base Path (screenshots)", name or relative path=w659) -> (appended path=w658:path)
    n380 = Create Folder(path (use dialog)=w658, error in=errorcluster {"status"=FALSE, "code"=0, "source"=""}) -> (created path=w655:path, error out=→"error out (monthly folder creation)":errorcluster)  [unwired: 1 in, 1 out]
    n381 = event shown="[1] \"Frontpanel screenshots\": Value Change" {
      selector: _ -> [_ _ _]
      dyn-events: _ -> [_ _ _]
      timeout: _ -> [_ _ _]
      tunnel: [FALSE _ TRUE] -> w663
      tunnel: w655 -> [_ w671 _]
      tunnel: w662 -> [_ w670 _]
      event Timeout {
        n382 = event-data() -> ()  [unwired: 1 in, 3 out]
      }
      event "Frontpanel screenshots": Value Change {
        n383 = event-data() -> ()  [unwired: 1 in, 3 out]
        n384 = property class="TabCtl (strict)"() -> ("Value"=w668:T1)  [unwired: 2 in, 2 out]
        n385 = stacked-sequence {
          tunnel: w671 -> [w677 w699 w721 w743 w765 w787 w809 w831 w853 _]
          tunnel: w670 -> [w676 w698 w720 w742 w764 w786 w808 w830 w852 _]
          tunnel: [w674 _ _ _ _ _ _ _ _ _] -> w669
          tunnel: w668 -> [w673 _ _ _ _ _ _ _ _ _]
          tunnel: [w673 _ _ _ _ _ _ _ _ _] -> w667
          tunnel: "cryostatus_" ("string") -> [w672 w695 w717 w739 w761 w783 w805 w827 w849 _]
          frame #0 {
            n386 = flat-sequence {
              tunnel: w676 -> [w679]
              tunnel: [w679] -> w675
              tunnel: w677 -> [w694]
              tunnel: w675 -> [w682]
              tunnel: [w681] -> w674
              tunnel: w672 -> [w680]
              frame #0 {
                n387 = property class="TabCtl (strict)"("Val(Sgnl)"=T1."NI USB CONFIG" ("Value (Signaling)")) -> ()  [unwired: 2 in, 2 out]
              }
              frame #1 {
                w692 = "_" ("string")
                n388 = local read "Cycle #"() -> (w690:u32)
                n389 = call "LV_UNIXTIME.vi"("current time"=w682) -> ("date/time string"=w693:string)  [unwired: 9 in, 1 out]
                n390 = Format Value(format string="%06d", value (0)=w690) -> (output string=w689:string)  [unwired: 1 in]
                n391 = Concatenate Strings(w680, w693, w692, w689, w692, "page1.png" ("string")) -> (w687:string)
                n392 = invoke class="TabCtl (strict)" method="Get Image"(error in=errorcluster {"status"=FALSE, "code"=0, "source"=""} ("error in (no error)")) -> (error out=w683:errorcluster, "image data"=w685:T24)  [unwired: 5 in, 4 out]
                n393 = Build Path(base path=w694, name or relative path=w687) -> (appended path=w686:path)
                n394 = call <vilib>:"Write PNG File.vi"("error in (no error)"=w683, "image data"=w685, "path to PNG file"=w686) -> ("error out"=w681:errorcluster)  [unwired: 7 in, 1 out]
              }
            }
          }
          frame #1 {
            n395 = flat-sequence {
              tunnel: w698 -> [w701]
              tunnel: [w701] -> w697
              tunnel: w699 -> [w716]
              tunnel: w697 -> [w704]
              tunnel: [w703] -> w696
              tunnel: w695 -> [w702]
              frame #0 {
                n396 = property class="TabCtl (strict)"("Val(Sgnl)"=T1."NI USB CONFIG" ("Value (Signaling)")) -> ()  [unwired: 2 in, 2 out]
              }
              frame #1 {
                w714 = "_" ("string")
                n397 = local read "Cycle #"() -> (w712:u32)
                n398 = call "LV_UNIXTIME.vi"("current time"=w704) -> ("date/time string"=w715:string)  [unwired: 9 in, 1 out]
                n399 = Format Value(format string="%06d", value (0)=w712) -> (output string=w711:string)  [unwired: 1 in]
                n400 = Concatenate Strings(w702, w715, w714, w711, w714, "page2.png" ("string")) -> (w709:string)
                n401 = invoke class="TabCtl (strict)" method="Get Image"(error in=errorcluster {"status"=FALSE, "code"=0, "source"=""} ("error in (no error)")) -> (error out=w705:errorcluster, "image data"=w707:T24)  [unwired: 5 in, 4 out]
                n402 = Build Path(base path=w716, name or relative path=w709) -> (appended path=w708:path)
                n403 = call <vilib>:"Write PNG File.vi"("error in (no error)"=w705, "image data"=w707, "path to PNG file"=w708) -> ("error out"=w703:errorcluster)  [unwired: 7 in, 1 out]
              }
            }
            n404 = local write "error out (frontpanel screenshots)"(w696) -> ()
          }
          frame #2 {
            n405 = flat-sequence {
              tunnel: w720 -> [w723]
              tunnel: [w723] -> w719
              tunnel: w721 -> [w738]
              tunnel: w719 -> [w726]
              tunnel: [w725] -> w718
              tunnel: w717 -> [w724]
              frame #0 {
                n406 = property class="TabCtl (strict)"("Val(Sgnl)"=T1."MEASUREMENT" ("Value (Signaling)")) -> ()  [unwired: 2 in, 2 out]
              }
              frame #1 {
                w736 = "_" ("string")
                n407 = local read "Cycle #"() -> (w734:u32)
                n408 = Format Value(format string="%06d", value (0)=w734) -> (output string=w733:string)  [unwired: 1 in]
                n409 = call "LV_UNIXTIME.vi"("current time"=w726) -> ("date/time string"=w737:string)  [unwired: 9 in, 1 out]
                n410 = Concatenate Strings(w724, w737, w736, w733, w736, "page3.png" ("string")) -> (w731:string)
                n411 = invoke class="TabCtl (strict)" method="Get Image"(error in=errorcluster {"status"=FALSE, "code"=0, "source"=""} ("error in (no error)")) -> (error out=w727:errorcluster, "image data"=w729:T24)  [unwired: 5 in, 4 out]
                n412 = Build Path(base path=w738, name or relative path=w731) -> (appended path=w730:path)
                n413 = call <vilib>:"Write PNG File.vi"("error in (no error)"=w727, "image data"=w729, "path to PNG file"=w730) -> ("error out"=w725:errorcluster)  [unwired: 7 in, 1 out]
              }
            }
            n414 = local write "error out (frontpanel screenshots)"(w718) -> ()
          }
          frame #3 {
            n415 = flat-sequence {
              tunnel: w742 -> [w745]
              tunnel: [w745] -> w741
              tunnel: w743 -> [w760]
              tunnel: w741 -> [w748]
              tunnel: [w747] -> w740
              tunnel: w739 -> [w746]
              frame #0 {
                n416 = property class="TabCtl (strict)"("Val(Sgnl)"=T1."HE AUTO FILL" ("Value (Signaling)")) -> ()  [unwired: 2 in, 2 out]
              }
              frame #1 {
                w758 = "_" ("string")
                n417 = local read "Cycle #"() -> (w756:u32)
                n418 = Format Value(format string="%06d", value (0)=w756) -> (output string=w755:string)  [unwired: 1 in]
                n419 = call "LV_UNIXTIME.vi"("current time"=w748) -> ("date/time string"=w759:string)  [unwired: 9 in, 1 out]
                n420 = Concatenate Strings(w746, w759, w758, w755, w758, "page4.png" ("string")) -> (w753:string)
                n421 = invoke class="TabCtl (strict)" method="Get Image"(error in=errorcluster {"status"=FALSE, "code"=0, "source"=""} ("error in (no error)")) -> (error out=w749:errorcluster, "image data"=w751:T24)  [unwired: 5 in, 4 out]
                n422 = Build Path(base path=w760, name or relative path=w753) -> (appended path=w752:path)
                n423 = call <vilib>:"Write PNG File.vi"("error in (no error)"=w749, "image data"=w751, "path to PNG file"=w752) -> ("error out"=w747:errorcluster)  [unwired: 7 in, 1 out]
              }
            }
            n424 = local write "error out (frontpanel screenshots)"(w740) -> ()
          }
          frame #4 {
            n425 = flat-sequence {
              tunnel: w764 -> [w767]
              tunnel: [w767] -> w763
              tunnel: w765 -> [w782]
              tunnel: w763 -> [w770]
              tunnel: [w769] -> w762
              tunnel: w761 -> [w768]
              frame #0 {
                n426 = property class="TabCtl (strict)"("Val(Sgnl)"=T1."VALVE/HEATER CTRL" ("Value (Signaling)")) -> ()  [unwired: 2 in, 2 out]
              }
              frame #1 {
                w780 = "_" ("string")
                n427 = local read "Cycle #"() -> (w778:u32)
                n428 = call "LV_UNIXTIME.vi"("current time"=w770) -> ("date/time string"=w781:string)  [unwired: 9 in, 1 out]
                n429 = Format Value(format string="%06d", value (0)=w778) -> (output string=w777:string)  [unwired: 1 in]
                n430 = Concatenate Strings(w768, w781, w780, w777, w780, "page5.png" ("string")) -> (w775:string)
                n431 = invoke class="TabCtl (strict)" method="Get Image"(error in=errorcluster {"status"=FALSE, "code"=0, "source"=""} ("error in (no error)")) -> (error out=w771:errorcluster, "image data"=w773:T24)  [unwired: 5 in, 4 out]
                n432 = Build Path(base path=w782, name or relative path=w775) -> (appended path=w774:path)
                n433 = call <vilib>:"Write PNG File.vi"("error in (no error)"=w771, "image data"=w773, "path to PNG file"=w774) -> ("error out"=w769:errorcluster)  [unwired: 7 in, 1 out]
              }
            }
            n434 = local write "error out (frontpanel screenshots)"(w762) -> ()
          }
          frame #5 {
            n435 = flat-sequence {
              tunnel: w786 -> [w789]
              tunnel: [w789] -> w785
              tunnel: w787 -> [w804]
              tunnel: w785 -> [w792]
              tunnel: [w791] -> w784
              tunnel: w783 -> [w790]
              frame #0 {
                n436 = property class="TabCtl (strict)"("Val(Sgnl)"=T1."DMMs" ("Value (Signaling)")) -> ()  [unwired: 2 in, 2 out]
              }
              frame #1 {
                w802 = "_" ("string")
                n437 = local read "Cycle #"() -> (w800:u32)
                n438 = call "LV_UNIXTIME.vi"("current time"=w792) -> ("date/time string"=w803:string)  [unwired: 9 in, 1 out]
                n439 = Format Value(format string="%06d", value (0)=w800) -> (output string=w799:string)  [unwired: 1 in]
                n440 = Concatenate Strings(w790, w803, w802, w799, w802, "page6.png" ("string")) -> (w797:string)
                n441 = invoke class="TabCtl (strict)" method="Get Image"(error in=errorcluster {"status"=FALSE, "code"=0, "source"=""} ("error in (no error)")) -> (error out=w793:errorcluster, "image data"=w795:T24)  [unwired: 5 in, 4 out]
                n442 = Build Path(base path=w804, name or relative path=w797) -> (appended path=w796:path)
                n443 = call <vilib>:"Write PNG File.vi"("error in (no error)"=w793, "image data"=w795, "path to PNG file"=w796) -> ("error out"=w791:errorcluster)  [unwired: 7 in, 1 out]
              }
            }
            n444 = local write "error out (frontpanel screenshots)"(w784) -> ()
          }
          frame #6 {
            n445 = flat-sequence {
              tunnel: w808 -> [w811]
              tunnel: [w811] -> w807
              tunnel: w809 -> [w826]
              tunnel: w807 -> [w814]
              tunnel: [w813] -> w806
              tunnel: w805 -> [w812]
              frame #0 {
                n446 = property class="TabCtl (strict)"("Val(Sgnl)"=T1."DIAGRAM" ("Value (Signaling)")) -> ()  [unwired: 2 in, 2 out]
              }
              frame #1 {
                w824 = "_" ("string")
                n447 = local read "Cycle #"() -> (w822:u32)
                n448 = Format Value(format string="%06d", value (0)=w822) -> (output string=w821:string)  [unwired: 1 in]
                n449 = call "LV_UNIXTIME.vi"("current time"=w814) -> ("date/time string"=w825:string)  [unwired: 9 in, 1 out]
                n450 = Concatenate Strings(w812, w825, w824, w821, w824, "page7.png" ("string")) -> (w819:string)
                n451 = invoke class="TabCtl (strict)" method="Get Image"(error in=errorcluster {"status"=FALSE, "code"=0, "source"=""} ("error in (no error)")) -> (error out=w815:errorcluster, "image data"=w817:T24)  [unwired: 5 in, 4 out]
                n452 = Build Path(base path=w826, name or relative path=w819) -> (appended path=w818:path)
                n453 = call <vilib>:"Write PNG File.vi"("error in (no error)"=w815, "image data"=w817, "path to PNG file"=w818) -> ("error out"=w813:errorcluster)  [unwired: 7 in, 1 out]
              }
            }
            n454 = local write "error out (frontpanel screenshots)"(w806) -> ()
          }
          frame #7 {
            n455 = flat-sequence {
              tunnel: w830 -> [w833]
              tunnel: [w833] -> w829
              tunnel: w831 -> [w848]
              tunnel: w829 -> [w836]
              tunnel: [w835] -> w828
              tunnel: w827 -> [w834]
              frame #0 {
                n456 = property class="TabCtl (strict)"("Val(Sgnl)"=T1."CHF" ("Value (Signaling)")) -> ()  [unwired: 2 in, 2 out]
              }
              frame #1 {
                w846 = "_" ("string")
                n457 = local read "Cycle #"() -> (w844:u32)
                n458 = Format Value(format string="%06d", value (0)=w844) -> (output string=w843:string)  [unwired: 1 in]
                n459 = call "LV_UNIXTIME.vi"("current time"=w836) -> ("date/time string"=w847:string)  [unwired: 9 in, 1 out]
                n460 = Concatenate Strings(w834, w847, w846, w843, w846, "page8.png" ("string")) -> (w841:string)
                n461 = invoke class="TabCtl (strict)" method="Get Image"(error in=errorcluster {"status"=FALSE, "code"=0, "source"=""} ("error in (no error)")) -> (error out=w837:errorcluster, "image data"=w839:T24)  [unwired: 5 in, 4 out]
                n462 = Build Path(base path=w848, name or relative path=w841) -> (appended path=w840:path)
                n463 = call <vilib>:"Write PNG File.vi"("error in (no error)"=w837, "image data"=w839, "path to PNG file"=w840) -> ("error out"=w835:errorcluster)  [unwired: 7 in, 1 out]
              }
            }
            n464 = local write "error out (frontpanel screenshots)"(w828) -> ()
          }
          frame #8 {
            n465 = flat-sequence {
              tunnel: w852 -> [w855]
              tunnel: [w855] -> w851
              tunnel: w853 -> [w870]
              tunnel: w851 -> [w858]
              tunnel: [w857] -> w850
              tunnel: w849 -> [w856]
              frame #0 {
                n466 = property class="TabCtl (strict)"("Val(Sgnl)"=T1."(Plc. hld.)" ("Value (Signaling)")) -> ()  [unwired: 2 in, 2 out]
              }
              frame #1 {
                w868 = "_" ("string")
                n467 = local read "Cycle #"() -> (w866:u32)
                n468 = Format Value(format string="%06d", value (0)=w866) -> (output string=w865:string)  [unwired: 1 in]
                n469 = call "LV_UNIXTIME.vi"("current time"=w858) -> ("date/time string"=w869:string)  [unwired: 9 in, 1 out]
                n470 = Concatenate Strings(w856, w869, w868, w865, w868, "page8.png" ("string")) -> (w863:string)
                n471 = invoke class="TabCtl (strict)" method="Get Image"(error in=errorcluster {"status"=FALSE, "code"=0, "source"=""} ("error in (no error)")) -> (error out=w859:errorcluster, "image data"=w861:T24)  [unwired: 5 in, 4 out]
                n472 = Build Path(base path=w870, name or relative path=w863) -> (appended path=w862:path)
                n473 = call <vilib>:"Write PNG File.vi"("error in (no error)"=w859, "image data"=w861, "path to PNG file"=w862) -> ("error out"=w857:errorcluster)  [unwired: 7 in, 1 out]
              }
            }
            n474 = local write "error out (frontpanel screenshots)"(w850) -> ()
          }
          frame #9 {
            n475 = local write "Frontpanel screenshots"(FALSE ("Frontpanel screenshots")) -> ()
          }
        }
        "error out (frontpanel screenshots)" <- w669
        n476 = property class="TabCtl (strict)"("Val(Sgnl)"=w667) -> ()  [unwired: 2 in, 2 out]
      }
      event "Stop Button": Value Change {
        n477 = event-data() -> ()  [unwired: 1 in, 3 out]
      }
    }
    n478 = Wait (ms)(milliseconds to wait=u32 123) -> ()  [unwired: 1 out]
  }
  n479 = while {
    stop <- w877 stop-if-true
    n480 = event shown="[5] \"Plot selecter LSI218(1)     1      2     3     4\", \"Plot selecter LSI218(2)     1      2     3     4\", \"Plot selecter (USB6210)     1      2     3     4\", \"Plot selecter LSI336       1      2     3     4\", \"Plot selecter (USB6218)     1      2     3     4\", \"Plot selecter (HP34401A)     1      2     3     4\": Value Change" {
      selector: _ -> [_ _ _ _ _ _ _ _ _ _ _]
      dyn-events: _ -> [_ _ _ _ _ _ _ _ _ _ _]
      timeout: _ -> [_ _ _ _ _ _ _ _ _ _ _]
      tunnel: [_ _ _ _ _ _ _ _ _ _ TRUE] -> w877
      tunnel: [errorcluster {"status"=FALSE, "code"=0, "source"=""} ("error out") w881 _ _ _ _ w1017 w1034 w1051 w1068 errorcluster {"status"=FALSE, "code"=0, "source"=""} ("error out")] -> w873
      event Timeout {
        n481 = event-data() -> ()  [unwired: 1 in, 3 out]
      }
      event "log/linear 1": Value Change {
        n482 = event-data() -> ()  [unwired: 1 in, 6 out]
        n483 = flat-sequence {
          tunnel: [w882] -> w881
          frame #0 {
            n484 = Boolean To (0,1)(Boolean="log/linear 1") -> (0, 1=w887:i16)
            n485 = control-ref of="Graph 1"() -> (w883:refnum<vi>)
            n486 = property class="XYGraph (strict)"(reference=w883, error in=errorcluster {"status"=FALSE, "code"=0, "source"=""} ("error in (no error)"), "YScale.Mapping Mode"=w887) -> (error out=w885:errorcluster)  [unwired: 1 out]
            n487 = control-ref of="error out (USB6210)"() -> (w886:refnum<vi>)
            n488 = property class="Clust (strict)"(reference=w886, "Val(Sgnl)"=w885) -> (error out=w882:errorcluster)  [unwired: 1 in, 1 out]
          }
        }
      }
      event "log/linear 2": Value Change {
        n489 = event-data() -> ()  [unwired: 1 in, 6 out]
        n490 = flat-sequence {
          frame #0 {
            n491 = Boolean To (0,1)(Boolean="log/linear 2") -> (0, 1=w893:i16)
            n492 = control-ref of="Graph 2"() -> (w891:refnum<vi>)
            n493 = property class="XYGraph (strict)"(reference=w891, error in=errorcluster {"status"=FALSE, "code"=0, "source"=""} ("error in (no error)"), "YScale.Mapping Mode"=w893) -> (error out=w892:errorcluster)  [unwired: 1 out]
            n494 = control-ref of="error out (USB6210)"() -> (w890:refnum<vi>)
            n495 = property class="Clust (strict)"(reference=w890, "Value"=w892) -> ()  [unwired: 1 in, 2 out]
          }
        }
      }
      event "log/linear 3": Value Change {
        n496 = event-data() -> ()  [unwired: 1 in, 6 out]
        n497 = flat-sequence {
          frame #0 {
            n498 = Boolean To (0,1)(Boolean="log/linear 3") -> (0, 1=w899:i16)
            n499 = control-ref of="Graph 3"() -> (w895:refnum<vi>)
            n500 = property class="XYGraph (strict)"(reference=w895, error in=errorcluster {"status"=FALSE, "code"=0, "source"=""} ("error in (no error)"), "YScale.Mapping Mode"=w899) -> (error out=w898:errorcluster)  [unwired: 1 out]
            n501 = control-ref of="error out (USB6210)"() -> (w897:refnum<vi>)
            n502 = property class="Clust (strict)"(reference=w897, "Value"=w898) -> ()  [unwired: 1 in, 2 out]
          }
        }
      }
      event "log/linear 4": Value Change {
        n503 = event-data() -> ()  [unwired: 1 in, 6 out]
        n504 = flat-sequence {
          frame #0 {
            n505 = Boolean To (0,1)(Boolean="log/linear 4") -> (0, 1=w905:i16)
            n506 = control-ref of="Graph 4"() -> (w901:refnum<vi>)
            n507 = property class="XYGraph (strict)"(reference=w901, error in=errorcluster {"status"=FALSE, "code"=0, "source"=""} ("error in (no error)"), "YScale.Mapping Mode"=w905) -> (error out=w904:errorcluster)  [unwired: 1 out]
            n508 = control-ref of="error out (USB6210)"() -> (w903:refnum<vi>)
            n509 = property class="Clust (strict)"(reference=w903, "Value"=w904) -> ()  [unwired: 1 in, 2 out]
          }
        }
      }
      event "Plot selecter LSI218(1)\n    1      2     3     4", "Plot selecter LSI218(2)\n    1      2     3     4", "Plot selecter (USB6210)\n    1      2     3     4", "Plot selecter LSI336 \n     1      2     3     4", "Plot selecter (USB6218)\n    1      2     3     4", "Plot selecter (HP34401A)\n    1      2     3     4": Value Change {
        n510 = event-data() -> ()  [unwired: 1 in, 6 out]
        n511 = local read "Labels (HP34401 LM)"() -> (w912:string[])
        n512 = call "BuildPlotLegends.vi"("Plot selecter \n    1      2     3     4"="Plot selecter (HP34401A)\n    1      2     3     4", "AllLabels"=w912) -> ("Series 4"=w907:string[], "Series 3"=w908:string[], "Series 2"=w909:string[], "Series 1"=w910:string[])  [unwired: 6 in]
        n513 = local read "All Labels (USB6210)"() -> (w929:string[])
        n514 = local read "All Labels (USB6218)"() -> (w918:string[])
        n515 = local read "Labels LSI218 (1)"() -> (w931:string[])
        n516 = local read "Labels LSI218 (2)"() -> (w932:string[])
        n517 = local read "Labels LSI336"() -> (w924:string[])
        n518 = call "BuildPlotLegends_LSI218.vi"("Plot selecter (2)\n    1      2     3     5"="Plot selecter LSI218(2)\n    1      2     3     4", "Plot selecter (1)\n    1      2     3     4"="Plot selecter LSI218(1)\n    1      2     3     4", "Labels (2)"=w932, "Labels (1)"=w931) -> ("Series 4"=w942:string[], "Series 3"=w940:string[], "Series 2"=w938:string[], "Series 1"=w936:string[])  [unwired: 4 in]
        n519 = call "BuildPlotLegends.vi"("Plot selecter \n    1      2     3     4"="Plot selecter (USB6210)\n    1      2     3     4", "AllLabels"=w929) -> ("Series 4"=w941:string[], "Series 3"=w939:string[], "Series 2"=w937:string[], "Series 1"=w935:string[])  [unwired: 6 in]
        n520 = call "BuildPlotLegends.vi"("Plot selecter \n    1      2     3     4"="Plot selecter LSI336 \n     1      2     3     4", "AllLabels"=w924) -> ("Series 4"=w919:string[], "Series 3"=w920:string[], "Series 2"=w921:string[], "Series 1"=w922:string[])  [unwired: 6 in]
        n521 = call "BuildPlotLegends.vi"("Plot selecter \n    1      2     3     4"="Plot selecter (USB6218)\n    1      2     3     4", "AllLabels"=w918) -> ("Series 4"=w914:string[], "Series 3"=w913:string[], "Series 2"=w915:string[], "Series 1"=w916:string[])  [unwired: 6 in]
        n522 = Build Array (concatenate)(w937, w938, w921, w915, w909) -> (w926:string[])
        "Series 2" <- w926
        n523 = Build Array (concatenate)(w939, w940, w920, w913, w908) -> (w927:string[])
        "Series 3" <- w927
        n524 = Build Array (concatenate)(w941, w942, w919, w914, w907) -> (w928:string[])
        "Series 4" <- w928
        n525 = Build Array (concatenate)(w935, w936, w922, w916, w910) -> (w925:string[])
        "Series 1" <- w925
        n526 = stacked-sequence {
          tunnel: [w952 _ _ _] -> w946
          tunnel: [_ w970 _ _] -> w947
          tunnel: [_ _ w987 _] -> w945
          tunnel: [_ _ _ w1004] -> w944
          tunnel: w925 -> [w950 _ _ _]
          tunnel: w926 -> [_ w968 _ _]
          tunnel: w927 -> [_ _ w985 _]
          tunnel: w928 -> [_ _ _ w1002]
          frame #0 {
            n527 = Array Size(array=w950) -> (size(s)=w954:i32)
            n528 = control-ref of="Graph 1"() -> (w948:refnum<vi>)
            n529 = property class="XYGraph (strict)"(reference=w948) -> ("LegNumRows"=w949:u32)  [unwired: 1 in, 2 out]
            n530 = for {
              N: w949 -> [_]
              tunnel: w948 -> [w963]
              shift-right: [w961] -> w953
              shift-left: errorcluster {"status"=FALSE, "code"=0, "source"=""} ("error in (no error)") -> [w962]
              i -> [w965]
              n531 = property class="XYGraph (strict)"(reference=w963, error in=w962, "Active Plot"=w965, "Plot.Plot Name"="") -> (error out=w961:errorcluster)  [unwired: 1 out]
            }
            n532 = for {
              N: w954 -> [_]
              tunnel: w948 -> [w959]
              shift-right: [w957] -> w952
              shift-left: w953 -> [w958]
              tunnel: w950 -> [w956] mode=indexing
              i -> [w960]
              n533 = property class="XYGraph (strict)"(reference=w959, error in=w958, "Active Plot"=w960, "Plot.Plot Name"=w956, "Plot.Visible?"=TRUE ("Plot.Visible")) -> (error out=w957:errorcluster)  [unwired: 1 out]
            }
          }
          frame #1 {
            n534 = Array Size(array=w968) -> (size(s)=w972:i32)
            n535 = control-ref of="Graph 2"() -> (w967:refnum<vi>)
            n536 = property class="XYGraph (strict)"(reference=w967) -> ("LegNumRows"=w966:u32)  [unwired: 1 in, 2 out]
            n537 = for {
              N: w966 -> [_]
              shift-right: [w979] -> w971
              shift-left: errorcluster {"status"=FALSE, "code"=0, "source"=""} ("error in (no error)") -> [w980]
              tunnel: w967 -> [w978]
              i -> [w982]
              n538 = property class="XYGraph (strict)"(reference=w978, error in=w980, "Active Plot"=w982, "Plot.Plot Name"="") -> (error out=w979:errorcluster)  [unwired: 1 out]
            }
            n539 = for {
              N: w972 -> [_]
              shift-right: [w975] -> w970
              shift-left: w971 -> [w976]
              tunnel: w968 -> [w974] mode=indexing
              tunnel: w967 -> [w973]
              i -> [w977]
              n540 = property class="XYGraph (strict)"(reference=w973, error in=w976, "Active Plot"=w977, "Plot.Plot Name"=w974) -> (error out=w975:errorcluster)  [unwired: 1 out]
            }
          }
          frame #2 {
            n541 = Array Size(array=w985) -> (size(s)=w989:i32)
            n542 = control-ref of="Graph 3"() -> (w983:refnum<vi>)
            n543 = property class="XYGraph (strict)"(reference=w983) -> ("LegNumRows"=w984:u32)  [unwired: 1 in, 2 out]
            n544 = for {
              N: w984 -> [_]
              tunnel: w983 -> [w997]
              shift-right: [w995] -> w988
              shift-left: errorcluster {"status"=FALSE, "code"=0, "source"=""} ("error in (no error)") -> [w996]
              i -> [w999]
              n545 = property class="XYGraph (strict)"(reference=w997, error in=w996, "Active Plot"=w999, "Plot.Plot Name"="") -> (error out=w995:errorcluster)  [unwired: 1 out]
            }
            n546 = for {
              N: w989 -> [_]
              tunnel: w983 -> [w993]
              shift-right: [w991] -> w987
              shift-left: w988 -> [w992]
              tunnel: w985 -> [w990] mode=indexing
              i -> [w994]
              n547 = property class="XYGraph (strict)"(reference=w993, error in=w992, "Active Plot"=w994, "Plot.Plot Name"=w990) -> (error out=w991:errorcluster)  [unwired: 1 out]
            }
          }
          frame #3 {
            n548 = Array Size(array=w1002) -> (size(s)=w1006:i32)
            n549 = control-ref of="Graph 4"() -> (w1000:refnum<vi>)
            n550 = property class="XYGraph (strict)"(reference=w1000) -> ("LegNumRows"=w1001:u32)  [unwired: 1 in, 2 out]
            n551 = for {
              N: w1001 -> [_]
              tunnel: w1000 -> [w1014]
              shift-right: [w1012] -> w1005
              shift-left: errorcluster {"status"=FALSE, "code"=0, "source"=""} ("error in (no error)") -> [w1013]
              i -> [w1016]
              n552 = property class="XYGraph (strict)"(reference=w1014, error in=w1013, "Active Plot"=w1016, "Plot.Plot Name"="") -> (error out=w1012:errorcluster)  [unwired: 1 out]
            }
            n553 = for {
              N: w1006 -> [_]
              tunnel: w1000 -> [w1010]
              shift-right: [w1008] -> w1004
              shift-left: w1005 -> [w1009]
              tunnel: w1002 -> [w1007] mode=indexing
              i -> [w1011]
              n554 = property class="XYGraph (strict)"(reference=w1010, error in=w1009, "Active Plot"=w1011, "Plot.Plot Name"=w1007) -> (error out=w1008:errorcluster)  [unwired: 1 out]
            }
          }
        }
        n555 = Merge Errors(w946, w947, w945, w944) -> (→"Plot errors":errorcluster)
      }
      event "Take Screenshot! 1": Value Change {
        n556 = event-data() -> ()  [unwired: 1 in, 6 out]
        n557 = flat-sequence {
          tunnel: [w1018] -> w1017
          frame #0 {
            n558 = flat-sequence {
              tunnel: [w1019] -> w1018
              frame #0 {
                w1028 = "_" ("string")
                n559 = Get Date/Time In Seconds() -> (seconds since 1Jan1904=w1025:timestamp)
                n560 = local read "RUN Identifier"() -> (w1030:string)
                n561 = call "LV_UNIXTIME.vi"("current time"=w1025) -> ("date/time string"=w1029:string)  [unwired: 9 in, 1 out]
                n562 = control-ref of="Graph 1"() -> (w1024:refnum<vi>)
                n563 = Concatenate Strings(w1030, w1028, w1029, w1028, "FIle suffix 1", ".png" ("string")) -> (w1032:string)
                n564 = local read "Base Path"() -> (w1031:path)
                n565 = invoke class="XYGraph (strict)" method="Get Image"(reference=w1024, error in=errorcluster {"status"=FALSE, "code"=0, "source"=""} ("error in (no error)")) -> (error out=w1020:errorcluster, "image data"=w1023:T24)  [unwired: 4 in, 4 out]
                n566 = Build Path(base path=w1031, name or relative path=w1032) -> (appended path=w1022:path)
                n567 = call <vilib>:"Write PNG File.vi"("error in (no error)"=w1020, "image data"=w1023, "path to PNG file"=w1022) -> ("error out"=w1019:errorcluster)  [unwired: 7 in, 1 out]
              }
              frame #1 {
                n568 = local write "Take Screenshot! 1"(FALSE ("Take Screenshot! 1")) -> ()
              }
            }
          }
        }
      }
      event "Take Screenshot! 2": Value Change {
        n569 = event-data() -> ()  [unwired: 1 in, 6 out]
        n570 = flat-sequence {
          tunnel: [w1035] -> w1034
          frame #0 {
            n571 = flat-sequence {
              tunnel: [w1041] -> w1035
              frame #0 {
                w1045 = "_" ("string")
                n572 = Get Date/Time In Seconds() -> (seconds since 1Jan1904=w1042:timestamp)
                n573 = local read "RUN Identifier"() -> (w1047:string)
                n574 = call "LV_UNIXTIME.vi"("current time"=w1042) -> ("date/time string"=w1046:string)  [unwired: 9 in, 1 out]
                n575 = control-ref of="Graph 2"() -> (w1036:refnum<vi>)
                n576 = Concatenate Strings(w1047, w1045, w1046, w1045, "FIle suffix 2", ".png" ("string")) -> (w1049:string)
                n577 = local read "Base Path"() -> (w1048:path)
                n578 = invoke class="XYGraph (strict)" method="Get Image"(reference=w1036, error in=errorcluster {"status"=FALSE, "code"=0, "source"=""} ("error in (no error)")) -> (error out=w1040:errorcluster, "image data"=w1038:T24)  [unwired: 4 in, 4 out]
                n579 = Build Path(base path=w1048, name or relative path=w1049) -> (appended path=w1037:path)
                n580 = call <vilib>:"Write PNG File.vi"("error in (no error)"=w1040, "image data"=w1038, "path to PNG file"=w1037) -> ("error out"=w1041:errorcluster)  [unwired: 7 in, 1 out]
              }
              frame #1 {
                n581 = local write "Take Screenshot! 2"(FALSE ("Take Screenshot! 1")) -> ()
              }
            }
          }
        }
      }
      event "Take Screenshot! 3": Value Change {
        n582 = event-data() -> ()  [unwired: 1 in, 6 out]
        n583 = flat-sequence {
          tunnel: [w1052] -> w1051
          frame #0 {
            n584 = flat-sequence {
              tunnel: [w1054] -> w1052
              frame #0 {
                w1062 = "_" ("string")
                n585 = Get Date/Time In Seconds() -> (seconds since 1Jan1904=w1060:timestamp)
                n586 = local read "RUN Identifier"() -> (w1064:string)
                n587 = call "LV_UNIXTIME.vi"("current time"=w1060) -> ("date/time string"=w1063:string)  [unwired: 9 in, 1 out]
                n588 = control-ref of="Graph 3"() -> (w1057:refnum<vi>)
                n589 = Concatenate Strings(w1064, w1062, w1063, w1062, "FIle suffix 3", ".png" ("string")) -> (w1066:string)
                n590 = local read "Base Path"() -> (w1065:path)
                n591 = invoke class="XYGraph (strict)" method="Get Image"(reference=w1057, error in=errorcluster {"status"=FALSE, "code"=0, "source"=""} ("error in (no error)")) -> (error out=w1055:errorcluster, "image data"=w1053:T24)  [unwired: 4 in, 4 out]
                n592 = Build Path(base path=w1065, name or relative path=w1066) -> (appended path=w1058:path)
                n593 = call <vilib>:"Write PNG File.vi"("error in (no error)"=w1055, "image data"=w1053, "path to PNG file"=w1058) -> ("error out"=w1054:errorcluster)  [unwired: 7 in, 1 out]
              }
              frame #1 {
                n594 = local write "Take Screenshot! 3"(FALSE ("Take Screenshot! 1")) -> ()
              }
            }
          }
        }
      }
      event "Take Screenshot! 4": Value Change {
        n595 = event-data() -> ()  [unwired: 1 in, 6 out]
        n596 = flat-sequence {
          tunnel: [w1069] -> w1068
          frame #0 {
            n597 = flat-sequence {
              tunnel: [w1072] -> w1069
              frame #0 {
                w1079 = "_" ("string")
                n598 = Get Date/Time In Seconds() -> (seconds since 1Jan1904=w1077:timestamp)
                n599 = local read "RUN Identifier"() -> (w1081:string)
                n600 = call "LV_UNIXTIME.vi"("current time"=w1077) -> ("date/time string"=w1080:string)  [unwired: 9 in, 1 out]
                n601 = control-ref of="Graph 4"() -> (w1073:refnum<vi>)
                n602 = Concatenate Strings(w1081, w1079, w1080, w1079, "FIle suffix 4", ".png" ("string")) -> (w1083:string)
                n603 = local read "Base Path"() -> (w1082:path)
                n604 = invoke class="XYGraph (strict)" method="Get Image"(reference=w1073, error in=errorcluster {"status"=FALSE, "code"=0, "source"=""} ("error in (no error)")) -> (error out=w1070:errorcluster, "image data"=w1074:T24)  [unwired: 4 in, 4 out]
                n605 = Build Path(base path=w1082, name or relative path=w1083) -> (appended path=w1075:path)
                n606 = call <vilib>:"Write PNG File.vi"("error in (no error)"=w1070, "image data"=w1074, "path to PNG file"=w1075) -> ("error out"=w1072:errorcluster)  [unwired: 7 in, 1 out]
              }
              frame #1 {
                n607 = local write "Take Screenshot! 4"(FALSE ("Take Screenshot! 1")) -> ()
              }
            }
          }
        }
      }
      event "Stop Button": Value Change {
        n608 = event-data() -> ()  [unwired: 1 in, 6 out]
      }
    }
    "error out (graph operations)" <- w873
    n609 = local write "Take Screenshot! 1"(FALSE ("Take Screenshot! 1")) -> ()
    n610 = local write "Take Screenshot! 2"(FALSE ("Take Screenshot! 1")) -> ()
    n611 = Wait (ms)(milliseconds to wait=u32 1000) -> ()  [unwired: 1 out]
    n612 = local write "Take Screenshot! 3"(FALSE ("Take Screenshot! 1")) -> ()
    n613 = local write "Take Screenshot! 4"(FALSE ("Take Screenshot! 1")) -> ()
  }
  n614 = while {
    i -> [w1091]
    stop <- w1088 stop-if-true
    n615 = Equal?(x=w1091, y=0) -> (x = y?=w1089:bool)
    n616 = case shown="True" w1089 {
      frame False {
      }
      frame True {
        n617 = property on="Agilent\nIntialized?" class="Bool (strict)"("Val(Sgnl)"=FALSE ("Value (Signaling)")) -> ()  [unwired: 2 in, 2 out]
      }
    }
    n618 = Wait (ms)(milliseconds to wait=u32 123) -> ()  [unwired: 1 out]
    n619 = event shown="[3] \"OUTPUT  Kenwood\", \"Kenwood set V (V)\": Value Change" {
      selector: _ -> [_ _ _ _ _]
      dyn-events: _ -> [_ _ _ _ _]
      timeout: _ -> [_ _ _ _ _]
      tunnel: [FALSE ("Value (Signaling)") TRUE ("Value (Signaling)") _ _ _] -> w1088
      tunnel: "VISA (Agilent 34402)" -> [_ _ w1097 w1100 _]
      event Timeout {
        n620 = event-data() -> ()  [unwired: 1 in, 3 out]
      }
      event "Stop Button": Value Change {
        n621 = event-data() -> ()  [unwired: 1 in, 3 out]
      }
      event "Initialize (Agilent)": Value Change {
        n622 = event-data() -> ()  [unwired: 1 in, 3 out]
        n623 = property on="Agilent\nIntialized?" class="Bool (strict)"("Val(Sgnl)"=TRUE ("Value (Signaling)")) -> ()  [unwired: 2 in, 2 out]
        n624 = call "Initialize.vi"("error in (no error)"=errorcluster {"status"=FALSE, "code"=0, "source"=""}, "VISA resource name"=w1097) -> ("error out"=→"error out (Agilent)":errorcluster)  [unwired: 8 in, 1 out]
      }
      event "OUTPUT \nKenwood", "Kenwood set V (V)": Value Change {
        n625 = local read "Agilent\nIntialized?"() -> (w1099:bool)
        n626 = event-data() -> ()  [unwired: 1 in, 3 out]
        n627 = case shown="True" w1099 {
          tunnel: w1100 -> [_ w1106]
          frame False {
          }
          frame True {
            w1108 = u16 0 items=["DC", "Sine", "Square", "Triangle", "Ramp", "Pulse", "Noise", "Sinc", "Negative Ramp", "Exponential Rise", "Exponential Fall", "Cardiac"] ("Waveform Function (1: Sine)")
            n628 = xnode "Formula"("X1"="Kenwood set V (V)") -> ("Result"=w1101:dbl)  [unwired: 1 in, 1 out]
            n629 = call "Configure Standard Waveform.vi"("DC Offset (0.00 V)"=w1101, "Frequency (1000 Hz)"=1.0, "error in (no error)"=errorcluster {"status"=FALSE, "code"=0, "source"=""}, "Amplitude (1)"=1.0, "Waveform Function (1: Sine)"=w1108, "VISA resource name"=w1106) -> ("error out"=w1110:errorcluster, "VISA resource name out"=w1111:refnum<visa-resource-name>)  [unwired: 4 in]
            n630 = call "Enable Output.vi"("error in (no error)"=w1110, "Enable Output  (T: Enable)"="OUTPUT \nKenwood", "VISA resource name"=w1111) -> ("error out"=w1104:errorcluster)  [unwired: 7 in, 1 out]
            n631 = local write "error out (Agilent)"(w1104) -> ()
          }
        }
      }
      event "V_lim_up (V)", "V_lim_low (V)": Value Change {
        n632 = event-data() -> ()  [unwired: 1 in, 3 out]
        n633 = property on="Kenwood set V (V)" class="DigNum (strict)"("Minimum"="V_lim_low (V)", "Maximum"="V_lim_up (V)") -> ()  [unwired: 2 in, 2 out]
      }
    }
  }
  n634 = while {
    stop <- w1123 stop-if-true
    n635 = Wait (ms)(milliseconds to wait=u32 101) -> ()  [unwired: 1 out]
    n636 = event shown="[2] Timeout" {
      selector: _ -> [_ _ _]
      dyn-events: _ -> [_ _ _]
      timeout: _ -> [_ _ _]
      tunnel: [FALSE TRUE FALSE] -> w1123
      event "Initialize (DMMs)": Value Change {
        w1126 = T4 [] ("Value (Signaling)")
        n637 = event-data() -> ()  [unwired: 1 in, 3 out]
        n638 = property on="Graph DMMs 1" class="XYGraph (strict)"("Val(Sgnl)"=w1126) -> ()  [unwired: 2 in, 2 out]
        n639 = property on="Graph DMMs 2" class="XYGraph (strict)"("Val(Sgnl)"=w1126) -> ()  [unwired: 2 in, 2 out]
      }
      event "Stop Button": Value Change {
        n640 = event-data() -> ()  [unwired: 1 in, 3 out]
      }
      event Timeout {
        n641 = event-data() -> ()  [unwired: 1 in, 3 out]
      }
    }
  }
  n642 = Obtain Notifier(name (unnamed)="stop notifier", notification data type=w17, create if not found? (T)=w17, error in (no error)=errorcluster {"status"=FALSE, "code"=0, "source"=""}) -> (notifier out=w5:refnum<notifier>, error out=w4:errorcluster)  [unwired: 1 out]
  n643 = while {
    shift-right: [w1239] -> w40
    shift-left: refnum<class "USBData.lvclass"> refnum ("USBData.lvclass") -> [w1242]
    shift-right: [w1235] -> w39
    shift-left: w6 -> [w1241]
    tunnel: "Base Path" -> [w1141]
    shift-right: [w1217] -> w34
    shift-left: errorcluster {"status"=FALSE, "code"=0, "source"=""} ("error in (no error)") -> [w1233]
    shift-right: [w1218] -> w35
    shift-left: refnum<class "LSI218Data.lvclass"> refnum ("LSI218Data.lvclass") -> [w1232]
    shift-right: [w1205] -> w31
    shift-left: refnum<class "LSI336Data.lvclass"> refnum ("LSI336Data.lvclass") -> [w1214]
    shift-right: [w1204] -> w30
    shift-left: w21 -> [w1213]
    shift-right: [w1193] -> _
    shift-left: w6 -> [w1194]
    shift-right: [w1183] -> w25
    shift-left: refnum<class "USBData.lvclass"> refnum ("USBData.lvclass") -> [w1191]
    shift-right: [w1182] -> w24
    shift-left: errorcluster {"status"=FALSE, "code"=0, "source"=""} ("error in (no error)") -> [w1190]
    shift-right: [w1179] -> _
    shift-left: w21 -> [w1178]
    tunnel: w5 -> [w1149]
    tunnel: w4 -> [w1148]
    tunnel: [w1146] -> w13
    tunnel: [w1145] -> w12
    shift-right: [w1142] -> _
    shift-left: refnum<class "LMData.lvclass"> refnum ("LMData in") -> [w1143]
    shift-right: [w1139] -> _
    shift-left: errorcluster {"status"=FALSE, "code"=0, "source"=""} ("error in (no error)") -> [w1140]
    i -> [w1138]
    stop <- "Stop Button" stop-if-true
    w1134 = T26 [] ("appended array")
    w1200 = u32 24 ("Number of Rows")
    w1210 = T26 [] ("appended array")
    w1227 = T26 [] ("appended array")
    n644 = local read "LSI218Settings(A-F)"() -> (w1170:T3)
    n645 = control-ref of="Plot selecter LSI218(2)\n    1      2     3     4"() -> (w1198:refnum<vi>)
    n646 = control-ref of="Plot selecter LSI218(1)\n    1      2     3     4"() -> (w1199:refnum<vi>)
    n647 = control-ref of="Plot selecter LSI336 \n     1      2     3     4"() -> (w1197:refnum<vi>)
    n648 = property on="Property Node" class="Arr (strict)"(reference=w1198, "Number of Rows"=w1200) -> ()  [unwired: 1 in, 2 out]
    n649 = property on="Property Node" class="Arr (strict)"(reference=w1199, "Number of Rows"=w1200) -> ()  [unwired: 1 in, 2 out]
    n650 = local read "LSI336Settings(X,Y)"() -> (w1168:T3)
    n651 = Array Size(array=w1170) -> (size(s)=w1169:i32)
    n652 = property on="Property Node" class="Arr (strict)"(reference=w1197, "Number of Rows"=u32 8) -> ()  [unwired: 1 in, 2 out]
    n653 = Multiply(x="Measurement Interval (s)", y=u32 1000) -> (x*y=w1236:dbl)
    n654 = Wait (ms)(milliseconds to wait=w1236) -> ()  [unwired: 1 out]
    n655 = for {
      N: w1169 -> [_]
      tunnel: w1170 -> [w1330] mode=indexing
      tunnel: [w1329] -> w1166 mode=concatenating
      n656 = Unbundle By Name(w1330) -> ("SensorLocations"=w1329:T19)
    }
    n657 = for {
      tunnel: w1168 -> [w1328] mode=indexing
      tunnel: [w1327] -> w1167 mode=concatenating
      n658 = Unbundle By Name(w1328) -> ("SensorLocations"=w1327:T19)
    }
    n659 = Quotient & Remainder(x=w1138, y="Screenshots interval") -> (x-y*floor(x/y)=w1154:i64)  [unwired: 1 out]
    n660 = Equal?(x=w1138, y=0) -> (x = y?=w1144:bool)
    n661 = case shown="True" w1144 {
      tunnel: w1242 -> [w2393 w2416]
      tunnel: w1241 -> [w2387 w2414]
      tunnel: w1138 -> [w2378 _]
      tunnel: [w2385 w2411] -> w1235
      tunnel: [w2382 w2410] -> w1192
      tunnel: [w2383 w2409] -> w1239
      tunnel: [w2373 w2404] -> w1240
      tunnel: w1141 -> [_ w2403]
      tunnel: [w2372 w2400] -> w1175
      frame False {
        n662 = call-dynamic "USBData_measure.vi"("USBData in"=w2393, "DAQ sample #"=i64 5, "DAQ timeout"=100.0 ("DAQ timeout (def: 100)"), "MeasurementIndex"=w2378, "error in (no error)"=w2387, "save every ... measurements"="Record interval") -> ("USBData out"=w2392:refnum<class "USBData.lvclass">, "TimeMeasuremeent"=w2389:timestamp, "Status"=→"USB6210 Status":T6, "LastDataAcquired"=w2374:dbl[], "error out"=w2388:errorcluster)  [unwired: 3 in, 2 out]
        "Time of Last Measurement (USB6210)" <- w2389
        "Last Vol\n(USB6210)" <- w2374
        n663 = call-dynamic "USBData_convert.vi"("Save every ... measurements"="Record interval", "MeasurementIndex"=w2378, "error in (no error)"=w2388, "LastDataAcquired"=w2374, "TimeMeasuremeent"=w2389, "USBData in"=w2392) -> ("error out"=w2386:errorcluster, "LeakDet_FULL"=w2381:dbl, "LastDataConverted"=w2375:dbl[], "USBData out"=w2384:refnum<class "USBData.lvclass">)  [unwired: 2 in]
        n664 = call "USBData_read.vi"("USBData in"=w2384, "error in (no error)"=w2386) -> ("Status"=w2376:T6, "USBData out"=w2383:refnum<class "USBData.lvclass">, "Data"=w2382:T27, "Basic"=w2373:T28, "error out"=w2385:errorcluster)  [unwired: 2 in, 2 out]
        n665 = local write "USB6210 Status"(w2376) -> ()
        n666 = Unbundle By Name(w2373) -> ("ReadLeakDet?"=w2380:bool)
        n667 = Unbundle By Name(w2373) -> ("Labels"=w2372:string[])
        n668 = case shown="False" w2380 {
          tunnel: w2375 -> [w2394 w2397]
          tunnel: w2381 -> [_ w2396]
          tunnel: [w2394 w2395] -> w2379
          frame False {
          }
          frame True {
            n669 = Build Array (concatenate)(w2397, w2396) -> (w2395:dbl[])
          }
        }
        "Last Data \n(USB6210)" <- w2379
      }
      frame True {
        n670 = local read "RUN Identifier"() -> (w2398:string)
        n671 = call-dynamic "USBData_initialize.vi"("USBData in"=w2416, "SeriesSetting"="USB6210 Config", "BasePath"=w2403, "RunIdentifier"=w2398, "FileName"="InstName (USB6210)", "error in (no error)"=w2414) -> ("Status"=w2399:T6, "USBData out"=w2412:refnum<class "USBData.lvclass">, "error out"=w2413:errorcluster)  [unwired: 5 in, 2 out]
        n672 = local write "USB6210 Status"(w2399) -> ()
        n673 = call "USBData_read.vi"("USBData in"=w2412, "error in (no error)"=w2413) -> ("Status"=w2402:T6, "USBData out"=w2409:refnum<class "USBData.lvclass">, "Data"=w2410:T27, "Basic"=w2404:T28, "error out"=w2411:errorcluster)  [unwired: 2 in, 2 out]
        n674 = local write "USB6210 Status"(w2402) -> ()
        n675 = Unbundle By Name(w2404) -> ("ReadLeakDet?"=w2408:bool, "Labels"=w2400:string[])
        n676 = Array Size(array=w2400) -> (size(s)=w2407:i32)
        n677 = case shown="True" w2408 {
          tunnel: w2407 -> [w2417 w2419]
          tunnel: [w2417 w2418] -> w2405
          frame False {
          }
          frame True {
            n678 = Add(x=w2419, y=1) -> (x+y=w2418:i32)
          }
        }
        n679 = Initialize Array(TRUE ("Activate 2"), w2405) -> ()  [unwired: 1 out]
      }
    }
    "error out (USB6210)" <- w1235
    n680 = case shown="False" w1144 {
      tunnel: [w1911 w1938] -> w1182
      tunnel: [w1908 w1937] -> w1189
      tunnel: [w1909 w1936] -> w1183
      tunnel: [w1900 w1931] -> w1188
      tunnel: [w1899 w1929] -> _
      tunnel: w1191 -> [w1898 w1927]
      tunnel: w1141 -> [_ w1926]
      tunnel: w1190 -> [w1897 w1925]
      tunnel: w1138 -> [w1896 _]
      frame False {
        n681 = local read "Record interval"() -> (w1895:i64)
        n682 = call-dynamic "USBData_measure.vi"("USBData in"=w1898, "DAQ sample #"=i64 5, "DAQ timeout"=100.0 ("DAQ timeout (def: 100)"), "MeasurementIndex"=w1896, "error in (no error)"=w1897, "save every ... measurements"=w1895) -> ("USBData out"=w1917:refnum<class "USBData.lvclass">, "TimeMeasuremeent"=w1914:timestamp, "Status"=→"USB6218 Status":T6, "LastDataAcquired"=w1901:dbl[], "error out"=w1913:errorcluster)  [unwired: 3 in, 2 out]
        "Time of Last Measurement (USB6218)" <- w1914
        "Last Vol \n(USB6218)" <- w1901
        n683 = call-dynamic "USBData_convert.vi"("Save every ... measurements"=w1895, "MeasurementIndex"=w1896, "error in (no error)"=w1913, "LastDataAcquired"=w1901, "TimeMeasuremeent"=w1914, "USBData in"=w1917) -> ("error out"=w1912:errorcluster, "LeakDet_FULL"=w1907:dbl, "LastDataConverted"=w1902:dbl[], "USBData out"=w1910:refnum<class "USBData.lvclass">)  [unwired: 2 in]
        n684 = call "USBData_read.vi"("USBData in"=w1910, "error in (no error)"=w1912) -> ("Status"=w1903:T6, "USBData out"=w1909:refnum<class "USBData.lvclass">, "Data"=w1908:T27, "Basic"=w1900:T28, "error out"=w1911:errorcluster)  [unwired: 2 in, 2 out]
        n685 = local write "USB6218 Status"(w1903) -> ()
        n686 = Unbundle By Name(w1900) -> ("ReadLeakDet?"=w1906:bool)
        n687 = Unbundle By Name(w1900) -> ("Labels"=w1899:string[])
        n688 = case shown="True" w1906 {
          tunnel: w1902 -> [w1918 w1921]
          tunnel: w1907 -> [_ w1920]
          tunnel: [w1918 w1919] -> w1905
          frame False {
          }
          frame True {
            n689 = Build Array (concatenate)(w1921, w1920) -> (w1919:dbl[])
          }
        }
        "Last Data \n(USB6218)" <- w1905
      }
      frame True {
        n690 = local read "RUN Identifier"() -> (w1922:string)
        n691 = call-dynamic "USBData_initialize.vi"("USBData in"=w1927, "SeriesSetting"="USB6218 Config", "BasePath"=w1926, "RunIdentifier"=w1922, "FileName"="InstName (USB6218)", "error in (no error)"=w1925) -> ("Status"=w1923:T6, "USBData out"=w1939:refnum<class "USBData.lvclass">, "error out"=w1940:errorcluster)  [unwired: 5 in, 2 out]
        n692 = local write "USB6218 Status"(w1923) -> ()
        n693 = call "USBData_read.vi"("USBData in"=w1939, "error in (no error)"=w1940) -> ("Status"=w1930:T6, "USBData out"=w1936:refnum<class "USBData.lvclass">, "Data"=w1937:T27, "Basic"=w1931:T28, "error out"=w1938:errorcluster)  [unwired: 2 in, 2 out]
        n694 = local write "USB6218 Status"(w1930) -> ()
        n695 = Unbundle By Name(w1931) -> ("ReadLeakDet?"=w1935:bool, "Labels"=w1929:string[])
        n696 = Array Size(array=w1929) -> (size(s)=w1934:i32)
        n697 = case shown="True" w1935 {
          tunnel: w1934 -> [w1941 w1943]
          tunnel: [w1941 w1942] -> w1932
          frame False {
          }
          frame True {
            n698 = Add(x=w1943, y=1) -> (x+y=w1942:i32)
          }
        }
        n699 = Initialize Array(TRUE ("Activate 2"), w1932) -> ()  [unwired: 1 out]
      }
    }
    "error out (USB6218)" <- w1182
    n700 = case shown="False" w1144 {
      frame False {
      }
      frame True {
        n701 = local read "RUN label"() -> (w1321:string)
        n702 = Get Date/Time In Seconds() -> (seconds since 1Jan1904=w1325:timestamp)
        n703 = call "LV_UNIXTIME.vi"("current time"=w1325) -> ("date/time string"=w1324:string)  [unwired: 9 in, 1 out]
        n704 = Concatenate Strings(w1324, "_" ("string"), w1321) -> (→"RUN Identifier" →"RUN Identifier 2" →"RUN Identifier 3" →"RUN Identifier 4" →"RUN Identifier 5" →"RUN Identifier 6" →"RUN Identifier 7":string)
      }
    }
    n705 = Equal?(x=w1154, y=i64 0) -> (x = y?=w1151:bool)
    n706 = local read "LastData (LSI218)"() -> (w1164:dbl[])
    n707 = local read "Last Data \nLSI336"() -> (w1163:dbl[])
    n708 = And(x="Analog Out ON?", y=w1144) -> (x .and. y?=w1180:bool)
    n709 = And(x=w1151, y="Automatic \nScreenshots?") -> (x .and. y?=w1150:bool)
    n710 = Build Array (concatenate)(w1164, w1163) -> (w1162:dbl[])
    "AllTemperatures" <- w1162
    n711 = Build Array (concatenate)(w1166, w1167) -> (w1165:T19)
    "TempSensorsLocations" <- w1165
    n712 = case shown="True" w1180 {
      tunnel: w1141 -> [_ w1714]
      tunnel: [w1690 w1705] -> w1179
      tunnel: w1178 -> [w1690 w1704]
      frame False {
      }
      frame True {
        w1697 = "_raw" ("string")
        w1721 = 10.0 ("V_lim_max")
        w1720 = 0.0 ("V_lim_min")
        w1719 = -1 items=["Default"=-1, "RSE"=10083, "Differential"=10106, "Pseudodifferential"=12529] ("output terminal configuration")
        w1718 = 10348 items=["Volts"=10348, "From Custom Scale"=10065] ("units")
        n713 = local read "RUN Identifier"() -> (w1703:string)
        n714 = Concatenate Strings(w1703, "_AO" ("string")) -> (w1723:string)
        n715 = Concatenate Strings(w1703, "_", "USB_AOUT.csv" ("string")) -> (w1715:string)
        n716 = Array To Cluster(array="AOUT Labels") -> (cluster=w1701:T29)
        n717 = Unbundle By Name(w1701) -> ("AOUT Labels[0]"=w1700:string, "AOUT Labels[1]"=w1698:string)
        n718 = Build Path(base path=w1714, name or relative path=w1715) -> (appended path=w1711:path)
        n719 = Concatenate Strings(w1700, w1697) -> (w1699:string)
        n720 = Concatenate Strings(w1698, w1697) -> (w1696:string)
        n721 = Open/Create/Replace File(file path (use dialog)=w1711, operation (0:open)=T25."open or create") -> (refnum out=w1709:refnum<file>)  [unwired: 4 in, 2 out]
        n722 = Build Array(w1700, w1698, w1699, w1696) -> (w1707:string[])
        n723 = call "FileIntialize.vi"("Error In"=w1704, "Labels"=w1707, "refnum in"=w1709) -> ("Error Out"=w1706:errorcluster, "File Refnum"=→"File Refn USB AO":refnum<file>)  [unwired: 7 in]
        n724 = call <vilib>:"DAQmx Create Task.vi"("new task name"=w1723, "auto cleanup"=FALSE, "error in"=w1706) -> ("task out"=w1722:refnum<k21>, "error out"=w1724:errorcluster)  [unwired: 11 in]
        n725 = Index Array(array="AOUT assignment", index #1=0 ("index"), index #2=1 ("index")) -> (element #1=w1693:tag, element #2=w1691:tag)
        n726 = call-poly <vilib>:"DAQmx Create Virtual Channel.vi"("task in"=w1722, "maximum value"=w1721, "minimum value"=w1720, "output terminal configuration"=w1719, "physical channels"=w1693, "units"=w1718, "error in"=w1724) -> ("task out"=w1726:refnum<k21>, "error out"=w1727:errorcluster)  [unwired: 7 in]
        n727 = call-poly <vilib>:"DAQmx Create Virtual Channel.vi"("task in"=w1726, "maximum value"=w1721, "minimum value"=w1720, "physical channels"=w1691, "error in"=w1727) -> ("task out"=w1729:refnum<k21>, "error out"=w1728:errorcluster)  [unwired: 9 in]
        n728 = call <vilib>:"DAQmx Start Task.vi"("task/channels in"=w1729, "error in"=w1728) -> ("task out"=→"AO task out":refnum<k21>, "error out"=w1705:errorcluster)  [unwired: 12 in]
      }
    }
    "error out (USB6210/6218 AOUT)" <- w1179
    n729 = case shown="True" w1150 {
      frame False {
      }
      frame True {
        n730 = flat-sequence {
          frame #0 {
            n731 = property on="Frontpanel screenshots" class="Bool (strict)"("Val(Sgnl)"=TRUE ("Value (Signaling)")) -> ()  [unwired: 2 in, 2 out]
          }
        }
      }
    }
    n732 = flat-sequence {
      tunnel: w1162 -> [w1331]
      tunnel: w1165 -> [w1332]
      tunnel: w1157 -> [w1584]
      tunnel: w1156 -> [w1583]
      frame #0 {
        n733 = stacked-sequence {
          tunnel: w1332 -> [w1337 w1342 w1347 w1352 w1357 w1362 w1367 w1372 w1377 w1382 w1387 w1392 w1397 w1402 w1407 w1412 w1417 w1422 w1427 w1432 w1437 w1442 w1447 w1452 w1457 w1462 w1467 w1472 w1477 w1482 w1487 w1492 w1497 w1502 w1507 w1512 w1517 w1522 w1527 w1532 w1537 w1542 w1547 w1552 w1557 w1562 w1567 w1572 w1577 w1582]
          tunnel: w1331 -> [w1335 w1340 w1345 w1350 w1355 w1360 w1365 w1370 w1375 w1380 w1385 w1390 w1395 w1400 w1405 w1410 w1415 w1420 w1425 w1430 w1435 w1440 w1445 w1450 w1455 w1460 w1465 w1470 w1475 w1480 w1485 w1490 w1495 w1500 w1505 w1510 w1515 w1520 w1525 w1530 w1535 w1540 w1545 w1550 w1555 w1560 w1565 w1570 w1575 w1580]
          frame #0 {
            n734 = Search 1D Array(1D array=w1337, element=T14."T3He1-1" ("SensorLocations")) -> (index of element=w1334:i32)  [unwired: 1 in]
            n735 = Index Array(array=w1335, index=w1334) -> (element=→"T3He1-1":dbl)
          }
          frame #1 {
            n736 = Search 1D Array(1D array=w1342, element=T14."T3He1-2" ("SensorLocations")) -> (index of element=w1339:i32)  [unwired: 1 in]
            n737 = Index Array(array=w1340, index=w1339) -> (element=→"T3He1-2":dbl)
          }
          frame #2 {
            n738 = Search 1D Array(1D array=w1347, element=T14."T3He1-3" ("SensorLocations")) -> (index of element=w1344:i32)  [unwired: 1 in]
            n739 = Index Array(array=w1345, index=w1344) -> (element=→"T3He1-3":dbl)
          }
          frame #3 {
            n740 = Search 1D Array(1D array=w1352, element=T14."T3He1-4" ("SensorLocations")) -> (index of element=w1349:i32)  [unwired: 1 in]
            n741 = Index Array(array=w1350, index=w1349) -> (element=→"T3He1-4":dbl)
          }
          frame #4 {
            n742 = Search 1D Array(1D array=w1357, element=T14."T3He2-1" ("SensorLocations")) -> (index of element=w1354:i32)  [unwired: 1 in]
            n743 = Index Array(array=w1355, index=w1354) -> (element=→"T3He2-1":dbl)
          }
          frame #5 {
            n744 = Search 1D Array(1D array=w1362, element=T14."T3He2-2" ("SensorLocations")) -> (index of element=w1359:i32)  [unwired: 1 in]
            n745 = Index Array(array=w1360, index=w1359) -> (element=→"T3He2-2":dbl)
          }
          frame #6 {
            n746 = Search 1D Array(1D array=w1367, element=T14."T3He3" ("SensorLocations")) -> (index of element=w1364:i32)  [unwired: 1 in]
            n747 = Index Array(array=w1365, index=w1364) -> (element=→"T3He3":dbl)
          }
          frame #7 {
            n748 = Search 1D Array(1D array=w1372, element=T14."T3He4" ("SensorLocations")) -> (index of element=w1369:i32)  [unwired: 1 in]
            n749 = Index Array(array=w1370, index=w1369) -> (element=→"T3He4":dbl)
          }
          frame #8 {
            n750 = Search 1D Array(1D array=w1377, element=T14."T3He5" ("SensorLocations")) -> (index of element=w1374:i32)  [unwired: 1 in]
            n751 = Index Array(array=w1375, index=w1374) -> (element=→"T3He5":dbl)
          }
          frame #9 {
            n752 = Search 1D Array(1D array=w1382, element=T14."T3He6-1" ("SensorLocations")) -> (index of element=w1379:i32)  [unwired: 1 in]
            n753 = Index Array(array=w1380, index=w1379) -> (element=→"T3He6-1" →"T3He6-1/6-2 (HEX1)":dbl)
          }
          frame #10 {
            n754 = Search 1D Array(1D array=w1387, element=T14."T3He6-2" ("SensorLocations")) -> (index of element=w1384:i32)  [unwired: 1 in]
            n755 = Index Array(array=w1385, index=w1384) -> (element=→"T3He6-2" →"T3He6-1/6-2 (3He pot) 2":dbl)
          }
          frame #11 {
            n756 = Search 1D Array(1D array=w1392, element=T14."T3He7-1" ("SensorLocations")) -> (index of element=w1389:i32)  [unwired: 1 in]
            n757 = Index Array(array=w1390, index=w1389) -> (element=→"T3He7-1" →"T3He7-1/7-2 (HEX1)":dbl)
          }
          frame #12 {
            n758 = Search 1D Array(1D array=w1397, element=T14."T3He7-2" ("SensorLocations")) -> (index of element=w1394:i32)  [unwired: 1 in]
            n759 = Index Array(array=w1395, index=w1394) -> (element=→"T3He7-2" →"T3He7-1/6-2 (3He pot) 2":dbl)
          }
          frame #13 {
            n760 = Search 1D Array(1D array=w1402, element=T14."T3He8" ("SensorLocations")) -> (index of element=w1399:i32)  [unwired: 1 in]
            n761 = Index Array(array=w1400, index=w1399) -> (element=→"T3He8":dbl)
          }
          frame #14 {
            n762 = Search 1D Array(1D array=w1407, element=T14."T3He9" ("SensorLocations")) -> (index of element=w1404:i32)  [unwired: 1 in]
            n763 = Index Array(array=w1405, index=w1404) -> (element=→"T3He9":dbl)
          }
          frame #15 {
            n764 = Search 1D Array(1D array=w1412, element=T14."T3He10" ("SensorLocations")) -> (index of element=w1409:i32)  [unwired: 1 in]
            n765 = Index Array(array=w1410, index=w1409) -> (element=→"T3He10":dbl)
          }
          frame #16 {
            n766 = Search 1D Array(1D array=w1417, element=T14."T4He1" ("SensorLocations")) -> (index of element=w1414:i32)  [unwired: 1 in]
            n767 = Index Array(array=w1415, index=w1414) -> (element=→"T4He1" →"T4He1 (4K reservoir )":dbl)
          }
          frame #17 {
            n768 = Search 1D Array(1D array=w1422, element=T14."T4He2-1" ("SensorLocations")) -> (index of element=w1419:i32)  [unwired: 1 in]
            n769 = Index Array(array=w1420, index=w1419) -> (element=→"T4He2-1":dbl)
          }
          frame #18 {
            n770 = Search 1D Array(1D array=w1427, element=T14."T4He2-2" ("SensorLocations")) -> (index of element=w1424:i32)  [unwired: 1 in]
            n771 = Index Array(array=w1425, index=w1424) -> (element=→"T4He2-2":dbl)
          }
          frame #19 {
            n772 = Search 1D Array(1D array=w1432, element=T14."T4He3-1" ("SensorLocations")) -> (index of element=w1429:i32)  [unwired: 1 in]
            n773 = Index Array(array=w1430, index=w1429) -> (element=→"T4He3-1":dbl)
          }
          frame #20 {
            n774 = Search 1D Array(1D array=w1437, element=T14."T4He3-2" ("SensorLocations")) -> (index of element=w1434:i32)  [unwired: 1 in]
            n775 = Index Array(array=w1435, index=w1434) -> (element=→"T4He3-2":dbl)
          }
          frame #21 {
            n776 = Search 1D Array(1D array=w1442, element=T14."T4He3-3" ("SensorLocations")) -> (index of element=w1439:i32)  [unwired: 1 in]
            n777 = Index Array(array=w1440, index=w1439) -> (element=→"T4He3-3":dbl)
          }
          frame #22 {
            n778 = Search 1D Array(1D array=w1447, element=T14."T4He3-4" ("SensorLocations")) -> (index of element=w1444:i32)  [unwired: 1 in]
            n779 = Index Array(array=w1445, index=w1444) -> (element=→"T4He3-4":dbl)
          }
          frame #23 {
            n780 = Search 1D Array(1D array=w1452, element=T14."T4He4" ("SensorLocations")) -> (index of element=w1449:i32)  [unwired: 1 in]
            n781 = Index Array(array=w1450, index=w1449) -> (element=→"T4He4":dbl)
          }
          frame #24 {
            n782 = Search 1D Array(1D array=w1457, element=T14."T4He5" ("SensorLocations")) -> (index of element=w1454:i32)  [unwired: 1 in]
            n783 = Index Array(array=w1455, index=w1454) -> (element=→"T4He5":dbl)
          }
          frame #25 {
            n784 = Search 1D Array(1D array=w1462, element=T14."T4He6" ("SensorLocations")) -> (index of element=w1459:i32)  [unwired: 1 in]
            n785 = Index Array(array=w1460, index=w1459) -> (element=→"T4He6":dbl)
          }
          frame #26 {
            n786 = Search 1D Array(1D array=w1467, element=T14."T4He7" ("SensorLocations")) -> (index of element=w1464:i32)  [unwired: 1 in]
            n787 = Index Array(array=w1465, index=w1464) -> (element=→"T4He7":dbl)
          }
          frame #27 {
            n788 = Search 1D Array(1D array=w1472, element=T14."T4He8" ("SensorLocations")) -> (index of element=w1469:i32)  [unwired: 1 in]
            n789 = Index Array(array=w1470, index=w1469) -> (element=→"T4He8":dbl)
          }
          frame #28 {
            n790 = Search 1D Array(1D array=w1477, element=T14."T4He9" ("SensorLocations")) -> (index of element=w1474:i32)  [unwired: 1 in]
            n791 = Index Array(array=w1475, index=w1474) -> (element=→"T4He9":dbl)
          }
          frame #29 {
            n792 = Search 1D Array(1D array=w1482, element=T14."T4He10" ("SensorLocations")) -> (index of element=w1479:i32)  [unwired: 1 in]
            n793 = Index Array(array=w1480, index=w1479) -> (element=→"T4He10":dbl)
          }
          frame #30 {
            n794 = Search 1D Array(1D array=w1487, element=T14."T1K1" ("SensorLocations")) -> (index of element=w1484:i32)  [unwired: 1 in]
            n795 = Index Array(array=w1485, index=w1484) -> (element=→"T1K1":dbl)
          }
          frame #31 {
            n796 = Search 1D Array(1D array=w1492, element=T14."T1K2" ("SensorLocations")) -> (index of element=w1489:i32)  [unwired: 1 in]
            n797 = Index Array(array=w1490, index=w1489) -> (element=→"T1K2":dbl)
          }
          frame #32 {
            n798 = Search 1D Array(1D array=w1497, element=T14."T1K3-1" ("SensorLocations")) -> (index of element=w1494:i32)  [unwired: 1 in]
            n799 = Index Array(array=w1495, index=w1494) -> (element=→"T1K3-1" →"T1K3-1/3-2 (1K pot)":dbl)
          }
          frame #33 {
            n800 = Search 1D Array(1D array=w1502, element=T14."T1K3-2" ("SensorLocations")) -> (index of element=w1499:i32)  [unwired: 1 in]
            n801 = Index Array(array=w1500, index=w1499) -> (element=→"T1K3-2" →"T1K3-1/3-2 (1K pot) 2":dbl)
          }
          frame #34 {
            n802 = Search 1D Array(1D array=w1507, element=T14."T1K4" ("SensorLocations")) -> (index of element=w1504:i32)  [unwired: 1 in]
            n803 = Index Array(array=w1505, index=w1504) -> (element=→"T1K4":dbl)
          }
          frame #35 {
            n804 = Search 1D Array(1D array=w1512, element=T14."T1K5" ("SensorLocations")) -> (index of element=w1509:i32)  [unwired: 1 in]
            n805 = Index Array(array=w1510, index=w1509) -> (element=→"T1K5":dbl)
          }
          frame #36 {
            n806 = Search 1D Array(1D array=w1517, element=T14."T1K6" ("SensorLocations")) -> (index of element=w1514:i32)  [unwired: 1 in]
            n807 = Index Array(array=w1515, index=w1514) -> (element=→"T1K6":dbl)
          }
          frame #37 {
            n808 = Search 1D Array(1D array=w1522, element=T14."TIP1" ("SensorLocations")) -> (index of element=w1519:i32)  [unwired: 1 in]
            n809 = Index Array(array=w1520, index=w1519) -> (element=→"TIP1":dbl)
          }
          frame #38 {
            n810 = Search 1D Array(1D array=w1527, element=T14."TIP2" ("SensorLocations")) -> (index of element=w1524:i32)  [unwired: 1 in]
            n811 = Index Array(array=w1525, index=w1524) -> (element=→"TIP2":dbl)
          }
          frame #39 {
            n812 = Search 1D Array(1D array=w1532, element=T14."TIP3" ("SensorLocations")) -> (index of element=w1529:i32)  [unwired: 1 in]
            n813 = Index Array(array=w1530, index=w1529) -> (element=→"TIP3":dbl)
          }
          frame #40 {
            n814 = Search 1D Array(1D array=w1537, element=T14."TIP4" ("SensorLocations")) -> (index of element=w1534:i32)  [unwired: 1 in]
            n815 = Index Array(array=w1535, index=w1534) -> (element=→"TIP4":dbl)
          }
          frame #41 {
            n816 = Search 1D Array(1D array=w1542, element=T14."TIP5" ("SensorLocations")) -> (index of element=w1539:i32)  [unwired: 1 in]
            n817 = Index Array(array=w1540, index=w1539) -> (element=→"TIP5":dbl)
          }
          frame #42 {
            n818 = Search 1D Array(1D array=w1547, element=T14."TIP6" ("SensorLocations")) -> (index of element=w1544:i32)  [unwired: 1 in]
            n819 = Index Array(array=w1545, index=w1544) -> (element=→"TIP6":dbl)
          }
          frame #43 {
            n820 = Search 1D Array(1D array=w1552, element=T14."TIP7" ("SensorLocations")) -> (index of element=w1549:i32)  [unwired: 1 in]
            n821 = Index Array(array=w1550, index=w1549) -> (element=→"TIP7":dbl)
          }
          frame #44 {
            n822 = Search 1D Array(1D array=w1557, element=T14."TTH1" ("SensorLocations")) -> (index of element=w1554:i32)  [unwired: 1 in]
            n823 = Index Array(array=w1555, index=w1554) -> (element=→"TTH1":dbl)
          }
          frame #45 {
            n824 = Search 1D Array(1D array=w1562, element=T14."TTH2" ("SensorLocations")) -> (index of element=w1559:i32)  [unwired: 1 in]
            n825 = Index Array(array=w1560, index=w1559) -> (element=→"TTH2":dbl)
          }
          frame #46 {
            n826 = Search 1D Array(1D array=w1567, element=T14."TTH3" ("SensorLocations")) -> (index of element=w1564:i32)  [unwired: 1 in]
            n827 = Index Array(array=w1565, index=w1564) -> (element=→"TTH3":dbl)
          }
          frame #47 {
            n828 = Search 1D Array(1D array=w1572, element=T14."TTH4" ("SensorLocations")) -> (index of element=w1569:i32)  [unwired: 1 in]
            n829 = Index Array(array=w1570, index=w1569) -> (element=→"TTH4":dbl)
          }
          frame #48 {
            n830 = Search 1D Array(1D array=w1577, element="SensorLocation 1") -> (index of element=w1574:i32)  [unwired: 1 in]
            n831 = Index Array(array=w1575, index=w1574) -> (element=→"Temperature 1":dbl)
          }
          frame #49 {
            n832 = Search 1D Array(1D array=w1582, element="SensorLocation 2") -> (index of element=w1579:i32)  [unwired: 1 in]
            n833 = Index Array(array=w1580, index=w1579) -> (element=→"Temperature 2":dbl)
          }
        }
      }
      frame #1 {
        n834 = stacked-sequence {
          tunnel: w1584 -> [w1589 w1594 w1599 w1604 w1609 w1614 w1619 w1624 w1629 w1634 w1639 w1644 w1649 w1654 w1659 w1664 w1669 w1674 w1679]
          tunnel: w1583 -> [w1586 w1592 w1598 w1603 w1608 w1612 w1617 w1622 w1627 w1632 w1637 w1642 w1646 w1651 w1656 w1661 w1666 w1671 _]
          tunnel: w1583 -> [_ _ _ _ _ _ _ _ _ _ _ _ _ _ _ _ _ _ w1677]
          frame #0 {
            n835 = Search 1D Array(1D array=w1589, element="Insulation vacuum") -> (index of element=w1587:i32)  [unwired: 1 in]
            n836 = Index Array(array=w1586, index=w1587) -> (element=→"P_ins" →"P (insulation)":dbl)
          }
          frame #1 {
            n837 = Search 1D Array(1D array=w1594, element="4K reservoir pressure") -> (index of element=w1591:i32)  [unwired: 1 in]
            n838 = Index Array(array=w1592, index=w1591) -> (element=→"P_4Kres" →"P (4K reservoir)":dbl)
          }
          frame #2 {
            n839 = Search 1D Array(1D array=w1599, element="3He inlet pressure") -> (index of element=w1597:i32)  [unwired: 1 in]
            n840 = Index Array(array=w1598, index=w1597) -> (element=→"P_3HeIN" →"P (3He IN)":dbl)
          }
          frame #3 {
            n841 = Search 1D Array(1D array=w1604, element="Shield return press.") -> (index of element=w1602:i32)  [unwired: 1 in]
            n842 = Index Array(array=w1603, index=w1602) -> (element=→"P_SldRTN" →"P (shield return)":dbl)
          }
          frame #4 {
            n843 = Search 1D Array(1D array=w1609, element="3He pot pressure") -> (index of element=w1607:i32)  [unwired: 1 in]
            n844 = Index Array(array=w1608, index=w1607) -> (element=→"P_3Hepot" →"P (3He pot)":dbl)
          }
          frame #5 {
            n845 = Search 1D Array(1D array=w1614, element="1Kpot pressure") -> (index of element=w1611:i32)  [unwired: 1 in]
            n846 = Index Array(array=w1612, index=w1611) -> (element=→"P_1Kpot" →"P (1K pot)":dbl)
          }
          frame #6 {
            n847 = Search 1D Array(1D array=w1619, element="Dewar pressure") -> (index of element=w1616:i32)  [unwired: 1 in]
            n848 = Index Array(array=w1617, index=w1616) -> (element=→"P_Dewar" →"P (Dewar)":dbl)
          }
          frame #7 {
            n849 = Search 1D Array(1D array=w1624, element="HEX7 out pressure") -> (index of element=w1621:i32)  [unwired: 1 in]
            n850 = Index Array(array=w1622, index=w1621) -> (element=→"P_HEX7OUT" →"P (HEX7 out)":dbl)
          }
          frame #8 {
            n851 = Search 1D Array(1D array=w1629, element="Diff pressure HEX4") -> (index of element=w1626:i32)  [unwired: 1 in]
            n852 = Index Array(array=w1627, index=w1626) -> (element=→"DP_HEX4" →"DP HEX4":dbl)
          }
          frame #9 {
            n853 = Search 1D Array(1D array=w1634, element="Diff pressure HEX5") -> (index of element=w1631:i32)  [unwired: 1 in]
            n854 = Index Array(array=w1632, index=w1631) -> (element=→"DP_HEX5" →"DP HEX5":dbl)
          }
          frame #10 {
            n855 = Search 1D Array(1D array=w1639, element="3He pump exhaust flow") -> (index of element=w1636:i32)  [unwired: 1 in]
            n856 = Index Array(array=w1637, index=w1636) -> (element=→"F_1" →"F1 (3He pump exhaust) flow":dbl)
          }
          frame #11 {
            n857 = Search 1D Array(1D array=w1644, element="Shield flow") -> (index of element=w1641:i32)  [unwired: 1 in]
            n858 = Index Array(array=w1642, index=w1641) -> (element=→"F_2" →"F2 (shield flow)":dbl)
          }
          frame #12 {
            n859 = Search 1D Array(1D array=w1649, element="4He return flow from HEX7") -> (index of element=w1647:i32)  [unwired: 1 in]
            n860 = Index Array(array=w1646, index=w1647) -> (element=→"F_3" →"F3 (4He rtn flw via HEX7)":dbl)
          }
          frame #13 {
            n861 = Search 1D Array(1D array=w1654, element="3He incoming flow into HEX7") -> (index of element=w1652:i32)  [unwired: 1 in]
            n862 = Index Array(array=w1651, index=w1652) -> (element=→"F_4" →"F4 (3He in to HEX7)":dbl)
          }
          frame #14 {
            n863 = Search 1D Array(1D array=w1659, element="1Kpot pump exhaust flow") -> (index of element=w1657:i32)  [unwired: 1 in]
            n864 = Index Array(array=w1656, index=w1657) -> (element=→"F_5" →"F5 (1K pump ex.)":dbl)
          }
          frame #15 {
            n865 = Search 1D Array(1D array=w1664, element="4K reservoir level") -> (index of element=w1662:i32)  [unwired: 1 in]
            n866 = Index Array(array=w1661, index=w1662) -> (element=→"L3" →"He level (4K)":dbl)
          }
          frame #16 {
            n867 = Search 1D Array(1D array=w1669, element="1K pot level") -> (index of element=w1667:i32)  [unwired: 1 in]
            n868 = Index Array(array=w1666, index=w1667) -> (element=→"L(1K) (a1)" →"He level (1K)":dbl)
          }
          frame #17 {
            n869 = Search 1D Array(1D array=w1674, element="1K pot (b)") -> (index of element=w1672:i32)  [unwired: 1 in]
            n870 = Index Array(array=w1671, index=w1672) -> (element=→"1K pot(b1)" →"He level (1K) b":dbl)
          }
          frame #18 {
            n871 = case shown="False" TRUE {
              tunnel: w1679 -> [w1684 _]
              tunnel: "3He pot" -> [w1683 w1688]
              tunnel: w1677 -> [w1681 _]
              tunnel: [w1680 w1687] -> w1676
              frame False {
                n872 = Search 1D Array(1D array=w1684, element=w1683) -> (index of element=w1682:i32)  [unwired: 1 in]
                n873 = Index Array(array=w1681, index=w1682) -> (element=w1680:dbl)
              }
              frame True {
                n874 = local read "Labels (HP34401 LM)"() -> (w1689:string[])
                n875 = local read "LastData (HP34401 LM)"() -> (w1685:dbl[])
                n876 = Search 1D Array(1D array=w1689, element=w1688) -> (index of element=w1686:i32)  [unwired: 1 in]
                n877 = Index Array(array=w1685, index=w1686) -> (element=w1687:dbl)
              }
            }
            "3He pot level" <- w1676
            "He level (3He)" <- w1676
          }
        }
      }
    }
    n878 = case shown="True" w1144 {
      tunnel: [w2248 w2260] -> w1204
      tunnel: [w2238 w2259] -> w1212
      tunnel: [w2247 w2258] -> w1205
      tunnel: [w2246 timestamp[] [] ("TimeArray")] -> w1174
      tunnel: [w2245 dbl[][] [] ("DataArray")] -> w1172
      tunnel: w1214 -> [w2244 w2255]
      tunnel: w1213 -> [w2243 w2254]
      tunnel: w1138 -> [w2239 _]
      tunnel: w1141 -> [_ w2249]
      frame False {
        n879 = local read "Record interval"() -> (w2236:i64)
        n880 = call-dynamic "LSI336Data_measure.vi"("LSI336Data in"=w2244, "MeasurementIndex"=w2239, "error in (no error)"=w2243, "save every ... measurements"=w2236) -> ("Active?"=→"Active?\n(LSI336)":bool[], "TimeMeasuremeent"=→"Time of Last Measurement (LSI336)":timestamp, "LSI336Data out"=w2247:refnum<class "LSI336Data.lvclass">, "LastData"=→"Last Data \nLSI336":dbl[], "LastMeasurementConfig"=→"LastMeasurementConfig (336)":T18, "DataArray"=w2245:dbl[][], "Status"=w2238:u16, "TimeArray"=w2246:timestamp[], "error out"=w2248:errorcluster)  [unwired: 3 in]
      }
      frame True {
        n881 = local read "RUN Identifier"() -> (w2250:string)
        n882 = call-dynamic "LSI336Data_initialize.vi"("LSI336Data in"=w2255, "RunIdentifier"=w2250, "InstName"="InstName (LSI336)", "FileFormat"="FileFormat (336)", "LSI336Settings(X, Y)"="LSI336Settings(X,Y)", "error in (no error)"=w2254, "base path"=w2249) -> ("LSI336Data out"=w2258:refnum<class "LSI336Data.lvclass">, "Status"=w2259:T7, "AllLabels"=→"Labels LSI336":string[], "error out"=w2260:errorcluster)  [unwired: 5 in]
      }
    }
    "LSI336 Status" <- w1212
    "error out (LSI336)" <- w1204
    "TimeArray (LSI336)" <- w1174
    "DataArray (336)" <- w1172
    n883 = local read "Labels (HP34401 LM) 2"() -> (w1137:string[])
    n884 = case shown="False" w1144 {
      tunnel: [w2353 w2368] -> w1217
      tunnel: [w2348 w2367] -> w1234
      tunnel: [w2351 w2366] -> w1218
      tunnel: w1138 -> [w2352 _]
      tunnel: w1233 -> [w2342 w2361]
      tunnel: w1232 -> [w2343 w2360]
      tunnel: w1141 -> [_ w2359]
      tunnel: [w2340 timestamp[] [] ("TimeArray")] -> w1231
      tunnel: [w2339 dbl[][] [] ("DataArray")] -> w1230
      frame False {
        w2346 = 24 ("index")
        n885 = local read "Record interval"() -> (w2337:i64)
        n886 = call-dynamic "LSI218Data_measure.vi"("LSI218Data in"=w2343, "MeasurementIndex"=w2352, "error in (no error)"=w2342, "save every ... measurements"=w2337) -> ("TimeMeasuremeent"=→"Time of Last Measurement (LSI218)":timestamp, "Active?"=w2347:bool[], "LSI218Data out"=w2351:refnum<class "LSI218Data.lvclass">, "LastMeasurementConfig"=→"LastMeasurementConfig (218)":T18, "LastData"=w2341:dbl[], "Status"=w2348:u16, "TimeArray"=w2340:timestamp[], "DataArray"=w2339:dbl[][], "error out"=w2353:errorcluster)  [unwired: 3 in]
        "LastData (LSI218)" <- w2341
        n887 = Split 1D Array(array=w2347, index=w2346) -> (first subarray=→"Active?\n (1)":bool[], second subarray=→"Active?\n(2)":bool[])
        n888 = Split 1D Array(array=w2341, index=w2346) -> (first subarray=→"Last Data \nLSI218 (1)":dbl[], second subarray=→"Last Data \nLSI218 (2)":dbl[])
      }
      frame True {
        n889 = local read "RUN Identifier"() -> (w2355:string)
        n890 = call-dynamic "LSI218Data_initialize.vi"("LSI218Settings(A-F)"="LSI218Settings(A-F)", "FileFormat"="FileFormat (218)", "base path"=w2359, "error in (no error)"=w2361, "InstName"="InstName (LSI218)", "RunIdentifier"=w2355, "LSI218Data in"=w2360) -> ("error out"=w2368:errorcluster, "Status"=w2367:T7, "AllLabels"=w2358:string[], "LSI218Data out"=w2366:refnum<class "LSI218Data.lvclass">)  [unwired: 1 in]
        n891 = Split 1D Array(array=w2358, index=24) -> (first subarray=→"Labels LSI218 (1)":string[], second subarray=→"Labels LSI218 (2)":string[])
      }
    }
    "LSI218 Status" <- w1234
    "error out (LSI218)" <- w1217
    n892 = case shown="True" w1144 {
      tunnel: w1143 -> [w1306 w1320]
      tunnel: [w1303 w1319] -> w1142
      tunnel: w1141 -> [_ w1317]
      tunnel: w1140 -> [w1305 w1316]
      tunnel: [w1302 w1313] -> w1139
      tunnel: w1138 -> [w1304 _]
      tunnel: [w1300 dbl[][] [] ("LastDataArray")] -> w1135
      tunnel: [w1299 timestamp[] [] ("LastTimeArray")] -> w1133
      frame False {
        n893 = call-dynamic "LMData_measure.vi"("error in (no error)"=w1305, "MeasurementInterval(>0)"="LM measurement interval (>0)", "MeasurementIndex"=w1304, "LMData in"=w1306) -> ("error out"=w1302:errorcluster, "LastDataArray"=w1300:dbl[][], "LastMeasurement"=→"LastData (HP34401 LM)":dbl[], "LMData out"=w1303:refnum<class "LMData.lvclass">, "LastTimeArray"=w1299:timestamp[])  [unwired: 3 in]
      }
      frame True {
        n894 = local read "RUN Identifier"() -> (w1318:string)
        n895 = call-dynamic "LMData_initialize.vi"("LMData in"=w1320, "VISA resource name"="VISA (HP34401 LM)", "Labels"="Labels (HP34401 LM)", "FileFormat"="FileFormat (HP34401 LM)", "RunIdentifier"=w1318, "InstName"="InstName (HP34401 LM)", "base path"=w1317, "error in (no error)"=w1316, "LevelCalibration (R0, R1, L0, L1)"="LevelCalibration (R0, R1, L0, L1)", "Active?"="Active? (HP34401 LM)") -> ("LMData out"=w1319:refnum<class "LMData.lvclass">, "error out"=w1313:errorcluster)  [unwired: 4 in]
        "Labels (HP34401 LM) 2" <- "Labels (HP34401 LM)"
      }
    }
    "error out (HP34401 LM)" <- w1139
    n896 = Array Size(array=w1137) -> (size(s)=w1136:i32)
    n897 = for {
      N: w1136 -> [_]
      tunnel: w1135 -> [w1260]
      shift-right: [w1247] -> w1129
      shift-left: w1134 -> [w1246]
      shift-right: [w1250] -> w1131
      shift-left: w1134 -> [w1251]
      shift-right: [w1254] -> w1132
      shift-left: w1134 -> [w1255]
      shift-right: [w1249] -> w1130
      shift-left: w1134 -> [w1248]
      tunnel: w1133 -> [w1258]
      i -> [w1259]
      n898 = local read "Plot selecter (HP34401A)\n    1      2     3     4"() -> (w1265:bool[][])
      n899 = Index Array(array=w1260, index (col)=w1259) -> (element=w1257:dbl[])  [unwired: 1 in]
      n900 = Bundle("LastTimeArray"=w1258, "LastDataArray"=w1257) -> (w1256:T30)  [unwired: 1 in]
      n901 = Index Array(array=w1265, index (row) #1=w1259, index (col) #1=0 ("disabled index (col)"), index (row) #2=w1259, index (col) #2=1 ("index (col)"), index (row) #3=w1259, index (col) #3=2 ("index (col)"), index (row) #4=w1259, index (col) #4=3 ("disabled index (col)")) -> (element #1=w1253:bool, element #2=w1252:bool, element #3=w1245:bool, element #4=w1244:bool)
      n902 = stacked-sequence {
        tunnel: w1256 -> [w1267 w1274 w1285 w1293]
        tunnel: w1255 -> [w1269 _ _ _]
        tunnel: [w1268 _ _ _] -> w1254
        tunnel: w1253 -> [w1266 _ _ _]
        tunnel: w1252 -> [_ w1277 _ _]
        tunnel: w1251 -> [_ w1276 _ _]
        tunnel: [_ w1275 _ _] -> w1250
        tunnel: [_ _ w1284 _] -> w1249
        tunnel: w1248 -> [_ _ w1283 _]
        tunnel: [_ _ _ w1292] -> w1247
        tunnel: w1246 -> [_ _ _ w1291]
        tunnel: w1245 -> [_ _ w1282 _]
        tunnel: w1244 -> [_ _ _ w1290]
        frame #0 {
          n903 = case shown="True" w1266 {
            tunnel: w1269 -> [w1270 w1273]
            tunnel: [w1270 w1272] -> w1268
            tunnel: w1267 -> [_ w1271]
            frame False {
            }
            frame True {
              n904 = Build Array (concatenate)(w1273, w1271) -> (w1272:T31)
            }
          }
        }
        frame #1 {
          n905 = case shown="True" w1277 {
            tunnel: [w1278 w1281] -> w1275
            tunnel: w1276 -> [w1278 w1280]
            tunnel: w1274 -> [_ w1279]
            frame False {
            }
            frame True {
              n906 = Build Array (concatenate)(w1280, w1279) -> (w1281:T31)
            }
          }
        }
        frame #2 {
          n907 = case shown="True" w1282 {
            tunnel: [w1286 w1289] -> w1284
            tunnel: w1285 -> [_ w1288]
            tunnel: w1283 -> [w1286 w1287]
            frame False {
            }
            frame True {
              n908 = Build Array (concatenate)(w1287, w1288) -> (w1289:T31)
            }
          }
        }
        frame #3 {
          n909 = case shown="True" w1290 {
            tunnel: [w1294 w1297] -> w1292
            tunnel: w1293 -> [_ w1296]
            tunnel: w1291 -> [w1294 w1295]
            frame False {
            }
            frame True {
              n910 = Build Array (concatenate)(w1295, w1296) -> (w1297:T31)
            }
          }
        }
      }
    }
    n911 = local read "Last Data \n(USB6210)"() -> (w1158:dbl[])
    n912 = local read "Last Data \n(USB6218)"() -> (w1159:dbl[])
    n913 = local read "All Labels (USB6210)"() -> (w1161:string[])
    n914 = local read "All Labels (USB6218)"() -> (w1160:string[])
    n915 = flat-sequence {
      tunnel: w1188 -> [w1748]
      tunnel: [w1743] -> w1187
      tunnel: [w1741] -> w1186
      tunnel: [w1740] -> w1185
      tunnel: [w1739] -> w1184
      tunnel: w1189 -> [w1735]
      frame #0 {
        w1742 = T26 [] ("appended array")
        n916 = Unbundle By Name(w1735) -> ("TimeArray"=w1731:timestamp[], "DataArrayConv"=w1746:dbl[][], "LDArray"=w1745:dbl[])
        "TimeArray (USB6218)" <- w1731
        n917 = Unbundle By Name(w1748) -> ("ReadLeakDet?"=w1747:bool, "LabelLD"=w1750:string, "Labels"=w1744:string[])  [unwired: 1 out]
        n918 = case shown="True" w1747 {
          tunnel: w1750 -> [_ w1758]
          tunnel: w1746 -> [w1752 w1757]
          tunnel: w1745 -> [_ w1756]
          tunnel: [w1752 w1755] -> w1733
          tunnel: w1744 -> [w1751 w1754]
          tunnel: [w1751 w1753] -> w1736
          frame False {
          }
          frame True {
            n919 = Build Array (concatenate)(w1757, w1756) -> (w1755:dbl[][])
            n920 = Build Array (concatenate)(w1754, w1758) -> (w1753:string[])
          }
        }
        "All Labels (USB6218)" <- w1736
        "DataArrayConv (USB6218)" <- w1733
        n921 = Array Size(array=w1731) -> (size(s)=→"TimeArray size (6218)":i32)
        n922 = local read "Plot selecter (USB6218)\n    1      2     3     4"() -> (w1738:bool[][])
        n923 = control-ref of="Plot selecter (USB6218)\n    1      2     3     4"() -> (w1734:refnum<vi>)
        n924 = Array Size(array=w1736) -> (size(s)=w1737:i32)
        n925 = Array Size(array=w1736) -> (size(s)=w1749:i32)
        n926 = Array Size(array=w1733) -> (size(s)=→"DataArraySize (6218)":i32[])
        n927 = property on="Property Node" class="Arr (strict)"(reference=w1734, "Number of Rows"=w1737) -> ()  [unwired: 1 in, 2 out]
        n928 = for {
          N: w1749 -> [_]
          tunnel: w1733 -> [w1779]
          tunnel: w1731 -> [w1780]
          shift-right: [w1774] -> w1741
          shift-left: w1742 -> [w1777]
          shift-right: [w1772] -> w1739
          shift-left: w1742 -> [w1775]
          shift-right: [w1773] -> w1743
          shift-left: w1742 -> [w1771]
          shift-right: [w1770] -> w1740
          shift-left: w1742 -> [w1769]
          tunnel: w1738 -> [w1768]
          i -> [w1763]
          n929 = Index Array(array=w1779, index (col)=w1763) -> (element=w1778:dbl[])  [unwired: 1 in]
          n930 = Index Array(array=w1768, index (row) #1=w1763, index (col) #1=0 ("index (row)"), index (row) #2=w1763, index (col) #2=1 ("index (row)"), index (row) #3=w1763, index (col) #3=2 ("index (row)"), index (row) #4=w1763, index (col) #4=3 ("index (row)")) -> (element #1=w1762:bool, element #2=w1761:bool, element #3=w1760:bool, element #4=w1759:bool)
          n931 = Bundle("TimeArray"=w1780, "DataArrayConv"=w1778) -> (w1776:T32)  [unwired: 1 in]
          n932 = stacked-sequence {
            tunnel: w1762 -> [w1784 _ _ _]
            tunnel: w1777 -> [_ w1792 _ _]
            tunnel: w1760 -> [_ _ w1800 _]
            tunnel: w1776 -> [w1781 w1790 w1799 w1805]
            tunnel: w1759 -> [_ _ _ w1808]
            tunnel: w1775 -> [_ _ _ w1807]
            tunnel: [_ _ _ w1806] -> w1772
            tunnel: [_ w1791 _ _] -> w1774
            tunnel: [w1783 _ _ _] -> w1773
            tunnel: w1771 -> [w1782 _ _ _]
            tunnel: [_ _ w1798 _] -> w1770
            tunnel: w1769 -> [_ _ w1797 _]
            tunnel: w1761 -> [_ w1789 _ _]
            frame #0 {
              n933 = case shown="True" w1784 {
                tunnel: [w1785 w1788] -> w1783
                tunnel: w1781 -> [_ w1787]
                tunnel: w1782 -> [w1785 w1786]
                frame False {
                }
                frame True {
                  n934 = Build Array (concatenate)(w1786, w1787) -> (w1788:T26)
                }
              }
            }
            frame #1 {
              n935 = case shown="True" w1789 {
                tunnel: w1792 -> [w1793 w1796]
                tunnel: [w1793 w1795] -> w1791
                tunnel: w1790 -> [_ w1794]
                frame False {
                }
                frame True {
                  n936 = Build Array (concatenate)(w1796, w1794) -> (w1795:T26)
                }
              }
            }
            frame #2 {
              n937 = case shown="True" w1800 {
                tunnel: [w1801 w1804] -> w1798
                tunnel: w1799 -> [_ w1803]
                tunnel: w1797 -> [w1801 w1802]
                frame False {
                }
                frame True {
                  n938 = Build Array (concatenate)(w1802, w1803) -> (w1804:T26)
                }
              }
            }
            frame #3 {
              n939 = case shown="True" w1808 {
                tunnel: [w1809 w1812] -> w1806
                tunnel: w1805 -> [_ w1811]
                tunnel: w1807 -> [w1809 w1810]
                frame False {
                }
                frame True {
                  n940 = Build Array (concatenate)(w1810, w1811) -> (w1812:T26)
                }
              }
            }
          }
        }
      }
    }
    n941 = case shown="True" "Digital Out ON?" {
      tunnel: w1144 -> [_ w1951]
      tunnel: w1194 -> [w1945 w1950]
      tunnel: [w1945 w1949] -> w1193
      tunnel: w1192 -> [_ w1948]
      tunnel: w1141 -> [_ w1947]
      tunnel: w1175 -> [_ w1946]
      frame False {
      }
      frame True {
        n942 = case shown="True" w1951 {
          tunnel: w1950 -> [w1969 w2155]
          tunnel: [w1969 w2162] -> w1949
          tunnel: w1948 -> [w1970 _]
          tunnel: w1947 -> [_ w2134]
          tunnel: w1946 -> [_ _]
          frame False {
            n943 = flat-sequence {
              frame #0 {
              }
            }
            n944 = case shown="\"USB6218AI\"" "AutoFill Source (P)" {
              tunnel: [w1973 w1974] -> w1955
              frame "USB6210", Default {
                n945 = local read "All Labels (USB6210)"() -> (w1973:string[])
              }
              frame "USB6218AI" {
                n946 = local read "All Labels (USB6218)"() -> (w1974:string[])
              }
            }
            n947 = case shown="\"USB6210\", Default" "AutoFill Source (L)" {
              tunnel: [w1971 w1972] -> w1952
              frame "USB6210", Default {
                n948 = local read "All Labels (USB6210)"() -> (w1971:string[])
              }
              frame "USB6218AI" {
                n949 = local read "All Labels (USB6218)"() -> (w1972:string[])
              }
            }
            n950 = Multiply(x="N for sampling", y=i64 2) -> (x*y=w1964:i64)
            n951 = local read "Cycle #"() -> (w1968:u32)
            n952 = Search 1D Array(1D array=w1955, element="Auto Fll Dewar P. label") -> (index of element=→"Target Index (P)":i32)  [unwired: 1 in]
            n953 = Search 1D Array(1D array=w1952, element="Auto Fll He L. label") -> (index of element=→"Target Index (L)":i32)  [unwired: 1 in]
            n954 = Add(x=w1964, y="Mov. Avg Interval") -> (x+y=w1966:i64)
            n955 = Greater?(x=w1968, y=w1966) -> (0:w1962:bool)
            n956 = And(x=w1962, y="Auto Fill ON?") -> (x .and. y?=w1960:bool)
            n957 = case shown="True" w1960 {
              tunnel: w1970 -> [_ w2008]
              tunnel: "Mov. Avg Interval" -> [_ w1994]
              tunnel: w1964 -> [_ w1981]
              tunnel: "N for sampling" -> [_ w1992]
              frame False {
              }
              frame True {
                n958 = local read "AutoFill Source (L)"() -> (w1975:T8)
                n959 = local read "AutoFill Source (P)"() -> (w1976:T8)
                n960 = case shown="\"USB6218AI\"" w1976 {
                  tunnel: [w2012 w2013] -> w1977
                  frame "USB6210", Default {
                    n961 = local read "DataArrayConv (USB6210)"() -> (w2012:dbl[][])
                  }
                  frame "USB6218AI" {
                    n962 = local read "DataArrayConv (USB6218)"() -> (w2013:dbl[][])
                  }
                }
                n963 = case shown="\"USB6210\", Default" w1975 {
                  tunnel: [w2010 w2011] -> w1979
                  frame "USB6210", Default {
                    n964 = local read "DataArrayConv (USB6210)"() -> (w2010:dbl[][])
                  }
                  frame "USB6218AI" {
                    n965 = local read "DataArrayConv (USB6218)"() -> (w2011:dbl[][])
                  }
                }
                n966 = local read "Pstd"() -> (→"Pstd history":dbl)
                n967 = local read "Lstd"() -> (→"Lstd history":dbl)
                n968 = local read "Target Index (L)"() -> (w1980:i32)
                n969 = local read "Pav (Pa)"() -> (→"Pav history":dbl)
                n970 = local read "Lav (%)"() -> (→"Lav history":dbl)
                n971 = Index Array(array=w1979, index (col)=w1980) -> (element=w1978:dbl[])  [unwired: 1 in]
                n972 = local read "Target Index (P)"() -> (w2009:i32)
                n973 = Unbundle By Name(w2008) -> ("TimeArray"=w2007:timestamp[])
                n974 = Index Array(array=w1977, index (col)=w2009) -> (element=w1996:dbl[])  [unwired: 1 in]
                n975 = Delete From Array(array=w1996, length=w1981) -> (deleted portion=w2004:dbl[])  [unwired: 1 in, 1 out]
                n976 = Delete From Array(array=w1978, length=w1981) -> (deleted portion=w1991:dbl[])  [unwired: 1 in, 1 out]
                n977 = call "MovingAverage.vi"("Moving Average interval"=w1994, "Input Array"=w1978) -> ("M.A. Array"=w1993:dbl[])  [unwired: 9 in]
                n978 = call "MovingAverage.vi"("Moving Average interval"=w1994, "Input Array"=w1996) -> ("M.A. Array"=w1995:dbl[])  [unwired: 9 in]
                n979 = Delete From Array(array=w1995, length=w1981) -> (deleted portion=w2005:dbl[])  [unwired: 1 in, 1 out]
                n980 = Delete From Array(array=w1995, length=w1981) -> (deleted portion=w2001:dbl[])  [unwired: 1 in, 1 out]
                "Last N M.A. Pressures" <- w2001
                n981 = Delete From Array(array=w1993, length=w1981) -> (deleted portion=w1986:dbl[])  [unwired: 1 in, 1 out]
                "Last N M.A. Levels" <- w1986
                n982 = Delete From Array(array=w2007, length=w1981) -> (deleted portion=w1988:timestamp[])  [unwired: 1 in, 1 out]
                n983 = Bundle("TimeArray"=w1988, "DataArrayConv (USB6218)"=w2004) -> (w2003:T33)  [unwired: 1 in]
                n984 = Bundle("TimeArray"=w1988, "M.A. Array"=w2005) -> (w2006:T34)  [unwired: 1 in]
                n985 = Bundle("TimeArray"=w1988, "DataArrayConv (USB6218)"=w1991) -> (w1990:T33)  [unwired: 1 in]
                n986 = Bundle("TimeArray"=w1988, "M.A. Array"=w1986) -> (w1987:T34)  [unwired: 1 in]
                n987 = Array Size(array=w2001) -> (size(s)=w2000:i32)
                n988 = Greater Or Equal?(x=w2000, y=w1992) -> (x >= y?=w1999:bool)
                n989 = Build Array(w2003, w2006) -> (→"Dewar Pressure":T35)
                n990 = Build Array(w1990, w1987) -> (→"He Level":T35)
                n991 = case shown="True" w1999 {
                  tunnel: [w2117 w2122] -> w1985
                  tunnel: w2001 -> [_ w2123]
                  tunnel: w1986 -> [_ w2120]
                  tunnel: [w2117 w2118] -> w1984
                  frame False {
                    w2117 = nan ("mean")
                  }
                  frame True {
                    n992 = call <vilib>:"Std Deviation and Variance.vi"("X"=w2123) -> ("mean"=w2122:dbl, "standard deviation"=w2121:dbl)  [unwired: 1 in, 1 out]
                    n993 = call <vilib>:"Std Deviation and Variance.vi"("X"=w2120) -> ("mean"=w2118:dbl, "standard deviation"=w2119:dbl)  [unwired: 1 in, 1 out]
                    n994 = local write "Pstd"(w2121) -> ()
                    n995 = local write "Lstd"(w2119) -> ()
                    n996 = local write "Pav (Pa)"(w2122) -> ()
                    n997 = local write "Lav (%)"(w2118) -> ()
                  }
                }
                n998 = flat-sequence {
                  tunnel: w1985 -> [w2014]
                  tunnel: w1984 -> [w2015]
                  frame #0 {
                    n999 = flat-sequence {
                      tunnel: w2015 -> [w2017]
                      tunnel: w2014 -> [w2016]
                      tunnel: w2014 -> [w2085]
                      frame #0 {
                        n1000 = stacked-sequence {
                          tunnel: w2017 -> [w2024 w2028 _ _ _ _]
                          tunnel: w2016 -> [_ _ w2042 w2051 w2060 w2069]
                          frame #0 {
                            n1001 = local read "L_low (%)"() -> (w2023:dbl)
                            n1002 = local read "Fill state"() -> (w2021:bool)
                            n1003 = Less?(x=w2024, y=w2023) -> (x < y?=w2020:bool)
                            n1004 = Equal?(x=w2021, y=FALSE) -> (x = y?=w2019:bool)
                            n1005 = And(x=w2020, y=w2019) -> (x .and. y?=w2018:bool)
                            n1006 = case shown="False" w2018 {
                              frame False {
                              }
                              frame True {
                                w2026 = TRUE ("Value (Signaling)")
                                n1007 = property on="Fill state" class="Bool (strict)"("Val(Sgnl)"=w2026) -> ()  [unwired: 2 in, 2 out]
                                n1008 = Not(x=w2026) -> (.not. x?=w2025:bool)
                                n1009 = property on="Fill (false)" class="Bool (strict)"("Val(Sgnl)"=w2025) -> ()  [unwired: 2 in, 2 out]
                              }
                            }
                          }
                          frame #1 {
                            n1010 = local read "L_high (%)"() -> (w2029:dbl)
                            n1011 = local read "Fill state"() -> (w2032:bool)
                            n1012 = Greater?(x=w2028, y=w2029) -> (0:w2027:bool)
                            n1013 = Equal?(x=w2032, y=TRUE) -> (x = y?=w2031:bool)
                            n1014 = And(x=w2027, y=w2031) -> (x .and. y?=w2030:bool)
                            n1015 = case shown="True" w2030 {
                              frame False {
                              }
                              frame True {
                                w2034 = FALSE ("Value (Signaling)")
                                n1016 = property on="Fill state" class="Bool (strict)"("Val(Sgnl)"=w2034) -> ()  [unwired: 2 in, 2 out]
                                n1017 = Not(x=w2034) -> (.not. x?=w2035:bool)
                                n1018 = property on="Fill (false)" class="Bool (strict)"("Val(Sgnl)"=w2035) -> ()  [unwired: 2 in, 2 out]
                              }
                            }
                          }
                          frame #2 {
                            n1019 = local read "P_1_low (Pa)"() -> (w2041:dbl)
                            n1020 = property on="state 1" class="Bool (strict)"() -> ("Value"=w2039:bool)  [unwired: 2 in, 2 out]
                            n1021 = Less?(x=w2042, y=w2041) -> (x < y?=w2038:bool)
                            n1022 = Equal?(x=w2039, y=FALSE) -> (x = y?=w2037:bool)
                            n1023 = And(x=w2037, y=w2038) -> (x .and. y?=w2036:bool)
                            n1024 = case shown="True" w2036 {
                              frame False {
                              }
                              frame True {
                                w2044 = TRUE ("Value (Signaling)")
                                n1025 = property on="state 1" class="Bool (strict)"("Val(Sgnl)"=w2044) -> ()  [unwired: 2 in, 2 out]
                                n1026 = Not(x=w2044) -> (.not. x?=w2043:bool)
                                n1027 = property on="state 1 (false)" class="Bool (strict)"("Val(Sgnl)"=w2043) -> ()  [unwired: 2 in, 2 out]
                              }
                            }
                          }
                          frame #3 {
                            n1028 = local read "P_1_high (Pa)"() -> (w2050:dbl)
                            n1029 = property on="state 1" class="Bool (strict)"() -> ("Value"=w2048:bool)  [unwired: 2 in, 2 out]
                            n1030 = Greater?(x=w2051, y=w2050) -> (0:w2047:bool)
                            n1031 = Equal?(x=w2048, y=TRUE) -> (x = y?=w2046:bool)
                            n1032 = And(x=w2046, y=w2047) -> (x .and. y?=w2045:bool)
                            n1033 = case shown="True" w2045 {
                              frame False {
                              }
                              frame True {
                                w2053 = FALSE ("Value (Signaling)")
                                n1034 = property on="state 1" class="Bool (strict)"("Val(Sgnl)"=w2053) -> ()  [unwired: 2 in, 2 out]
                                n1035 = Not(x=w2053) -> (.not. x?=w2052:bool)
                                n1036 = property on="state 1 (false)" class="Bool (strict)"("Val(Sgnl)"=w2052) -> ()  [unwired: 2 in, 2 out]
                              }
                            }
                          }
                          frame #4 {
                            n1037 = local read "P_2_low (Pa)"() -> (w2059:dbl)
                            n1038 = property on="state 2" class="Bool (strict)"() -> ("Value"=w2054:bool)  [unwired: 2 in, 2 out]
                            n1039 = Less?(x=w2060, y=w2059) -> (x < y?=w2057:bool)
                            n1040 = Equal?(x=w2054, y=FALSE) -> (x = y?=w2056:bool)
                            n1041 = And(x=w2056, y=w2057) -> (x .and. y?=w2055:bool)
                            n1042 = case shown="True" w2055 {
                              frame False {
                              }
                              frame True {
                                w2061 = TRUE ("Value (Signaling)")
                                n1043 = property on="state 2" class="Bool (strict)"("Val(Sgnl)"=w2061) -> ()  [unwired: 2 in, 2 out]
                                n1044 = Not(x=w2061) -> (.not. x?=w2062:bool)
                                n1045 = property on="state 2 (false)" class="Bool (strict)"("Val(Sgnl)"=w2062) -> ()  [unwired: 2 in, 2 out]
                              }
                            }
                          }
                          frame #5 {
                            n1046 = local read "P_2_high (Pa)"() -> (w2068:dbl)
                            n1047 = property on="state 2" class="Bool (strict)"() -> ("Value"=w2063:bool)  [unwired: 2 in, 2 out]
                            n1048 = Greater?(x=w2069, y=w2068) -> (0:w2066:bool)
                            n1049 = Equal?(x=w2063, y=TRUE) -> (x = y?=w2065:bool)
                            n1050 = And(x=w2065, y=w2066) -> (x .and. y?=w2064:bool)
                            n1051 = case shown="True" w2064 {
                              frame False {
                              }
                              frame True {
                                w2070 = FALSE ("Value (Signaling)")
                                n1052 = property on="state 2" class="Bool (strict)"("Val(Sgnl)"=w2070) -> ()  [unwired: 2 in, 2 out]
                                n1053 = Not(x=w2070) -> (.not. x?=w2071:bool)
                                n1054 = property on="state 2 (false)" class="Bool (strict)"("Val(Sgnl)"=w2071) -> ()  [unwired: 2 in, 2 out]
                              }
                            }
                          }
                        }
                      }
                      frame #1 {
                        n1055 = property on="Fill state" class="Bool (strict)"() -> ("Value"=w2072:bool)  [unwired: 2 in, 2 out]
                        n1056 = case shown="True" w2072 {
                          frame False {
                            n1057 = property on="V1 (N.O.)" class="Bool (strict)"("Val(Sgnl)"=TRUE ("V1 (N.O.)")) -> ()  [unwired: 2 in, 2 out]
                            n1058 = property on="V2 (N.C.)" class="Bool (strict)"("Val(Sgnl)"=FALSE ("Value (Signaling)")) -> ()  [unwired: 2 in, 2 out]
                          }
                          frame True {
                            n1059 = property on="state 1" class="Bool (strict)"() -> ("Value"=w2076:bool)  [unwired: 2 in, 2 out]
                            n1060 = property on="state 2" class="Bool (strict)"() -> ("Value"=w2075:bool)  [unwired: 2 in, 2 out]
                            n1061 = case shown="True" w2076 {
                              frame False {
                                n1062 = property on="V1 (N.O.)" class="Bool (strict)"("Val(Sgnl)"=TRUE ("Value (Signaling)")) -> ()  [unwired: 2 in, 2 out]
                                n1063 = local write "Status V1 CTRL"(enum16{"Pressurize", "Release"}."Release" ("Status V1 CTRL")) -> ()
                              }
                              frame True {
                                n1064 = property on="V1 (N.O.)" class="Bool (strict)"("Val(Sgnl)"=FALSE ("V1 (N.O.)")) -> ()  [unwired: 2 in, 2 out]
                                n1065 = local write "Status V1 CTRL"(enum16{"Pressurize", "Release"}."Pressurize" ("Status V1 CTRL")) -> ()
                              }
                            }
                            n1066 = case shown="True" w2075 {
                              frame False {
                                n1067 = property on="V2 (N.C.)" class="Bool (strict)"("Val(Sgnl)"=FALSE ("Value (Signaling)")) -> ()  [unwired: 2 in, 2 out]
                                n1068 = local write "Status V2 CTRL"(enum16{"Pressurize", "Release"}."Release" ("Status V2 CTRL")) -> ()
                              }
                              frame True {
                                n1069 = property on="V2 (N.C.)" class="Bool (strict)"("Val(Sgnl)"=TRUE ("Value (Signaling)")) -> ()  [unwired: 2 in, 2 out]
                                n1070 = local write "Status V2 CTRL"(enum16{"Pressurize", "Release"}."Pressurize" ("Status V2 CTRL")) -> ()
                              }
                            }
                          }
                        }
                      }
                      frame #2 {
                        n1071 = Greater?(x=w2085, y="P_safelimit_high (Pa)") -> (0:w2087:bool)
                        n1072 = Less?(x=w2085, y="P_safelimit_low (Pa)") -> (x < y?=w2089:bool)
                        n1073 = Or(x=w2087, y=w2089) -> (x .or. y?=w2090:bool)
                        n1074 = case shown="False" w2090 {
                          frame False {
                          }
                          frame True {
                            w2091 = FALSE ("Value (Signaling)")
                            w2093 = FALSE ("Value (Signaling)")
                            n1075 = property on="V2 (N.C.)" class="Bool (strict)"("Val(Sgnl)"=FALSE ("V1 (N.O.)")) -> ()  [unwired: 2 in, 2 out]
                            n1076 = property on="state 1" class="Bool (strict)"("Val(Sgnl)"=w2091) -> ()  [unwired: 2 in, 2 out]
                            n1077 = property on="V1 (N.O.)" class="Bool (strict)"("Val(Sgnl)"=TRUE ("V1 (N.O.)")) -> ()  [unwired: 2 in, 2 out]
                            n1078 = property on="state 2" class="Bool (strict)"("Val(Sgnl)"=w2093) -> ()  [unwired: 2 in, 2 out]
                            n1079 = Not(x=w2091) -> (.not. x?=w2092:bool)
                            n1080 = Not(x=w2093) -> (.not. x?=w2094:bool)
                            n1081 = property on="state 1 (false)" class="Bool (strict)"("Val(Sgnl)"=w2092) -> ()  [unwired: 2 in, 2 out]
                            n1082 = property on="state 2 (false)" class="Bool (strict)"("Val(Sgnl)"=w2094) -> ()  [unwired: 2 in, 2 out]
                          }
                        }
                      }
                    }
                  }
                  frame #1 {
                    n1083 = property on="V2 (N.C.)" class="Bool (strict)"() -> ("Value"=w2104:bool)  [unwired: 2 in, 2 out]
                    n1084 = property on="V1 (N.O.)" class="Bool (strict)"() -> ("Value"=w2115:bool)  [unwired: 2 in, 2 out]
                    n1085 = local read "P_1_high (Pa)"() -> (w2109:dbl)
                    n1086 = local read "P_2_high (Pa)"() -> (w2107:dbl)
                    n1087 = local read "P_1_low (Pa)"() -> (w2110:dbl)
                    n1088 = local read "P_2_low (Pa)"() -> (w2108:dbl)
                    n1089 = local read "L_high (%)"() -> (w2105:dbl)
                    n1090 = local read "L_low (%)"() -> (w2106:dbl)
                    n1091 = local read "Pav (Pa)"() -> (w2098:dbl)
                    n1092 = local read "Lav (%)"() -> (w2097:dbl)
                    n1093 = Boolean To (0,1)(Boolean=w2104) -> (0, 1=w2103:i16)
                    n1094 = Boolean To (0,1)(Boolean=w2115) -> (0, 1=w2116:i16)
                    n1095 = local read "File Refn DewarCTRL"() -> (w2111:refnum<file>)
                    n1096 = local read "Cycle #"() -> (w2114:u32)
                    n1097 = Build Array(w2098, w2097, w2110, w2109, w2108, w2107, w2106, w2105, w2116, w2103) -> (w2102:dbl[])
                    n1098 = Get Date/Time In Seconds() -> (seconds since 1Jan1904=w2112:timestamp)
                    n1099 = call "FileWrite.vi"("DataArray"=w2102, "Time Stamp"=w2112, "Error In"=errorcluster {"status"=FALSE, "code"=0, "source"=""}, "FileFormat"=string[] ["%4.5e", "%4.2f", "%4.4e", "%4.4e", "%4.4e", "%4.4e", "%4.4e", "%d", "%d"] ("Array"), "Index"=w2114, "refnum in"=w2111) -> ("Error Out"=→"Error Out (Dewar CTRL":errorcluster, "Byte Stream File Refnum"=w2101:refnum<file>)  [unwired: 4 in]
                    n1100 = local write "File Refn DewarCTRL"(w2101) -> ()
                  }
                }
              }
            }
          }
          frame True {
            n1101 = flat-sequence {
              frame #0 {
                w2177 = FALSE ("V1 (N.O.)")
                n1102 = local write "V1 (N.O.)"(TRUE ("V1 (N.O.)")) -> ()
                n1103 = local write "V2 (N.C.)"(FALSE ("V1 (N.O.)")) -> ()
                n1104 = local write "state 2"(w2177) -> ()
                n1105 = local write "state 1"(w2177) -> ()
                n1106 = local write "Fill state"(w2177) -> ()
                n1107 = Not(x=w2177) -> (.not. x?=w2179:bool)
                n1108 = Not(x=w2177) -> (.not. x?=w2178:bool)
                n1109 = local write "state 1 (false)"(w2178) -> ()
                n1110 = local write "state 2 (false)"(w2178) -> ()
                n1111 = local write "Fill (false)"(w2179) -> ()
              }
            }
            n1112 = local read "RUN Identifier"() -> (w2126:string)
            n1113 = Concatenate Strings(w2126, "_DO" ("new task name")) -> (w2169:string)
            n1114 = Concatenate Strings(w2126, "_") -> (w2137:string)
            n1115 = Concatenate Strings(w2137, "DEWAR.csv" ("string")) -> (w2147:string)
            n1116 = Concatenate Strings(w2137, "USB_DOUT.csv" ("string")) -> (w2149:string)
            n1117 = Build Path(base path=w2134, name or relative path=w2147) -> (appended path=w2146:path)
            n1118 = Build Path(base path=w2134, name or relative path=w2149) -> (appended path=w2160:path)
            n1119 = Open/Create/Replace File(file path (use dialog)=w2160, error in=w2155, operation (0:open)=T25."open or create") -> (refnum out=w2158:refnum<file>, error out=w2154:errorcluster)  [unwired: 3 in, 1 out]
            n1120 = call "FileIntialize.vi"("Error In"=w2154, "Labels"="DOUT6218 Labels", "refnum in"=w2158) -> ("Error Out"=w2143:errorcluster, "File Refnum"=→"File Refn USB DO":refnum<file>)  [unwired: 7 in]
            n1121 = Open/Create/Replace File(file path (use dialog)=w2146, error in=w2143, operation (0:open)=T25."open or create") -> (refnum out=w2152:refnum<file>, error out=w2153:errorcluster)  [unwired: 3 in, 1 out]
            n1122 = Concatenate Strings(w2137, "AZDAX.csv" ("string")) -> (w2135:string)
            n1123 = call "FileIntialize.vi"("Error In"=w2153, "Labels"=string[] ["P_av", "L_av", "P_1_low", "P_1_high", "P_2_low", "P_2_high", "L_low", "L_high", "V1(NO)", "V2(NC)"], "refnum in"=w2152) -> ("Error Out"=w2129:errorcluster, "File Refnum"=→"File Refn DewarCTRL":refnum<file>)  [unwired: 7 in]
            n1124 = Build Path(base path=w2134, name or relative path=w2135) -> (appended path=w2131:path)
            n1125 = Array Size(array="DOUT Physical CH") -> (size(s)=w2124:i32)
            n1126 = Open/Create/Replace File(file path (use dialog)=w2131, operation (0:open)=T25."open or create") -> (refnum out=w2132:refnum<file>)  [unwired: 4 in, 2 out]
            n1127 = call "FileIntialize.vi"("Error In"=w2129, "Labels"=string[] ["AZDAX"] ("string"), "refnum in"=w2132) -> ("Error Out"=w2128:errorcluster, "File Refnum"=→"File ref AZD-AX status":refnum<file>)  [unwired: 7 in]
            n1128 = call <vilib>:"DAQmx Create Task.vi"("new task name"=w2169, "auto cleanup"=FALSE, "error in"=w2128) -> ("task out"=w2141:refnum<k21>, "error out"=w2142:errorcluster)  [unwired: 11 in]
            n1129 = for {
              N: w2124 -> [_]
              tunnel: "DOUT Physical CH" -> [w2174] mode=indexing
              shift-right: [w2172] -> w2139
              shift-left: w2141 -> [w2173]
              tunnel: [FALSE ("auto cleanup")] -> w2140 mode=indexing
              shift-right: [w2170] -> w2138
              shift-left: w2142 -> [w2176]
              w2175 = 1 items=["one channel for each line", "one channel for all lines"] ("line grouping")
              n1130 = call-poly <vilib>:"DAQmx Create Virtual Channel.vi"("task in"=w2173, "lines"=w2174, "line grouping"=w2175, "error in"=w2176) -> ("task out"=w2172:refnum<k21>, "error out"=w2170:errorcluster)  [unwired: 10 in]
            }
            n1131 = call <vilib>:"DAQmx Start Task.vi"("task/channels in"=w2139, "error in"=w2138) -> ("task out"=w2165:refnum<k21>, "error out"=w2163:errorcluster)  [unwired: 12 in]
            n1132 = call <vilib>:"DAQmx Write (Digital 1D Bool NChan 1Samp 1Line).vi"("task/channels in"=w2165, "data"=w2140, "timeout"=10.0, "error in"=w2163) -> ("task out"=→"DOUT task out":refnum<k21>, "error out"=w2162:errorcluster)  [unwired: 9 in, 1 out]
          }
        }
      }
    }
    "error out (USB6210/6218 DOUT)" <- w1193
    n1133 = Build Array (concatenate)(w1158, w1159) -> (w1156:dbl[])
    n1134 = Build Array (concatenate)(w1161, w1160) -> (w1157:string[])
    n1135 = flat-sequence {
      tunnel: w1240 -> [w1829]
      tunnel: [w1824] -> w1228
      tunnel: [w1822] -> w1226
      tunnel: [w1821] -> w1223
      tunnel: [w1820] -> w1221
      tunnel: w1192 -> [w1815]
      frame #0 {
        w1823 = T26 [] ("appended array")
        n1136 = Unbundle By Name(w1815) -> ("TimeArray"=w1832:timestamp[], "DataArrayConv"=w1827:dbl[][], "LDArray"=w1826:dbl[])
        n1137 = Unbundle By Name(w1829) -> ("ReadLeakDet?"=w1828:bool, "LabelLD"=w1831:string, "Labels"=w1825:string[])  [unwired: 1 out]
        n1138 = case shown="True" w1828 {
          tunnel: w1831 -> [_ w1840]
          tunnel: w1827 -> [w1834 w1839]
          tunnel: w1826 -> [_ w1838]
          tunnel: [w1834 w1837] -> w1814
          tunnel: w1825 -> [w1833 w1836]
          tunnel: [w1833 w1835] -> w1817
          frame False {
          }
          frame True {
            n1139 = Build Array (concatenate)(w1839, w1838) -> (w1837:dbl[][])
            n1140 = Build Array (concatenate)(w1836, w1840) -> (w1835:string[])
          }
        }
        "All Labels (USB6210)" <- w1817
        "DataArrayConv (USB6210)" <- w1814
        n1141 = control-ref of="Plot selecter (USB6210)\n    1      2     3     4"() -> (w1816:refnum<vi>)
        n1142 = local read "Plot selecter (USB6210)\n    1      2     3     4"() -> (w1819:bool[][])
        n1143 = Array Size(array=w1817) -> (size(s)=w1830:i32)
        n1144 = Array Size(array=w1817) -> (size(s)=w1818:i32)
        n1145 = Array Size(array=w1814) -> (size(s)=→"Data Array sizes (6210)":i32[])
        n1146 = property on="Property Node" class="Arr (strict)"(reference=w1816, "Number of Rows"=w1818) -> ()  [unwired: 1 in, 2 out]
        n1147 = for {
          N: w1830 -> [_]
          tunnel: w1814 -> [w1861]
          tunnel: w1832 -> [w1862]
          shift-right: [w1857] -> w1822
          shift-left: w1823 -> [w1860]
          shift-right: [w1855] -> w1820
          shift-left: w1823 -> [w1858]
          shift-right: [w1856] -> w1824
          shift-left: w1823 -> [w1854]
          shift-right: [w1853] -> w1821
          shift-left: w1823 -> [w1852]
          tunnel: w1819 -> [w1851]
          i -> [w1846]
          n1148 = Index Array(array=w1861, index (col)=w1846) -> (element=w1841:dbl[])  [unwired: 1 in]
          n1149 = Index Array(array=w1851, index (row) #1=w1846, index (col) #1=0 ("index (row)"), index (row) #2=w1846, index (col) #2=1 ("index (row)"), index (row) #3=w1846, index (col) #3=2 ("index (row)"), index (row) #4=w1846, index (col) #4=3 ("index (row)")) -> (element #1=w1845:bool, element #2=w1844:bool, element #3=w1843:bool, element #4=w1842:bool)
          n1150 = Bundle("TimeArray"=w1862, "DataArrayConv"=w1841) -> (w1859:T32)  [unwired: 1 in]
          n1151 = stacked-sequence {
            tunnel: w1845 -> [w1866 _ _ _]
            tunnel: w1860 -> [_ w1874 _ _]
            tunnel: w1843 -> [_ _ w1882 _]
            tunnel: w1859 -> [w1863 w1872 w1881 w1887]
            tunnel: w1842 -> [_ _ _ w1890]
            tunnel: w1858 -> [_ _ _ w1889]
            tunnel: [_ _ _ w1888] -> w1855
            tunnel: [_ w1873 _ _] -> w1857
            tunnel: [w1865 _ _ _] -> w1856
            tunnel: w1854 -> [w1864 _ _ _]
            tunnel: [_ _ w1880 _] -> w1853
            tunnel: w1852 -> [_ _ w1879 _]
            tunnel: w1844 -> [_ w1871 _ _]
            frame #0 {
              n1152 = case shown="True" w1866 {
                tunnel: [w1867 w1870] -> w1865
                tunnel: w1863 -> [_ w1869]
                tunnel: w1864 -> [w1867 w1868]
                frame False {
                }
                frame True {
                  n1153 = Build Array (concatenate)(w1868, w1869) -> (w1870:T26)
                }
              }
            }
            frame #1 {
              n1154 = case shown="True" w1871 {
                tunnel: w1874 -> [w1875 w1878]
                tunnel: [w1875 w1877] -> w1873
                tunnel: w1872 -> [_ w1876]
                frame False {
                }
                frame True {
                  n1155 = Build Array (concatenate)(w1878, w1876) -> (w1877:T26)
                }
              }
            }
            frame #2 {
              n1156 = case shown="True" w1882 {
                tunnel: [w1883 w1886] -> w1880
                tunnel: w1881 -> [_ w1885]
                tunnel: w1879 -> [w1883 w1884]
                frame False {
                }
                frame True {
                  n1157 = Build Array (concatenate)(w1884, w1885) -> (w1886:T26)
                }
              }
            }
            frame #3 {
              n1158 = case shown="True" w1890 {
                tunnel: [w1891 w1894] -> w1888
                tunnel: w1887 -> [_ w1893]
                tunnel: w1889 -> [w1891 w1892]
                frame False {
                }
                frame True {
                  n1159 = Build Array (concatenate)(w1892, w1893) -> (w1894:T26)
                }
              }
            }
          }
        }
      }
    }
    n1160 = local read "Plot selecter LSI218(2)\n    1      2     3     4"() -> (w1215:bool[][])
    n1161 = local read "Plot selecter LSI218(1)\n    1      2     3     4"() -> (w1216:bool[][])
    n1162 = for {
      N: 48 -> [_]
      tunnel: w1231 -> [w2281]
      tunnel: w1230 -> [w2278]
      tunnel: w1216 -> [w2262]
      tunnel: w1215 -> [w2263]
      shift-right: [w2279] -> w1229
      shift-left: w1227 -> [w2280]
      shift-right: [w2274] -> w1224
      shift-left: w1227 -> [w2275]
      shift-right: [w2273] -> w1222
      shift-left: w1227 -> [w2272]
      shift-right: [w2271] -> w1220
      shift-left: w1227 -> [w2270]
      i -> [w2268]
      n1163 = Index Array(array=w2278, index (col)=w2268) -> (element=w2277:dbl[])  [unwired: 1 in]
      n1164 = Less?(x=w2268, y=24) -> (x < y?=w2269:bool)
      n1165 = case shown="True" w2269 {
        tunnel: [w2286 w2304] -> w2267
        tunnel: [w2285 w2303] -> w2266
        tunnel: [w2284 w2301] -> w2265
        tunnel: [w2283 w2300] -> w2264
        tunnel: w2262 -> [_ w2299]
        tunnel: w2263 -> [w2293 _]
        tunnel: w2268 -> [w2288 w2296]
        frame False {
          n1166 = Subtract(x=w2288, y=24) -> (x-y=w2292:i32)
          n1167 = Index Array(array=w2293, index (row) #1=w2292, index (col) #1=0 ("index (row)"), index (row) #2=w2292, index (col) #2=1 ("index (row)"), index (row) #3=w2292, index (col) #3=2 ("index (row)"), index (row) #4=w2292, index (col) #4=3 ("index (row)")) -> (element #1=w2286:bool, element #2=w2285:bool, element #3=w2284:bool, element #4=w2283:bool)
        }
        frame True {
          n1168 = Index Array(array=w2299, index (row) #1=w2296, index (col) #1=0 ("index (row)"), index (row) #2=w2296, index (col) #2=1 ("index (row)"), index (row) #3=w2296, index (col) #3=2 ("index (row)"), index (row) #4=w2296, index (col) #4=3 ("index (row)")) -> (element #1=w2304:bool, element #2=w2303:bool, element #3=w2301:bool, element #4=w2300:bool)
        }
      }
      n1169 = Bundle("TimeArray"=w2281, "DataArray"=w2277) -> (w2276:T36)  [unwired: 1 in]
      n1170 = stacked-sequence {
        tunnel: w2280 -> [w2308 _ _ _]
        tunnel: [w2307 _ _ _] -> w2279
        tunnel: w2276 -> [w2306 w2316 w2324 w2332]
        tunnel: w2275 -> [_ w2315 _ _]
        tunnel: [_ w2314 _ _] -> w2274
        tunnel: [_ _ w2323 _] -> w2273
        tunnel: w2272 -> [_ _ w2322 _]
        tunnel: [_ _ _ w2331] -> w2271
        tunnel: w2270 -> [_ _ _ w2330]
        tunnel: w2267 -> [w2305 _ _ _]
        tunnel: w2266 -> [_ w2313 _ _]
        tunnel: w2265 -> [_ _ w2321 _]
        tunnel: w2264 -> [_ _ _ w2329]
        frame #0 {
          n1171 = case shown="False" w2305 {
            tunnel: w2306 -> [_ w2310]
            tunnel: w2308 -> [w2309 w2312]
            tunnel: [w2309 w2311] -> w2307
            frame False {
            }
            frame True {
              n1172 = Build Array (concatenate)(w2312, w2310) -> (w2311:T4)
            }
          }
        }
        frame #1 {
          n1173 = case shown="True" w2313 {
            tunnel: [w2317 w2320] -> w2314
            tunnel: w2316 -> [_ w2319]
            tunnel: w2315 -> [w2317 w2318]
            frame False {
            }
            frame True {
              n1174 = Build Array (concatenate)(w2318, w2319) -> (w2320:T4)
            }
          }
        }
        frame #2 {
          n1175 = case shown="True" w2321 {
            tunnel: [w2325 w2328] -> w2323
            tunnel: w2324 -> [_ w2327]
            tunnel: w2322 -> [w2325 w2326]
            frame False {
            }
            frame True {
              n1176 = Build Array (concatenate)(w2326, w2327) -> (w2328:T4)
            }
          }
        }
        frame #3 {
          n1177 = case shown="True" w2329 {
            tunnel: [w2333 w2336] -> w2331
            tunnel: w2332 -> [_ w2335]
            tunnel: w2330 -> [w2333 w2334]
            frame False {
            }
            frame True {
              n1178 = Build Array (concatenate)(w2334, w2335) -> (w2336:T4)
            }
          }
        }
      }
    }
    n1179 = local read "Labels LSI336"() -> (w1203:string[])
    n1180 = Array Size(array=w1203) -> (size(s)=w1202:i32)
    n1181 = local read "Plot selecter LSI336 \n     1      2     3     4"() -> (w1211:bool[][])
    n1182 = for {
      N: w1202 -> [_]
      tunnel: w1211 -> [w2194]
      shift-right: [w2188] -> w1209
      shift-left: w1210 -> [w2203]
      shift-right: [w2184] -> w1208
      shift-left: w1210 -> [w2201]
      shift-right: [w2185] -> w1207
      shift-left: w1210 -> [w2200]
      shift-right: [w2183] -> w1206
      shift-left: w1210 -> [w2199]
      tunnel: w1172 -> [w2191]
      tunnel: w1174 -> [w2189]
      i -> [w2192]
      n1183 = Index Array(array=w2191, index (col)=w2192) -> (element=w2190:dbl[])  [unwired: 1 in]
      n1184 = Index Array(array=w2194, index (row) #1=w2192, index (col) #1=0 ("index (row)"), index (row) #2=w2192, index (col) #2=1 ("index (row)"), index (row) #3=w2192, index (col) #3=2 ("index (row)"), index (row) #4=w2192, index (col) #4=3 ("index (row)")) -> (element #1=w2193:bool, element #2=w2187:bool, element #3=w2186:bool, element #4=w2182:bool)
      n1185 = Bundle("TimeArray"=w2189, "DataArray"=w2190) -> (w2202:T36)  [unwired: 1 in]
      n1186 = stacked-sequence {
        tunnel: w2203 -> [w2207 _ _ _]
        tunnel: [w2206 _ _ _] -> w2188
        tunnel: w2202 -> [w2205 w2215 w2223 w2231]
        tunnel: w2201 -> [_ w2214 _ _]
        tunnel: [_ w2213 _ _] -> w2184
        tunnel: [_ _ w2222 _] -> w2185
        tunnel: w2200 -> [_ _ w2221 _]
        tunnel: [_ _ _ w2230] -> w2183
        tunnel: w2199 -> [_ _ _ w2229]
        tunnel: w2193 -> [w2204 _ _ _]
        tunnel: w2187 -> [_ w2212 _ _]
        tunnel: w2186 -> [_ _ w2220 _]
        tunnel: w2182 -> [_ _ _ w2228]
        frame #0 {
          n1187 = case shown="False" w2204 {
            tunnel: w2205 -> [_ w2209]
            tunnel: w2207 -> [w2208 w2211]
            tunnel: [w2208 w2210] -> w2206
            frame False {
            }
            frame True {
              n1188 = Build Array (concatenate)(w2211, w2209) -> (w2210:T4)
            }
          }
        }
        frame #1 {
          n1189 = case shown="True" w2212 {
            tunnel: [w2216 w2219] -> w2213
            tunnel: w2215 -> [_ w2217]
            tunnel: w2214 -> [w2216 w2218]
            frame False {
            }
            frame True {
              n1190 = Build Array (concatenate)(w2218, w2217) -> (w2219:T4)
            }
          }
        }
        frame #2 {
          n1191 = case shown="True" w2220 {
            tunnel: [w2224 w2227] -> w2222
            tunnel: w2223 -> [_ w2225]
            tunnel: w2221 -> [w2224 w2226]
            frame False {
            }
            frame True {
              n1192 = Build Array (concatenate)(w2226, w2225) -> (w2227:T4)
            }
          }
        }
        frame #3 {
          n1193 = case shown="True" w2228 {
            tunnel: [w2232 w2235] -> w2230
            tunnel: w2231 -> [_ w2233]
            tunnel: w2229 -> [w2232 w2234]
            frame False {
            }
            frame True {
              n1194 = Build Array (concatenate)(w2234, w2233) -> (w2235:T4)
            }
          }
        }
      }
    }
    n1195 = Array Size(array=w1174) -> (size(s)=→"TimeArray Size (336)":i32)
    n1196 = Array Size(array=w1172) -> (size(s)=→"DataArray size (336)":i32[])
    n1197 = Build Array (concatenate)(w1228, w1229, w1209, w1187, w1132) -> (→"Graph 1":T26)
    n1198 = Build Array (concatenate)(w1226, w1224, w1208, w1186, w1131) -> (→"Graph 2":T26)
    n1199 = Build Array (concatenate)(w1223, w1222, w1207, w1185, w1130) -> (→"Graph 3":T26)
    n1200 = Build Array (concatenate)(w1221, w1220, w1206, w1184, w1129) -> (→"Graph 4":T26)
    n1201 = Send Notification(notification="Stop Button", notifier=w1149, error in (no error)=w1148) -> (notifier out=w1145:refnum<notifier>, error out=w1146:errorcluster)
    "Cycle #" <- w1138
  }
  n1202 = while {
    tunnel: w5 -> [w2425]
    tunnel: w4 -> [w2424]
    stop <- w2426 stop-if-true
    n1203 = flat-sequence {
      frame #0 {
        n1204 = Divide(x="V_sample", y="I_sample") -> (x/y=w2432:dbl)
        "R_sample" <- w2432
        n1205 = Multiply(x="I_sample", y="V_sample") -> (x*y=→"Q_sample":dbl)
        n1206 = Divide(x="Q_input", y=w2432) -> (x/y=w2431:dbl)
        n1207 = Square Root(x=w2431) -> (sqrt(x)=→"V_input":dbl)
      }
    }
    n1208 = Wait (ms)(milliseconds to wait=u32 214) -> ()  [unwired: 1 out]
    n1209 = case shown="True" "START heater cycle" {
      frame False {
      }
      frame True {
        n1210 = flat-sequence {
          frame #0 {
            n1211 = while {
              i -> [w2439]
              stop <- w2437 stop-if-true
              n1212 = flat-sequence {
                frame #0 {
                  n1213 = property on="OUTPUT \nKenwood" class="Bool (strict)"("Val(Sgnl)"=TRUE ("Value (Signaling)")) -> ()  [unwired: 2 in, 2 out]
                  n1214 = property on="Kenwood set V (V)" class="DigNum (strict)"("Val(Sgnl)"="V_peak") -> ()  [unwired: 2 in, 2 out]
                }
                frame #1 {
                  n1215 = Multiply(x="t_on", y=1000.0) -> (x*y=w2445:dbl)
                  n1216 = Wait (ms)(milliseconds to wait=w2445) -> ()  [unwired: 1 out]
                }
                frame #2 {
                  n1217 = property on="OUTPUT \nKenwood" class="Bool (strict)"("Val(Sgnl)"=FALSE ("Value (Signaling)")) -> ()  [unwired: 2 in, 2 out]
                  n1218 = property on="Kenwood set V (V)" class="DigNum (strict)"("Val(Sgnl)"=0.0 ("Value (Signaling)")) -> ()  [unwired: 2 in, 2 out]
                }
                frame #3 {
                  n1219 = Multiply(x="t_off", y=1000.0) -> (x*y=w2452:dbl)
                  n1220 = Wait (ms)(milliseconds to wait=w2452) -> ()  [unwired: 1 out]
                }
              }
              n1221 = case shown="True" "STOP heater cycle" {
                tunnel: [FALSE TRUE] -> w2437
                frame False {
                }
                frame True {
                  n1222 = property on="START heater cycle" class="Bool (strict)"("Val(Sgnl)"=FALSE ("Value (Signaling)")) -> ()  [unwired: 2 in, 2 out]
                }
              }
              "Heat Cycle counter" <- w2439
            }
          }
          frame #1 {
            n1223 = property on="STOP heater cycle" class="Bool (strict)"("Val(Sgnl)"=FALSE ("Value (Signaling)")) -> ()  [unwired: 2 in, 2 out]
          }
        }
      }
    }
    n1224 = case shown="False" "RECORD GRAPH" {
      frame False {
      }
      frame True {
        n1225 = stacked-sequence {
          frame #0 {
            n1226 = Get Date/Time In Seconds() -> (seconds since 1Jan1904=w2471:timestamp)
            n1227 = local read "Base Path"() -> (w2456:path)
            n1228 = local read "RUN Identifier"() -> (w2472:string)
            n1229 = call "LV_UNIXTIME.vi"("current time"=w2471) -> ("date/time string"=w2473:string)  [unwired: 9 in, 1 out]
            n1230 = control-ref of="Graph CHF"() -> (w2462:refnum<vi>)
            n1231 = Concatenate Strings(w2472, "_CHF" ("string"), w2473, "_" ("string"), "CHF Graph Comment") -> (w2458:string)
            n1232 = Concatenate Strings(w2458, ".png" ("string")) -> (w2457:string)
            n1233 = Concatenate Strings(w2458, ".csv" ("string")) -> (w2460:string)
            "CHF file name" <- w2460
            n1234 = Build Path(base path=w2456, name or relative path=w2460) -> (appended path=w2467:path)
            n1235 = invoke class="XYGraph (strict)" method="Get Image"(reference=w2462) -> ("image data"=w2454:T24)  [unwired: 5 in, 5 out]
            n1236 = local read "ƒ¢T_array"() -> (w2464:dbl[])
            n1237 = local read "Q_array"() -> (w2463:dbl[])
            n1238 = Build Path(base path=w2456, name or relative path=w2457) -> (appended path=w2455:path)
            n1239 = Open/Create/Replace File(file path (use dialog)=w2467, operation (0:open)=T25."open or create") -> (refnum out=w2465:refnum<file>)  [unwired: 4 in, 2 out]
            n1240 = for {
              tunnel: w2465 -> [w2477]
              tunnel: w2464 -> [w2475] mode=indexing
              tunnel: w2463 -> [w2474] mode=indexing
              n1241 = Format Into String(format string="%4.4e,%4.4e\\n" ("prompt"), initial string=w2477, w2475, w2474) -> ()  [unwired: 1 in, 2 out]
            }
            n1242 = call <vilib>:"Write PNG File.vi"("image data"=w2454, "path to PNG file"=w2455) -> ()  [unwired: 8 in, 2 out]
          }
          frame #1 {
            n1243 = local write "RECORD GRAPH"(FALSE ("RECORD GRAPH")) -> ()
          }
        }
      }
    }
    n1244 = case shown="False" "START CHF" {
      tunnel: "RecordSettings" -> [_ w2482]
      frame False {
      }
      frame True {
        n1245 = stacked-sequence {
          tunnel: [w2486 _ _] -> _
          tunnel: w2482 -> [w2485 w2559 _]
          frame #0 {
            (unwired) T25."open or create" ("operation (0:open)")
            n1246 = Get Date/Time In Seconds() -> (seconds since 1Jan1904=w2498:timestamp)
            n1247 = for {
              tunnel: [w2546] -> w2484 mode=indexing
              tunnel: w2485 -> [w2545] mode=indexing
              n1248 = Unbundle By Name(w2545) -> ("SourceLabel"=w2546:string)
            }
            "CHF Data Labels" <- w2484
            n1249 = local read "Base Path"() -> (w2493:path)
            n1250 = local read "RUN Identifier"() -> (w2497:string)
            n1251 = call "LV_UNIXTIME.vi"("current time"=w2498) -> ("date/time string"=w2496:string)  [unwired: 9 in, 1 out]
            n1252 = Concatenate Strings(w2497, "_" ("string"), w2496, "_CHFlog.csv" ("string")) -> (w2492:string)
            "CHF log file name" <- w2492
            n1253 = Build Path(base path=w2493, name or relative path=w2492) -> (appended path=w2491:path)
            n1254 = Open/Create/Replace File(file path (use dialog)=w2491, error in=errorcluster {"status"=FALSE, "code"=0, "source"=""}, operation (0:open)=T25."open or create", access (0:read/write)=enum16{"read/write", "read-only", "write-only"}."read/write") -> (refnum out=w2489:refnum<file>, error out=w2488:errorcluster)  [unwired: 2 in, 1 out]
            n1255 = call "FileIntialize.vi"("Error In"=w2488, "Labels"=w2484, "refnum in"=w2489) -> ("File Refnum"=w2486:refnum<file>)  [unwired: 7 in, 1 out]
            "File Refnum (CHF)" <- w2486
            n1256 = local write "CHF measurement counter"(0 ("CHF counter")) -> ()
            n1257 = property on="Kenwood set V (V)" class="DigNum (strict)"("Val(Sgnl)"="V start (V)") -> ()  [unwired: 2 in, 2 out]
            n1258 = stacked-sequence {
              tunnel: w2484 -> [w2502 w2525]
              frame #0 {
                n1259 = Array Size(array=w2502) -> (size(s)=w2510:i32)
                n1260 = control-ref of="Graph CHF log 1"() -> (w2503:refnum<vi>)
                n1261 = property class="XYGraph (strict)"(reference=w2503, error in=errorcluster {"status"=FALSE, "code"=0, "source"=""} ("error in (no error)")) -> (reference out=w2505:refnum<vi>, error out=w2507:errorcluster, "LegNumRows"=w2508:u32)
                n1262 = for {
                  N: w2508 -> [_]
                  shift-right: [w2519] -> w2509
                  shift-left: w2507 -> [w2520]
                  tunnel: w2505 -> [w2518]
                  tunnel: [w2517] -> w2504 mode=indexing
                  i -> [w2522]
                  n1263 = property class="XYGraph (strict)"(reference=w2518, error in=w2520, "Active Plot"=w2522, "Plot.Plot Name"="") -> (reference out=w2517:refnum<vi>, error out=w2519:errorcluster)
                }
                n1264 = for {
                  N: w2510 -> [_]
                  shift-right: [w2514] -> w2501
                  shift-left: w2509 -> [w2515]
                  tunnel: w2504 -> [w2512] mode=indexing
                  tunnel: w2502 -> [w2511] mode=indexing
                  i -> [w2516]
                  n1265 = property class="XYGraph (strict)"(reference=w2512, error in=w2515, "Active Plot"=w2516, "Plot.Plot Name"=w2511, "Plot.Visible?"=TRUE ("Plot.Visible")) -> (error out=w2514:errorcluster)  [unwired: 1 out]
                }
                n1266 = local write "Error out (CHF rec)"(w2501) -> ()
              }
              frame #1 {
                n1267 = Array Size(array=w2525) -> (size(s)=w2532:i32)
                n1268 = control-ref of="Graph CHF log 2"() -> (w2524:refnum<vi>)
                n1269 = property class="XYGraph (strict)"(reference=w2524, error in=errorcluster {"status"=FALSE, "code"=0, "source"=""} ("error in (no error)")) -> (reference out=w2527:refnum<vi>, error out=w2529:errorcluster, "LegNumRows"=w2530:u32)
                n1270 = for {
                  N: w2530 -> [_]
                  shift-right: [w2541] -> w2531
                  shift-left: w2529 -> [w2542]
                  tunnel: w2527 -> [w2540]
                  tunnel: [w2539] -> w2526 mode=indexing
                  i -> [w2544]
                  n1271 = property class="XYGraph (strict)"(reference=w2540, error in=w2542, "Active Plot"=w2544, "Plot.Plot Name"="") -> (reference out=w2539:refnum<vi>, error out=w2541:errorcluster)
                }
                n1272 = for {
                  N: w2532 -> [_]
                  shift-right: [w2536] -> w2523
                  shift-left: w2531 -> [w2537]
                  tunnel: w2526 -> [w2534] mode=indexing
                  tunnel: w2525 -> [w2533] mode=indexing
                  i -> [w2538]
                  n1273 = property class="XYGraph (strict)"(reference=w2534, error in=w2537, "Active Plot"=w2538, "Plot.Plot Name"=w2533, "Plot.Visible?"=TRUE ("Plot.Visible")) -> (error out=w2536:errorcluster)  [unwired: 1 out]
                }
                n1274 = local write "Error out (CHF rec)"(w2523) -> ()
              }
            }
          }
          frame #1 {
            n1275 = local read "V start (V)"() -> (w2558:dbl)
            n1276 = Absolute Value(x="V_end (V)") -> (abs(x)=w2555:dbl)
            n1277 = Absolute Value(x=w2558) -> (abs(x)=w2556:dbl)
            n1278 = Build Array(w2556, w2555) -> (w2554:dbl[])
            n1279 = Array Max & Min(array=w2554) -> (max value=w2553:dbl, min value=w2552:dbl)  [unwired: 2 out]
            n1280 = Subtract(x=w2553, y=w2552) -> (x-y=w2551:dbl)
            n1281 = Quotient & Remainder(x=w2551, y="ƒ¢V / cycle (V)") -> (floor(x/y)=w2549:dbl)  [unwired: 1 out]
            n1282 = for {
              N: w2549 -> [_]
              tunnel: w2559 -> [w2567]
              shift-right: [w2563] -> _
              shift-left: dbl[][] [] -> [w2565]
              shift-right: [w2562] -> _
              shift-left: timestamp[] [] -> [w2564]
              tunnel: "ƒ¢V / cycle (V)" -> [w2561]
              i -> [w2566]
              n1283 = case shown="False" "STOP CHF" {
                tunnel: w2567 -> [w2583 _]
                tunnel: w2566 -> [w2582 _]
                tunnel: w2565 -> [w2581 w2808]
                tunnel: w2564 -> [w2577 w2807]
                tunnel: [w2574 w2808] -> w2563
                tunnel: [w2573 w2807] -> w2562
                tunnel: w2561 -> [w2568 _]
                frame False {
                  n1284 = stacked-sequence {
                    tunnel: w2583 -> [_ _ w2615]
                    tunnel: [_ _ w2606] -> w2572
                    tunnel: w2582 -> [_ _ w2605]
                    tunnel: w2582 -> [w2590 _ _]
                    tunnel: [_ _ w2603] -> w2571
                    tunnel: [_ _ w2602] -> w2576
                    tunnel: [_ _ w2601] -> w2580
                    tunnel: w2581 -> [_ _ w2601]
                    tunnel: [_ _ w2600] -> w2579
                    tunnel: w2577 -> [_ _ w2599]
                    tunnel: [_ _ w2599] -> w2578
                    tunnel: w2568 -> [w2589 _ _]
                    frame #0 {
                      n1285 = property on="CHF measurement counter" class="DigNum (strict)"("Val(Sgnl)"=w2590) -> ()  [unwired: 2 in, 2 out]
                      n1286 = property on="Kenwood set V (V)" class="DigNum (strict)"() -> ("Value"=w2592:dbl)  [unwired: 2 in, 2 out]
                      n1287 = Add(x=w2592, y=w2589) -> (x+y=w2591:dbl)
                      n1288 = property on="Kenwood set V (V)" class="DigNum (strict)"("Val(Sgnl)"=w2591) -> ()  [unwired: 2 in, 2 out]
                    }
                    frame #1 {
                      n1289 = Multiply(x="CHF cycle interval (s) (>1s)", y=1000.0) -> (x*y=w2594:dbl)
                      n1290 = Wait (ms)(milliseconds to wait=w2594) -> ()  [unwired: 1 out]
                    }
                    frame #2 {
                      n1291 = for {
                        tunnel: w2615 -> [w2772] mode=indexing
                        tunnel: [w2770] -> w2602 mode=indexing
                        tunnel: [w2768] -> w2613 mode=indexing
                        n1292 = Unbundle By Name(w2772) -> ("Source"=w2771:T37, "SourceLabel"=w2769:string, "FileFormat"=w2768:string)
                        n1293 = case shown="\"LSI218\"" w2771 {
                          tunnel: [w2773 w2778 w2783 w2789 w2797 w2802] -> w2770
                          tunnel: w2769 -> [w2774 w2780 w2785 w2788 w2798 w2806]
                          frame "USB6210", Default {
                            n1294 = local read "All Labels (USB6210)"() -> (w2776:string[])
                            n1295 = local read "Last Data \n(USB6210)"() -> (w2777:dbl[])
                            n1296 = Search 1D Array(1D array=w2776, element=w2774) -> (index of element=w2775:i32)  [unwired: 1 in]
                            n1297 = Index Array(array=w2777, index=w2775) -> (element=w2773:dbl)
                          }
                          frame "USB6218AI" {
                            n1298 = local read "All Labels (USB6218)"() -> (w2781:string[])
                            n1299 = local read "Last Data \n(USB6218)"() -> (w2782:dbl[])
                            n1300 = Search 1D Array(1D array=w2781, element=w2780) -> (index of element=w2779:i32)  [unwired: 1 in]
                            n1301 = Index Array(array=w2782, index=w2779) -> (element=w2778:dbl)
                          }
                          frame "USB6218AO" {
                            n1302 = local read "USB 6218 AOUT"() -> (w2787:dbl[])
                            n1303 = local read "AOUT Labels"() -> (w2786:string[])
                            n1304 = Search 1D Array(1D array=w2786, element=w2785) -> (index of element=w2784:i32)  [unwired: 1 in]
                            n1305 = Index Array(array=w2787, index=w2784) -> (element=w2783:dbl)
                          }
                          frame "LSI218" {
                            n1306 = local read "Labels LSI218 (1)"() -> (w2792:string[])
                            n1307 = local read "Labels LSI218 (2)"() -> (w2791:string[])
                            n1308 = local read "Last Data \nLSI218 (1)"() -> (w2795:dbl[])
                            n1309 = local read "Last Data \nLSI218 (2)"() -> (w2794:dbl[])
                            n1310 = Build Array (concatenate)(w2792, w2791) -> (w2790:string[])
                            n1311 = Build Array (concatenate)(w2795, w2794) -> (w2793:dbl[])
                            n1312 = Search 1D Array(1D array=w2790, element=w2788) -> (index of element=w2796:i32)  [unwired: 1 in]
                            n1313 = Index Array(array=w2793, index=w2796) -> (element=w2789:dbl)
                          }
                          frame "LSI336" {
                            n1314 = local read "Last Data \nLSI336"() -> (w2800:dbl[])
                            n1315 = local read "Labels LSI336"() -> (w2801:string[])
                            n1316 = Search 1D Array(1D array=w2801, element=w2798) -> (index of element=w2799:i32)  [unwired: 1 in]
                            n1317 = Index Array(array=w2800, index=w2799) -> (element=w2797:dbl)
                          }
                          frame "DMMs" {
                            n1318 = local read "DMM LastMeasurements"() -> (w2803:dbl[])
                            n1319 = local read "DMMsLabels"() -> (w2805:string[])
                            n1320 = Search 1D Array(1D array=w2805, element=w2806) -> (index of element=w2804:i32)  [unwired: 1 in]
                            n1321 = Index Array(array=w2803, index=w2804) -> (element=w2802:dbl)
                          }
                        }
                      }
                      "CHF last data" <- w2602
                      n1322 = stacked-sequence {
                        tunnel: [w2616 _ _ _] -> w2611
                        tunnel: [_ w2654 _ _] -> w2610
                        tunnel: [_ _ _ w2730] -> w2609
                        tunnel: [_ _ w2692 _] -> w2608
                        frame #0 {
                          n1323 = Unbundle By Name("Data I") -> ("Source"=w2618:T37, "SourceLabel"=w2617:string)
                          n1324 = case shown="\"DMMs\"" w2618 {
                            tunnel: w2617 -> [w2621 w2626 w2631 w2636 w2645 w2650]
                            tunnel: [w2620 w2625 w2630 w2635 w2644 w2649] -> w2616
                            frame "USB6210", Default {
                              n1325 = local read "All Labels (USB6210)"() -> (w2623:string[])
                              n1326 = local read "Last Data \n(USB6210)"() -> (w2622:dbl[])
                              n1327 = Search 1D Array(1D array=w2623, element=w2621) -> (index of element=w2624:i32)  [unwired: 1 in]
                              n1328 = Index Array(array=w2622, index=w2624) -> (element=w2620:dbl)
                            }
                            frame "USB6218AI" {
                              n1329 = local read "All Labels (USB6218)"() -> (w2628:string[])
                              n1330 = local read "Last Data \n(USB6218)"() -> (w2627:dbl[])
                              n1331 = Search 1D Array(1D array=w2628, element=w2626) -> (index of element=w2629:i32)  [unwired: 1 in]
                              n1332 = Index Array(array=w2627, index=w2629) -> (element=w2625:dbl)
                            }
                            frame "USB6218AO" {
                              n1333 = local read "USB 6218 AOUT"() -> (w2632:dbl[])
                              n1334 = local read "AOUT Labels"() -> (w2633:string[])
                              n1335 = Search 1D Array(1D array=w2633, element=w2631) -> (index of element=w2634:i32)  [unwired: 1 in]
                              n1336 = Index Array(array=w2632, index=w2634) -> (element=w2630:dbl)
                            }
                            frame "LSI218" {
                              n1337 = local read "Labels LSI218 (1)"() -> (w2641:string[])
                              n1338 = local read "Labels LSI218 (2)"() -> (w2642:string[])
                              n1339 = local read "Last Data \nLSI218 (1)"() -> (w2638:dbl[])
                              n1340 = local read "Last Data \nLSI218 (2)"() -> (w2639:dbl[])
                              n1341 = Build Array (concatenate)(w2641, w2642) -> (w2643:string[])
                              n1342 = Build Array (concatenate)(w2638, w2639) -> (w2640:dbl[])
                              n1343 = Search 1D Array(1D array=w2643, element=w2636) -> (index of element=w2637:i32)  [unwired: 1 in]
                              n1344 = Index Array(array=w2640, index=w2637) -> (element=w2635:dbl)
                            }
                            frame "LSI336" {
                              n1345 = local read "Last Data \nLSI336"() -> (w2647:dbl[])
                              n1346 = local read "Labels LSI336"() -> (w2646:string[])
                              n1347 = Search 1D Array(1D array=w2646, element=w2645) -> (index of element=w2648:i32)  [unwired: 1 in]
                              n1348 = Index Array(array=w2647, index=w2648) -> (element=w2644:dbl)
                            }
                            frame "DMMs" {
                              n1349 = local read "DMM LastMeasurements"() -> (w2653:dbl[])
                              n1350 = local read "DMMsLabels"() -> (w2651:string[])
                              n1351 = Search 1D Array(1D array=w2651, element=w2650) -> (index of element=w2652:i32)  [unwired: 1 in]
                              n1352 = Index Array(array=w2653, index=w2652) -> (element=w2649:dbl)
                            }
                          }
                          "I" <- w2616
                        }
                        frame #1 {
                          n1353 = Unbundle By Name("Data V") -> ("Source"=w2657:T37, "SourceLabel"=w2656:string)
                          n1354 = case shown="\"LSI218\"" w2657 {
                            tunnel: w2656 -> [w2659 w2664 w2669 w2674 w2683 w2688]
                            tunnel: [w2658 w2663 w2668 w2673 w2682 w2687] -> w2654
                            frame "USB6210", Default {
                              n1355 = local read "All Labels (USB6210)"() -> (w2661:string[])
                              n1356 = local read "Last Data \n(USB6210)"() -> (w2660:dbl[])
                              n1357 = Search 1D Array(1D array=w2661, element=w2659) -> (index of element=w2662:i32)  [unwired: 1 in]
                              n1358 = Index Array(array=w2660, index=w2662) -> (element=w2658:dbl)
                            }
                            frame "USB6218AI" {
                              n1359 = local read "All Labels (USB6218)"() -> (w2666:string[])
                              n1360 = local read "Last Data \n(USB6218)"() -> (w2665:dbl[])
                              n1361 = Search 1D Array(1D array=w2666, element=w2664) -> (index of element=w2667:i32)  [unwired: 1 in]
                              n1362 = Index Array(array=w2665, index=w2667) -> (element=w2663:dbl)
                            }
                            frame "USB6218AO" {
                              n1363 = local read "USB 6218 AOUT"() -> (w2670:dbl[])
                              n1364 = local read "AOUT Labels"() -> (w2671:string[])
                              n1365 = Search 1D Array(1D array=w2671, element=w2669) -> (index of element=w2672:i32)  [unwired: 1 in]
                              n1366 = Index Array(array=w2670, index=w2672) -> (element=w2668:dbl)
                            }
                            frame "LSI218" {
                              n1367 = local read "Labels LSI218 (1)"() -> (w2679:string[])
                              n1368 = local read "Labels LSI218 (2)"() -> (w2680:string[])
                              n1369 = local read "Last Data \nLSI218 (1)"() -> (w2676:dbl[])
                              n1370 = local read "Last Data \nLSI218 (2)"() -> (w2677:dbl[])
                              n1371 = Build Array (concatenate)(w2679, w2680) -> (w2681:string[])
                              n1372 = Build Array (concatenate)(w2676, w2677) -> (w2678:dbl[])
                              n1373 = Search 1D Array(1D array=w2681, element=w2674) -> (index of element=w2675:i32)  [unwired: 1 in]
                              n1374 = Index Array(array=w2678, index=w2675) -> (element=w2673:dbl)
                            }
                            frame "LSI336" {
                              n1375 = local read "Last Data \nLSI336"() -> (w2685:dbl[])
                              n1376 = local read "Labels LSI336"() -> (w2684:string[])
                              n1377 = Search 1D Array(1D array=w2684, element=w2683) -> (index of element=w2686:i32)  [unwired: 1 in]
                              n1378 = Index Array(array=w2685, index=w2686) -> (element=w2682:dbl)
                            }
                            frame "DMMs" {
                              n1379 = local read "DMM LastMeasurements"() -> (w2691:dbl[])
                              n1380 = local read "DMMsLabels"() -> (w2689:string[])
                              n1381 = Search 1D Array(1D array=w2689, element=w2688) -> (index of element=w2690:i32)  [unwired: 1 in]
                              n1382 = Index Array(array=w2691, index=w2690) -> (element=w2687:dbl)
                            }
                          }
                          "V" <- w2654
                        }
                        frame #2 {
                          n1383 = Unbundle By Name("Data T_low") -> ("Source"=w2695:T37, "SourceLabel"=w2694:string)
                          n1384 = case shown="\"DMMs\"" w2695 {
                            tunnel: w2694 -> [w2697 w2702 w2707 w2712 w2721 w2726]
                            tunnel: [w2696 w2701 w2706 w2711 w2720 w2725] -> w2692
                            frame "USB6210", Default {
                              n1385 = local read "All Labels (USB6210)"() -> (w2699:string[])
                              n1386 = local read "Last Data \n(USB6210)"() -> (w2698:dbl[])
                              n1387 = Search 1D Array(1D array=w2699, element=w2697) -> (index of element=w2700:i32)  [unwired: 1 in]
                              n1388 = Index Array(array=w2698, index=w2700) -> (element=w2696:dbl)
                            }
                            frame "USB6218AI" {
                              n1389 = local read "All Labels (USB6218)"() -> (w2704:string[])
                              n1390 = local read "Last Data \n(USB6218)"() -> (w2703:dbl[])
                              n1391 = Search 1D Array(1D array=w2704, element=w2702) -> (index of element=w2705:i32)  [unwired: 1 in]
                              n1392 = Index Array(array=w2703, index=w2705) -> (element=w2701:dbl)
                            }
                            frame "USB6218AO" {
                              n1393 = local read "USB 6218 AOUT"() -> (w2708:dbl[])
                              n1394 = local read "AOUT Labels"() -> (w2709:string[])
                              n1395 = Search 1D Array(1D array=w2709, element=w2707) -> (index of element=w2710:i32)  [unwired: 1 in]
                              n1396 = Index Array(array=w2708, index=w2710) -> (element=w2706:dbl)
                            }
                            frame "LSI218" {
                              n1397 = local read "Labels LSI218 (1)"() -> (w2717:string[])
                              n1398 = local read "Labels LSI218 (2)"() -> (w2718:string[])
                              n1399 = local read "Last Data \nLSI218 (1)"() -> (w2714:dbl[])
                              n1400 = local read "Last Data \nLSI218 (2)"() -> (w2715:dbl[])
                              n1401 = Build Array (concatenate)(w2717, w2718) -> (w2719:string[])
                              n1402 = Build Array (concatenate)(w2714, w2715) -> (w2716:dbl[])
                              n1403 = Search 1D Array(1D array=w2719, element=w2712) -> (index of element=w2713:i32)  [unwired: 1 in]
                              n1404 = Index Array(array=w2716, index=w2713) -> (element=w2711:dbl)
                            }
                            frame "LSI336" {
                              n1405 = local read "Last Data \nLSI336"() -> (w2723:dbl[])
                              n1406 = local read "Labels LSI336"() -> (w2722:string[])
                              n1407 = Search 1D Array(1D array=w2722, element=w2721) -> (index of element=w2724:i32)  [unwired: 1 in]
                              n1408 = Index Array(array=w2723, index=w2724) -> (element=w2720:dbl)
                            }
                            frame "DMMs" {
                              n1409 = local read "DMM LastMeasurements"() -> (w2729:dbl[])
                              n1410 = local read "DMMsLabels"() -> (w2727:string[])
                              n1411 = Search 1D Array(1D array=w2727, element=w2726) -> (index of element=w2728:i32)  [unwired: 1 in]
                              n1412 = Index Array(array=w2729, index=w2728) -> (element=w2725:dbl)
                            }
                          }
                          "T_low" <- w2692
                        }
                        frame #3 {
                          n1413 = Unbundle By Name("Data T_high") -> ("Source"=w2733:T37, "SourceLabel"=w2732:string)
                          n1414 = case shown="\"DMMs\"" w2733 {
                            tunnel: w2732 -> [w2735 w2740 w2745 w2750 w2759 w2764]
                            tunnel: [w2734 w2739 w2744 w2749 w2758 w2763] -> w2730
                            frame "USB6210", Default {
                              n1415 = local read "All Labels (USB6210)"() -> (w2737:string[])
                              n1416 = local read "Last Data \n(USB6210)"() -> (w2736:dbl[])
                              n1417 = Search 1D Array(1D array=w2737, element=w2735) -> (index of element=w2738:i32)  [unwired: 1 in]
                              n1418 = Index Array(array=w2736, index=w2738) -> (element=w2734:dbl)
                            }
                            frame "USB6218AI" {
                              n1419 = local read "All Labels (USB6218)"() -> (w2742:string[])
                              n1420 = local read "Last Data \n(USB6218)"() -> (w2741:dbl[])
                              n1421 = Search 1D Array(1D array=w2742, element=w2740) -> (index of element=w2743:i32)  [unwired: 1 in]
                              n1422 = Index Array(array=w2741, index=w2743) -> (element=w2739:dbl)
                            }
                            frame "USB6218AO" {
                              n1423 = local read "USB 6218 AOUT"() -> (w2746:dbl[])
                              n1424 = local read "AOUT Labels"() -> (w2747:string[])
                              n1425 = Search 1D Array(1D array=w2747, element=w2745) -> (index of element=w2748:i32)  [unwired: 1 in]
                              n1426 = Index Array(array=w2746, index=w2748) -> (element=w2744:dbl)
                            }
                            frame "LSI218" {
                              n1427 = local read "Labels LSI218 (1)"() -> (w2755:string[])
                              n1428 = local read "Labels LSI218 (2)"() -> (w2756:string[])
                              n1429 = local read "Last Data \nLSI218 (1)"() -> (w2752:dbl[])
                              n1430 = local read "Last Data \nLSI218 (2)"() -> (w2753:dbl[])
                              n1431 = Build Array (concatenate)(w2755, w2756) -> (w2757:string[])
                              n1432 = Build Array (concatenate)(w2752, w2753) -> (w2754:dbl[])
                              n1433 = Search 1D Array(1D array=w2757, element=w2750) -> (index of element=w2751:i32)  [unwired: 1 in]
                              n1434 = Index Array(array=w2754, index=w2751) -> (element=w2749:dbl)
                            }
                            frame "LSI336" {
                              n1435 = local read "Last Data \nLSI336"() -> (w2761:dbl[])
                              n1436 = local read "Labels LSI336"() -> (w2760:string[])
                              n1437 = Search 1D Array(1D array=w2760, element=w2759) -> (index of element=w2762:i32)  [unwired: 1 in]
                              n1438 = Index Array(array=w2761, index=w2762) -> (element=w2758:dbl)
                            }
                            frame "DMMs" {
                              n1439 = local read "DMM LastMeasurements"() -> (w2767:dbl[])
                              n1440 = local read "DMMsLabels"() -> (w2765:string[])
                              n1441 = Search 1D Array(1D array=w2765, element=w2764) -> (index of element=w2766:i32)  [unwired: 1 in]
                              n1442 = Index Array(array=w2767, index=w2766) -> (element=w2763:dbl)
                            }
                          }
                          "T_high" <- w2730
                        }
                      }
                      n1443 = local read "File Refnum (CHF)"() -> (w2596:refnum<file>)
                      n1444 = Get Date/Time In Seconds() -> (seconds since 1Jan1904=w2600:timestamp)
                      n1445 = Subtract(x=w2609, y=w2608) -> (x-y=w2604:dbl)
                      "ƒ¢T" <- w2604
                      n1446 = Multiply(x=w2611, y=w2610) -> (x*y=w2607:dbl)
                      "Q" <- w2607
                      n1447 = local read "ƒ¢T_array"() -> (w2598:dbl[])
                      n1448 = local read "Q_array"() -> (w2597:dbl[])
                      n1449 = call "FileWrite.vi"("DataArray"=w2602, "Time Stamp"=w2600, "Error In"=errorcluster {"status"=FALSE, "code"=0, "source"=""}, "FileFormat"=w2613, "Index"=w2605, "refnum in"=w2596) -> ("Error Out"=→"Error out (CHF rec)":errorcluster)  [unwired: 4 in, 1 out]
                      n1450 = Build Array (concatenate)(w2598, w2604) -> (w2603:dbl[])
                      n1451 = Build Array (concatenate)(w2597, w2607) -> (w2606:dbl[])
                    }
                  }
                  n1452 = Build Array (concatenate)(w2580, w2576) -> (w2574:dbl[][])
                  n1453 = Build Array (concatenate)(w2578, w2579) -> (w2573:timestamp[])
                  n1454 = Bundle(w2571, w2572) -> (→"Graph CHF":cluster{dbl[], dbl[]})  [unwired: 1 in]
                  n1455 = local write "ƒ¢T_array"(w2571) -> ()
                  n1456 = local write "Q_array"(w2572) -> ()
                  n1457 = Array Size(array=w2576) -> (size(s)=w2575:i32)
                  n1458 = for {
                    N: w2575 -> [_]
                    tunnel: w2574 -> [w2588]
                    tunnel: w2573 -> [w2586]
                    tunnel: [w2584] -> w2569 mode=indexing
                    i -> [w2587]
                    n1459 = Index Array(array=w2588, index (col)=w2587) -> (element=w2585:dbl[])  [unwired: 1 in]
                    n1460 = Bundle(w2586, w2585) -> (w2584:cluster{timestamp[], dbl[]})  [unwired: 1 in]
                  }
                  "Graph CHF log 2" <- w2569
                  "Graph CHF log 1" <- w2569
                  "Graph CHF log 3" <- w2569
                }
                frame True {
                }
              }
            }
          }
          frame #2 {
            n1461 = local write "CHF measurement counter"(0 ("CHF counter")) -> ()
            n1462 = local write "START CHF"(FALSE ("START CHF")) -> ()
            n1463 = local write "STOP CHF"(FALSE ("STOP CHF")) -> ()
          }
        }
      }
    }
    n1464 = case shown="False" "REFRESH GRAPH" {
      frame False {
      }
      frame True {
        n1465 = stacked-sequence {
          frame #0 {
            w2480 = dbl[] [] ("ƒ¢T_array")
            n1466 = local write "ƒ¢T_array"(w2480) -> ()
            n1467 = local write "Q_array"(w2480) -> ()
            n1468 = Bundle("ƒ¢T_array"=w2480, "ƒ¢T_array"=w2480) -> (w2479:cluster{"ƒ¢T_array":dbl[], "ƒ¢T_array":dbl[]})  [unwired: 1 in]
            n1469 = local write "Graph CHF"(w2479) -> ()
          }
          frame #1 {
            n1470 = local write "REFRESH GRAPH"(FALSE ("REFRESH GRAPH")) -> ()
          }
        }
      }
    }
    n1471 = Get Notifier Status(notifier=w2425, error in (no error)=w2424) -> (current notification=w2426:bool)  [unwired: 4 out]
  }
  n1472 = while {
    shift-right: [w2821] -> w8
    shift-left: refnum<class "DMMsData.lvclass"> refnum ("DMMsData.lvclass") -> [w2820]
    shift-right: [w2819] -> w7
    shift-left: errorcluster {"status"=FALSE, "code"=0, "source"=""} ("error in (no error)") -> [w2812]
    tunnel: w5 -> [w2817]
    tunnel: w4 -> [w2816]
    tunnel: [w2815] -> w11
    i -> [w2818]
    stop <- w2814 stop-if-true
    n1473 = Equal?(x=w2818, y=0) -> (x = y?=w2822:bool)
    n1474 = Wait (ms)(milliseconds to wait="Measurement Interval DMMs (ms)") -> ()  [unwired: 1 out]
    n1475 = case shown="False" "Measure DMMs?" {
      tunnel: w2822 -> [_ w2833]
      tunnel: [w2826 w2831] -> w2821
      tunnel: w2820 -> [w2826 w2830]
      tunnel: w2812 -> [w2825 w2829]
      tunnel: [w2825 w2828] -> w2819
      tunnel: w2818 -> [_ w2827]
      frame False {
      }
      frame True {
        n1476 = Or(x="Initialize (DMMs)", y=w2833) -> (x .or. y?=w2832:bool)
        n1477 = case shown="False" w2832 {
          tunnel: w2830 -> [w2864 w2900]
          tunnel: [w2861 w2899] -> w2831
          tunnel: w2829 -> [w2863 w2896]
          tunnel: [w2862 w2893] -> w2828
          tunnel: w2827 -> [w2860 _]
          frame False {
            n1478 = local read "VariableSources"() -> (w2853:T12)
            n1479 = for {
              tunnel: w2853 -> [w2867] mode=indexing
              tunnel: [w2866] -> w2852 mode=indexing
              tunnel: [w2865] -> w2851 mode=indexing
              n1480 = case shown="\"LSI218\"" w2867 {
                tunnel: [w2869 w2871 w2873 w2874 w2880] -> w2866
                tunnel: [w2868 w2870 w2872 w2875 w2881] -> w2865
                frame "USB6210" {
                  n1481 = local read "All Labels (USB6210)"() -> (w2869:string[])
                  n1482 = local read "Last Data \n(USB6210)"() -> (w2868:dbl[])
                }
                frame "USB6218AI" {
                  n1483 = local read "Last Data \n(USB6218)"() -> (w2870:dbl[])
                  n1484 = local read "All Labels (USB6218)"() -> (w2871:string[])
                }
                frame "USB6218AO" {
                  n1485 = local read "USB 6218 AOUT"() -> (w2872:dbl[])
                  n1486 = local read "AOUT Labels"() -> (w2873:string[])
                }
                frame "LSI218" {
                  n1487 = local read "Last Data \nLSI218 (2)"() -> (w2876:dbl[])
                  n1488 = local read "Last Data \nLSI218 (1)"() -> (w2877:dbl[])
                  n1489 = local read "Labels LSI218 (2)"() -> (w2879:string[])
                  n1490 = local read "Labels LSI218 (1)"() -> (w2878:string[])
                  n1491 = Build Array (concatenate)(w2877, w2876) -> (w2875:dbl[])
                  n1492 = Build Array (concatenate)(w2878, w2879) -> (w2874:string[])
                }
                frame "LSI336" {
                  n1493 = local read "Last Data \nLSI336"() -> (w2881:dbl[])
                  n1494 = local read "Labels LSI336"() -> (w2880:string[])
                }
              }
            }
            n1495 = local read "DMMsConfig (variables)"() -> (w2845:T13)
            n1496 = local read "DMMsConfig"() -> (w2857:T11)
            n1497 = call-dynamic "DMMs_measure.vi"("DMMsData in"=w2864, "Sample #"="Sample #", "MeasurementIndex"=w2860, "SourceDataLabels"=w2852, "error in (no error)"=w2863, "SourceDataArray"=w2851) -> ("TimeArray"=w2859:timestamp[], "DMMsData out"=w2861:refnum<class "DMMsData.lvclass">, "LastData"=w2839:dbl[], "DataArray"=w2856:dbl[][], "DeviceActive?"=→"Active?":bool[], "error out"=w2862:errorcluster)  [unwired: 4 in]
            "DMM LastMeasurements" <- w2839
            n1498 = Array Size(array=w2845) -> (size(s)=w2843:i32)
            n1499 = Array Size(array=w2857) -> (size(s)=w2844:i32)
            n1500 = Add(x=w2844, y=w2843) -> (x+y=w2842:i32)
            n1501 = for {
              N: w2842 -> [_]
              tunnel: w2859 -> [w2884]
              tunnel: w2856 -> [w2888]
              shift-right: [w2882] -> w2841
              shift-left: T4 [] -> [w2883]
              i -> [w2887]
              n1502 = Index Array(array=w2888, index (col)=w2887) -> (element=w2886:dbl[])  [unwired: 1 in]
              n1503 = Bundle("TimeArray"=w2884, "DataArray"=w2886) -> (w2885:T36)  [unwired: 1 in]
              n1504 = Build Array (concatenate)(w2883, w2885) -> (w2882:T4)
            }
            "Graph DMMs 2" <- w2841
            "Graph DMMs 1" <- w2841
            "Graph DMMs 3" <- w2841
            n1505 = Index Array(array=w2839, index #1="index T_2", index #2="index T_ 1") -> (element #1=w2838:dbl, element #2=w2835:dbl)
            n1506 = Index Array(array=w2839, index #1="index V", index #2="index I") -> (element #1=w2848:dbl, element #2=w2847:dbl)
            n1507 = Subtract(x=w2838, y=w2835) -> (x-y=→"ƒ¢T=T_2 -T_1":dbl)
            n1508 = Multiply(x=w2848, y=w2847) -> (x*y=→"Q = I *V":dbl)
          }
          frame True {
            n1509 = local write "Initialize (DMMs)"(FALSE ("Initialize 2")) -> ()
            n1510 = local read "RUN Identifier"() -> (w2892:string)
            n1511 = local read "Base Path"() -> (w2897:path)
            n1512 = call-dynamic "DMMs_initialize.vi"("DMMsConfig (variables)"="DMMsConfig (variables)", "DMMsConfig"="DMMsConfig", "InstName"="InstName DMMs", "error in (no error)"=w2896, "base path"=w2897, "RunIdentifier"=w2892, "DMMsData in"=w2900) -> ("error out"=w2893:errorcluster, "DMMsLabels"=w2894:string[], "FileName"=→"DMMFileName":string, "DMMsData out"=w2899:refnum<class "DMMsData.lvclass">, "VariableSources"=→"VariableSources":T12)
            "DMMsLabels" <- w2894
            n1513 = stacked-sequence {
              tunnel: w2894 -> [w2902 w2925 w2948]
              frame #0 {
                n1514 = Array Size(array=w2902) -> (size(s)=w2911:i32)
                n1515 = control-ref of="Graph DMMs 1"() -> (w2908:refnum<vi>)
                n1516 = property class="XYGraph (strict)"(reference=w2908, error in=errorcluster {"status"=FALSE, "code"=0, "source"=""} ("error in (no error)")) -> (reference out=w2904:refnum<vi>, error out=w2907:errorcluster, "LegNumRows"=w2909:u32)
                n1517 = for {
                  N: w2909 -> [_]
                  shift-right: [w2920] -> w2910
                  shift-left: w2907 -> [w2921]
                  tunnel: w2904 -> [w2919]
                  tunnel: [w2918] -> w2903 mode=indexing
                  i -> [w2923]
                  n1518 = property class="XYGraph (strict)"(reference=w2919, error in=w2921, "Active Plot"=w2923, "Plot.Plot Name"="") -> (reference out=w2918:refnum<vi>, error out=w2920:errorcluster)
                }
                n1519 = for {
                  N: w2911 -> [_]
                  shift-right: [w2915] -> w2905
                  shift-left: w2910 -> [w2916]
                  tunnel: w2903 -> [w2913] mode=indexing
                  tunnel: w2902 -> [w2912] mode=indexing
                  i -> [w2917]
                  n1520 = property class="XYGraph (strict)"(reference=w2913, error in=w2916, "Active Plot"=w2917, "Plot.Plot Name"=w2912, "Plot.Visible?"=TRUE ("Plot.Visible")) -> (error out=w2915:errorcluster)  [unwired: 1 out]
                }
                "error out (DMM graphs)" <- w2905
              }
              frame #1 {
                n1521 = Array Size(array=w2925) -> (size(s)=w2933:i32)
                n1522 = control-ref of="Graph DMMs 2"() -> (w2928:refnum<vi>)
                n1523 = property class="XYGraph (strict)"(reference=w2928, error in=errorcluster {"status"=FALSE, "code"=0, "source"=""} ("error in (no error)")) -> (reference out=w2927:refnum<vi>, error out=w2930:errorcluster, "LegNumRows"=w2931:u32)
                n1524 = for {
                  N: w2931 -> [_]
                  shift-right: [w2942] -> w2932
                  shift-left: w2930 -> [w2943]
                  tunnel: w2927 -> [w2941]
                  tunnel: [w2940] -> w2926 mode=indexing
                  i -> [w2945]
                  n1525 = property class="XYGraph (strict)"(reference=w2941, error in=w2943, "Active Plot"=w2945, "Plot.Plot Name"="") -> (reference out=w2940:refnum<vi>, error out=w2942:errorcluster)
                }
                n1526 = for {
                  N: w2933 -> [_]
                  shift-right: [w2937] -> w2924
                  shift-left: w2932 -> [w2938]
                  tunnel: w2926 -> [w2935] mode=indexing
                  tunnel: w2925 -> [w2934] mode=indexing
                  i -> [w2939]
                  n1527 = property class="XYGraph (strict)"(reference=w2935, error in=w2938, "Active Plot"=w2939, "Plot.Plot Name"=w2934, "Plot.Visible?"=TRUE ("Plot.Visible")) -> (error out=w2937:errorcluster)  [unwired: 1 out]
                }
                n1528 = local write "error out (DMM graphs)"(w2924) -> ()
              }
              frame #2 {
                n1529 = Array Size(array=w2948) -> (size(s)=w2955:i32)
                n1530 = control-ref of="Graph DMMs 3"() -> (w2946:refnum<vi>)
                n1531 = property class="XYGraph (strict)"(reference=w2946, error in=errorcluster {"status"=FALSE, "code"=0, "source"=""} ("error in (no error)")) -> (reference out=w2950:refnum<vi>, error out=w2952:errorcluster, "LegNumRows"=w2953:u32)
                n1532 = for {
                  N: w2953 -> [_]
                  shift-right: [w2964] -> w2954
                  shift-left: w2952 -> [w2965]
                  tunnel: w2950 -> [w2963]
                  tunnel: [w2962] -> w2949 mode=indexing
                  i -> [w2967]
                  n1533 = property class="XYGraph (strict)"(reference=w2963, error in=w2965, "Active Plot"=w2967, "Plot.Plot Name"="") -> (reference out=w2962:refnum<vi>, error out=w2964:errorcluster)
                }
                n1534 = for {
                  N: w2955 -> [_]
                  shift-right: [w2959] -> w2947
                  shift-left: w2954 -> [w2960]
                  tunnel: w2949 -> [w2957] mode=indexing
                  tunnel: w2948 -> [w2956] mode=indexing
                  i -> [w2961]
                  n1535 = property class="XYGraph (strict)"(reference=w2957, error in=w2960, "Active Plot"=w2961, "Plot.Plot Name"=w2956, "Plot.Visible?"=TRUE ("Plot.Visible")) -> (error out=w2959:errorcluster)  [unwired: 1 out]
                }
                n1536 = local write "error out (DMM graphs)"(w2947) -> ()
              }
            }
          }
        }
        "error out (DMMs)" <- w2828
      }
    }
    n1537 = Get Notifier Status(notifier=w2817, error in (no error)=w2816) -> (current notification=w2814:bool, error out=w2815:errorcluster)  [unwired: 3 out]
    "cycle # (DMMs)" <- w2818
  }
  n1538 = call-dynamic "USBData_terminate.vi"("error in (no error)"=w24, "USBData in"=w25) -> ("error out"=w26:errorcluster)  [unwired: 8 in, 1 out]
  n1539 = local write "error out (USB6210)"(w26) -> ()
  n1540 = call-dynamic "DMMs_terminate.vi"("error in (no error)"=w7, "DMMsData in"=w8) -> ("error out"=→"error out (DMMs) 2":errorcluster)  [unwired: 8 in, 1 out]
  n1541 = call-dynamic "USBData_terminate.vi"("error in (no error)"=w39, "USBData in"=w40) -> ("error out"=w41:errorcluster)  [unwired: 8 in, 1 out]
  n1542 = call-dynamic "LSI336Data_terminate.vi"("error in (no error)"=w30, "LSI336Data in"=w31) -> ("error out"=w29:errorcluster)  [unwired: 8 in, 1 out]
  n1543 = Merge Errors(w11, w13) -> (w14:errorcluster)
  n1544 = local write "error out (USB6210)"(w41) -> ()
  n1545 = local write "error out (LSI336)"(w29) -> ()
  n1546 = call "LSI218Data_terminate.vi"("error in (no error)"=w34, "LSI218Data in"=w35) -> ("error out"=w33:errorcluster)  [unwired: 8 in, 1 out]
  n1547 = Release Notifier(notifier=w12, error in (no error)=w14) -> (error out=→"error out (notifier)":errorcluster)  [unwired: 1 in, 2 out]
  n1548 = local write "error out (LSI218)"(w33) -> ()
